vi "LCM_data_assign_tmp.vi"(9 "time-to-live":u16, 10 "Velodyne1":T3(ring), 11 "velodyne enable":bool) -> ()   [LabVIEW 2015]
uses:
  G_LCM.vi
  G_ALL.vi
  G_SEN.vi
  <vilib>/Instr/_visa.llb/VISA Configure Serial Port (Instr).vi
panel:
  out "mission_request":T1
  out "error out 3":errorcluster
  out "velodyne overflow? 2":bool
  out "VELO_RAW":T2={"hash"=6418264790525055119, "sys time"=0, "type"=0, "raw"=""} {"hash" format="%x"}
  out "ibeo overflow?":bool
  out "veodyne error out":errorcluster
  out "control input":T4
  in  "saveconfig":bool
  in  "get data":bool
  in  "parameter idx 2":u16 format="%x"
  in  "setdata":bool
  in  "Mouting":u32 format="%x"
  in  "parameter idx":u16 format="%x"
  out "LCM error":errorcluster
  out "error out":errorcluster
  out "SDT_GPS_DATA":T5
  out "PATH_T":T6
  out "length":i32
  out "ALT_T":T7={"hash"=-8920902524919788889, "sys time"=0, "u time"=0, "alt"=0.0} {"hash" format="%016x"}
  out "value":cluster{"time":i32, "alt":sgl}
  out "data":dbl[][](array[numeric]) format="%#_17g"
  out "Waveform Graph":dbl[](graph)
  out "IBEO_2202_T":T8={"hash"=-9184050406206942030, "sys time"=0, "Header"={"Size of prev messages"=0, "Size of this messages"=8534, "Reserved"=0, "DeviceID"=0, "Data type"=8706, "NTP time"=30358766255088}, "Scan header"={"Scan number"=22632, "scanner status"=811, "Sync phase offset"=0, "Scan start time NTP"=30358508796168, "Scan end time NTP"=30358603880928, "Angle ticks per rotation"=11520, "Start angle"=0.8726646259971648, "End angle"=-0.8726646259971648, "Scan points"=849, "pos_x"=0.0, "pos_y"=0.0, "pos_h"=0.0, "Mounting position x"=3.5, "Mounting position y"=0.0, "Mounting position z"=0.45, "Reserved"=5}, "Scan points"=[{"flags"=0, "Echo"=0, "Radial distance"=20.2, "Horizontal angle"=0.8552113334772213, "Vertical angle"=-0.020943951023931952, "Echo pulse width"=92, "Reserved"=0}, {"flags"=0, "Echo"=0, "Radial distance"=20.05, "Horizontal angle"=0.8552113334772213, "Vertical angle"=-0.006981317007977317, "Echo pulse width"=48, "Reserved"=0}, {"flags"=0, "Echo"=0, "Radial distance"=20.21, "Horizontal angle"=0.8464846872172498, "Vertical angle"=-0.020943951023931952, "Echo pulse width"=80, "Reserved"=0}, {"flags"=0, "Echo"=0, "Radial distance"=20.03, "Horizontal angle"=0.8464846872172498, "Vertical angle"=-0.006981317007977317, "Echo pulse width"=120, "Reserved"=0}, {"flags"=0, "Echo"=0, "Radial distance"=20.400000000000002, "Horizontal angle"=0.8377580409572781, "Vertical angle"=-0.020943951023931952, "Echo pulse width"=136, "Reserved"=0}, {"flags"=0, "Echo"=0, "Radial distance"=20.080000000000002, "Horizontal angle"=0.8377580409572781, "Vertical angle"=-0.006981317007977317, "Echo pulse width"=132, "Reserved"=0}, {"flags"=0, "Echo"=0, "Radial distance"=20.67, "Horizontal angle"=0.8290313946973066, "Vertical angle"=-0.020943951023931952, "Echo pulse width"=124, "Reserved"=0}, {"flags"=0, "Echo"=0, "Radial distance"=20.37, "Horizontal angle"=0.8290313946973066, "Vertical angle"=-0.006981317007977317, "Echo pulse width"=144, "Reserved"=0}, {"flags"=5, "Echo"=0, "Radial distance"=20.830000000000002, "Horizontal angle"=0.8203047484373349, "Vertical angle"=-0.020943951023931952, "Echo pulse width"=72, "Reserved"=0}, {"flags"=4, "Echo"=1, "Radial distance"=21.87, "Horizontal angle"=0.8203047484373349, "Vertical angle"=-0.020943951023931952, "Echo pulse width"=124, "Reserved"=0}, {"flags"=4, "Echo"=0, "Radial distance"=21.88, "Horizontal angle"=0.8115781021773633, "Vertical angle"=-0.020943951023931952, "Echo pulse width"=132, "Reserved"=0}, {"flags"=4, "Echo"=0, "Radial distance"=21.78, "Horizontal angle"=0.8028514559173915, "Vertical angle"=-0.020943951023931952, "Echo pulse width"=156, "Reserved"=0}, {"flags"=4, "Echo"=0, "Radial distance"=21.76, "Horizontal angle"=0.7941248096574199, "Vertical angle"=-0.020943951023931952, "Echo pulse width"=176, "Reserved"=0}, {"flags"=1, "Echo"=0, "Radial distance"=23.37, "Horizontal angle"=0.7941248096574199, "Vertical angle"=-0.006981317007977317, "Echo pulse width"=100, "Reserved"=1}, {"flags"=0, "Echo"=1, "Radial distance"=48.230000000000004, "Horizontal angle"=0.7941248096574199, "Vertical angle"=-0.006981317007977317, "Echo pulse width"=120, "Reserved"=2}, {"flags"=4, "Echo"=0, "Radial distance"=21.76, "Horizontal angle"=0.7853981633974483, "Vertical angle"=-0.020943951023931952, "Echo pulse width"=172, "Reserved"=0}, {"flags"=1, "Echo"=0, "Radial distance"=23.25, "Horizontal angle"=0.7853981633974483, "Vertical angle"=-0.006981317007977317, "Echo pulse width"=144, "Reserved"=1}, {"flags"=0, "Echo"=1, "Radial distance"=48.02, "Horizontal angle"=0.7853981633974483, "Vertical angle"=-0.006981317007977317, "Echo pulse width"=108, "Reserved"=2}, {"flags"=0, "Echo"=0, "Radial distance"=16.740000000000002, "Horizontal angle"=0.7766715171374766, "Vertical angle"=-0.020943951023931952, "Echo pulse width"=156, "Reserved"=3}, {"flags"=0, "Echo"=0, "Radial distance"=16.77, "Horizontal angle"=0.7766715171374766, "Vertical angle"=-0.006981317007977317, "Echo pulse width"=152, "Reserved"=3}, {"flags"=5, "Echo"=0, "Radial distance"=5.44, "Horizontal angle"=0.767944870877505, "Vertical angle"=-0.020943951023931952, "Echo pulse width"=136, "Reserved"=0}, {"flags"=4, "Echo"=1, "Radial distance"=21.87, "Horizontal angle"=0.767944870877505, "Vertical angle"=-0.020943951023931952, "Echo pulse width"=164, "Reserved"=0}, {"flags"=1, "Echo"=0, "Radial distance"=23.17, "Horizontal angle"=0.767944870877505, "Vertical angle"=-0.006981317007977317, "Echo pulse width"=148, "Reserved"=1}, {"flags"=0, "Echo"=1, "Radial distance"=48.18, "Horizontal angle"=0.767944870877505, "Vertical angle"=-0.006981317007977317, "Echo pulse width"=108, "Reserved"=4}, {"flags"=4, "Echo"=0, "Radial distance"=22.03, "Horizontal angle"=0.7592182246175333, "Vertical angle"=-0.020943951023931952, "Echo pulse width"=164, "Reserved"=0}, {"flags"=0, "Echo"=0, "Radial distance"=23.3, "Horizontal angle"=0.7592182246175333, "Vertical angle"=-0.006981317007977317, "Echo pulse width"=168, "Reserved"=1}, {"flags"=5, "Echo"=0, "Radial distance"=5.21, "Horizontal angle"=0.7504915783575618, "Vertical angle"=-0.020943951023931952, "Echo pulse width"=144, "Reserved"=0}, {"flags"=4, "Echo"=1, "Radial distance"=22.27, "Horizontal angle"=0.7504915783575618, "Vertical angle"=-0.020943951023931952, "Echo pulse width"=164, "Reserved"=0}, {"flags"=0, "Echo"=0, "Radial distance"=23.34, "Horizontal angle"=0.7504915783575618, "Vertical angle"=-0.006981317007977317, "Echo pulse width"=172, "Reserved"=1}, {"flags"=5, "Echo"=0, "Radial distance"=20.36, "Horizontal angle"=0.74176493209759, "Vertical angle"=-0.020943951023931952, "Echo pulse width"=68, "Reserved"=0}, {"flags"=4, "Echo"=1, "Radial distance"=22.42, "Horizontal angle"=0.74176493209759, "Vertical angle"=-0.020943951023931952, "Echo pulse width"=152, "Reserved"=0}, {"flags"=0, "Echo"=0, "Radial distance"=23.38, "Horizontal angle"=0.74176493209759, "Vertical angle"=-0.006981317007977317, "Echo pulse width"=168, "Reserved"=1}, {"flags"=5, "Echo"=0, "Radial distance"=5.5600000000000005, "Horizontal angle"=0.7330382858376184, "Vertical angle"=-0.020943951023931952, "Echo pulse width"=168, "Reserved"=0}, {"flags"=4, "Echo"=1, "Radial distance"=22.62, "Horizontal angle"=0.7330382858376184, "Vertical angle"=-0.020943951023931952, "Echo pulse width"=152, "Reserved"=0}, {"flags"=1, "Echo"=0, "Radial distance"=23.37, "Horizontal angle"=0.7330382858376184, "Vertical angle"=-0.006981317007977317, "Echo pulse width"=156, "Reserved"=1}, {"flags"=0, "Echo"=1, "Radial distance"=48.21, "Horizontal angle"=0.7330382858376184, "Vertical angle"=-0.006981317007977317, "Echo pulse width"=72, "Reserved"=5}, {"flags"=5, "Echo"=0, "Radial distance"=5.58, "Horizontal angle"=0.7243116395776468, "Vertical angle"=-0.020943951023931952, "Echo pulse width"=136, "Reserved"=0}, {"flags"=5, "Echo"=1, "Radial distance"=20.88, "Horizontal angle"=0.7243116395776468, "Vertical angle"=-0.020943951023931952, "Echo pulse width"=64, "Reserved"=0}, {"flags"=4, "Echo"=2, "Radial distance"=22.77, "Horizontal angle"=0.7243116395776468, "Vertical angle"=-0.020943951023931952, "Echo pulse width"=148, "Reserved"=0}, {"flags"=0, "Echo"=0, "Radial distance"=23.62, "Horizontal angle"=0.7243116395776468, "Vertical angle"=-0.006981317007977317, "Echo pulse width"=172, "Reserved"=1}, {"flags"=5, "Echo"=0, "Radial distance"=5.63, "Horizontal angle"=0.7155849933176751, "Vertical angle"=-0.020943951023931952, "Echo pulse width"=196, "Reserved"=0}, {"flags"=4, "Echo"=1, "Radial distance"=22.69, "Horizontal angle"=0.7155849933176751, "Vertical angle"=-0.020943951023931952, "Echo pulse width"=212, "Reserved"=0}, {"flags"=0, "Echo"=0, "Radial distance"=23.82, "Horizontal angle"=0.7155849933176751, "Vertical angle"=-0.006981317007977317, "Echo pulse width"=160, "Reserved"=1}, {"flags"=5, "Echo"=0, "Radial distance"=5.67, "Horizontal angle"=0.7068583470577035, "Vertical angle"=-0.020943951023931952, "Echo pulse width"=172, "Reserved"=0}, {"flags"=4, "Echo"=1, "Radial distance"=23.16, "Horizontal angle"=0.7068583470577035, "Vertical angle"=-0.020943951023931952, "Echo pulse width"=176, "Reserved"=0}, {"flags"=0, "Echo"=0, "Radial distance"=23.62, "Horizontal angle"=0.7068583470577035, "Vertical angle"=-0.006981317007977317, "Echo pulse width"=164, "Reserved"=1}, {"flags"=5, "Echo"=0, "Radial distance"=5.53, "Horizontal angle"=0.6981317007977318, "Vertical angle"=-0.020943951023931952, "Echo pulse width"=208, "Reserved"=0}, {"flags"=0, "Echo"=1, "Radial distance"=23.35, "Horizontal angle"=0.6981317007977318, "Vertical angle"=-0.020943951023931952, "Echo pulse width"=160, "Reserved"=1}, {"flags"=0, "Echo"=0, "Radial distance"=23.650000000000002, "Horizontal angle"=0.6981317007977318, "Vertical angle"=-0.006981317007977317, "Echo pulse width"=148, "Reserved"=1}, {"flags"=5, "Echo"=0, "Radial distance"=5.55, "Horizontal angle"=0.6894050545377601, "Vertical angle"=-0.020943951023931952, "Echo pulse width"=192, "Reserved"=0}, {"flags"=0, "Echo"=1, "Radial distance"=23.55, "Horizontal angle"=0.6894050545377601, "Vertical angle"=-0.020943951023931952, "Echo pulse width"=160, "Reserved"=1}, {"flags"=0, "Echo"=0, "Radial distance"=23.62, "Horizontal angle"=0.6894050545377601, "Vertical angle"=-0.006981317007977317, "Echo pulse width"=160, "Reserved"=1}, {"flags"=5, "Echo"=0, "Radial distance"=5.5600000000000005, "Horizontal angle"=0.6806784082777886, "Vertical angle"=-0.020943951023931952, "Echo pulse width"=236, "Reserved"=0}, {"flags"=0, "Echo"=1, "Radial distance"=23.77, "Horizontal angle"=0.6806784082777886, "Vertical angle"=-0.020943951023931952, "Echo pulse width"=144, "Reserved"=1}, {"flags"=0, "Echo"=0, "Radial distance"=23.61, "Horizontal angle"=0.6806784082777886, "Vertical angle"=-0.006981317007977317, "Echo pulse width"=156, "Reserved"=1}, {"flags"=5, "Echo"=0, "Radial distance"=5.5200000000000005, "Horizontal angle"=0.6719517620178168, "Vertical angle"=-0.020943951023931952, "Echo pulse width"=220, "Reserved"=0}, {"flags"=4, "Echo"=1, "Radial distance"=24.17, "Horizontal angle"=0.6719517620178168, "Vertical angle"=-0.020943951023931952, "Echo pulse width"=148, "Reserved"=0}, {"flags"=0, "Echo"=0, "Radial distance"=23.66, "Horizontal angle"=0.6719517620178168, "Vertical angle"=-0.006981317007977317, "Echo pulse width"=164, "Reserved"=1}, {"flags"=5, "Echo"=0, "Radial distance"=5.67, "Horizontal angle"=0.6632251157578453, "Vertical angle"=-0.020943951023931952, "Echo pulse width"=224, "Reserved"=0}, {"flags"=4, "Echo"=1, "Radial distance"=24.45, "Horizontal angle"=0.6632251157578453, "Vertical angle"=-0.020943951023931952, "Echo pulse width"=148, "Reserved"=0}, {"flags"=1, "Echo"=0, "Radial distance"=32.230000000000004, "Horizontal angle"=0.6632251157578453, "Vertical angle"=-0.006981317007977317, "Echo pulse width"=40, "Reserved"=6}, {"flags"=0, "Echo"=1, "Radial distance"=35.42, "Horizontal angle"=0.6632251157578453, "Vertical angle"=-0.006981317007977317, "Echo pulse width"=164, "Reserved"=7}, {"flags"=5, "Echo"=0, "Radial distance"=5.63, "Horizontal angle"=0.6544984694978736, "Vertical angle"=-0.020943951023931952, "Echo pulse width"=208, "Reserved"=0}, {"flags"=4, "Echo"=1, "Radial distance"=24.73, "Horizontal angle"=0.6544984694978736, "Vertical angle"=-0.020943951023931952, "Echo pulse width"=144, "Reserved"=0}, {"flags"=0, "Echo"=0, "Radial distance"=35.14, "Horizontal angle"=0.6544984694978736, "Vertical angle"=-0.006981317007977317, "Echo pulse width"=164, "Reserved"=7}, {"flags"=5, "Echo"=0, "Radial distance"=5.64, "Horizontal angle"=0.6457718232379019, "Vertical angle"=-0.020943951023931952, "Echo pulse width"=244, "Reserved"=0}, {"flags"=4, "Echo"=1, "Radial distance"=25.04, "Horizontal angle"=0.6457718232379019, "Vertical angle"=-0.020943951023931952, "Echo pulse width"=132, "Reserved"=0}, {"flags"=0, "Echo"=0, "Radial distance"=35.01, "Horizontal angle"=0.6457718232379019, "Vertical angle"=-0.006981317007977317, "Echo pulse width"=156, "Reserved"=7}, {"flags"=5, "Echo"=0, "Radial distance"=5.71, "Horizontal angle"=0.6370451769779303, "Vertical angle"=-0.020943951023931952, "Echo pulse width"=264, "Reserved"=0}, {"flags"=4, "Echo"=1, "Radial distance"=25.6, "Horizontal angle"=0.6370451769779303, "Vertical angle"=-0.020943951023931952, "Echo pulse width"=132, "Reserved"=0}, {"flags"=1, "Echo"=0, "Radial distance"=32.68, "Horizontal angle"=0.6370451769779303, "Vertical angle"=-0.006981317007977317, "Echo pulse width"=56, "Reserved"=8}, {"flags"=0, "Echo"=1, "Radial distance"=34.86, "Horizontal angle"=0.6370451769779303, "Vertical angle"=-0.006981317007977317, "Echo pulse width"=160, "Reserved"=7}, {"flags"=5, "Echo"=0, "Radial distance"=5.63, "Horizontal angle"=0.6283185307179586, "Vertical angle"=-0.020943951023931952, "Echo pulse width"=296, "Reserved"=0}, {"flags"=4, "Echo"=1, "Radial distance"=25.84, "Horizontal angle"=0.6283185307179586, "Vertical angle"=-0.020943951023931952, "Echo pulse width"=92, "Reserved"=0}, {"flags"=5, "Echo"=0, "Radial distance"=7.54, "Horizontal angle"=0.6283185307179586, "Vertical angle"=-0.006981317007977317, "Echo pulse width"=168, "Reserved"=0}, {"flags"=0, "Echo"=1, "Radial distance"=34.87, "Horizontal angle"=0.6283185307179586, "Vertical angle"=-0.006981317007977317, "Echo pulse width"=124, "Reserved"=7}, {"flags"=4, "Echo"=0, "Radial distance"=5.67, "Horizontal angle"=0.619591884457987, "Vertical angle"=-0.020943951023931952, "Echo pulse width"=272, "Reserved"=0}, {"flags"=4, "Echo"=0, "Radial distance"=7.38, "Horizontal angle"=0.619591884457987, "Vertical angle"=-0.006981317007977317, "Echo pulse width"=204, "Reserved"=0}, {"flags"=4, "Echo"=0, "Radial distance"=5.67, "Horizontal angle"=0.6108652381980153, "Vertical angle"=-0.020943951023931952, "Echo pulse width"=284, "Reserved"=0}, {"flags"=0, "Echo"=0, "Radial distance"=7.33, "Horizontal angle"=0.6108652381980153, "Vertical angle"=-0.006981317007977317, "Echo pulse width"=224, "Reserved"=9}, {"flags"=0, "Echo"=0, "Radial distance"=7.21, "Horizontal angle"=0.6065019150680295, "Vertical angle"=0.00698131700797732, "Echo pulse width"=124, "Reserved"=9}, {"flags"=0, "Echo"=0, "Radial distance"=7.08, "Horizontal angle"=0.6065019150680295, "Vertical angle"=0.020943951023931963, "Echo pulse width"=120, "Reserved"=9}, {"flags"=4, "Echo"=0, "Radial distance"=5.79, "Horizontal angle"=0.6021385919380438, "Vertical angle"=-0.020943951023931952, "Echo pulse width"=248, "Reserved"=0}, {"flags"=0, "Echo"=0, "Radial distance"=7.09, "Horizontal angle"=0.6021385919380438, "Vertical angle"=-0.006981317007977317, "Echo pulse width"=232, "Reserved"=9}, {"flags"=0, "Echo"=0, "Radial distance"=7.24, "Horizontal angle"=0.5977752688080579, "Vertical angle"=0.00698131700797732, "Echo pulse width"=72, "Reserved"=9}, {"flags"=0, "Echo"=0, "Radial distance"=6.99, "Horizontal angle"=0.5977752688080579, "Vertical angle"=0.020943951023931963, "Echo pulse width"=60, "Reserved"=9}, {"flags"=4, "Echo"=0, "Radial distance"=5.75, "Horizontal angle"=0.593411945678072, "Vertical angle"=-0.020943951023931952, "Echo pulse width"=268, "Reserved"=0}, {"flags"=0, "Echo"=0, "Radial distance"=6.84, "Horizontal angle"=0.593411945678072, "Vertical angle"=-0.006981317007977317, "Echo pulse width"=284, "Reserved"=9}, {"flags"=0, "Echo"=0, "Radial distance"=7.140000000000001, "Horizontal angle"=0.5890486225480862, "Vertical angle"=0.00698131700797732, "Echo pulse width"=160, "Reserved"=9}, {"flags"=0, "Echo"=0, "Radial distance"=6.98, "Horizontal angle"=0.5890486225480862, "Vertical angle"=0.020943951023931963, "Echo pulse width"=144, "Reserved"=9}, {"flags"=4, "Echo"=0, "Radial distance"=5.79, "Horizontal angle"=0.5846852994181004, "Vertical angle"=-0.020943951023931952, "Echo pulse width"=236, "Reserved"=0}, {"flags"=0, "Echo"=0, "Radial distance"=6.95, "Horizontal angle"=0.5846852994181004, "Vertical angle"=-0.006981317007977317, "Echo pulse width"=264, "Reserved"=9}, {"flags"=0, "Echo"=0, "Radial distance"=7.03, "Horizontal angle"=0.5803219762881145, "Vertical angle"=0.00698131700797732, "Echo pulse width"=112, "Reserved"=9}, {"flags"=0, "Echo"=0, "Radial distance"=6.8, "Horizontal angle"=0.5803219762881145, "Vertical angle"=0.020943951023931963, "Echo pulse width"=104, "Reserved"=9}, {"flags"=4, "Echo"=0, "Radial distance"=5.67, "Horizontal angle"=0.5759586531581287, "Vertical angle"=-0.020943951023931952, "Echo pulse width"=268, "Reserved"=0}, {"flags"=0, "Echo"=0, "Radial distance"=6.76, "Horizontal angle"=0.5759586531581287, "Vertical angle"=-0.006981317007977317, "Echo pulse width"=288, "Reserved"=9}, {"flags"=0, "Echo"=0, "Radial distance"=7.0200000000000005, "Horizontal angle"=0.5715953300281429, "Vertical angle"=0.00698131700797732, "Echo pulse width"=168, "Reserved"=9}, {"flags"=0, "Echo"=0, "Radial distance"=6.91, "Horizontal angle"=0.5715953300281429, "Vertical angle"=0.020943951023931963, "Echo pulse width"=156, "Reserved"=9}, {"flags"=4, "Echo"=0, "Radial distance"=5.76, "Horizontal angle"=0.5672320068981571, "Vertical angle"=-0.020943951023931952, "Echo pulse width"=216, "Reserved"=0}, {"flags"=0, "Echo"=0, "Radial distance"=6.71, "Horizontal angle"=0.5672320068981571, "Vertical angle"=-0.006981317007977317, "Echo pulse width"=264, "Reserved"=9}, {"flags"=0, "Echo"=0, "Radial distance"=7.08, "Horizontal angle"=0.5628686837681712, "Vertical angle"=0.00698131700797732, "Echo pulse width"=136, "Reserved"=9}, {"flags"=0, "Echo"=0, "Radial distance"=6.8100000000000005, "Horizontal angle"=0.5628686837681712, "Vertical angle"=0.020943951023931963, "Echo pulse width"=112, "Reserved"=9}, {"flags"=4, "Echo"=0, "Radial distance"=5.79, "Horizontal angle"=0.5585053606381855, "Vertical angle"=-0.020943951023931952, "Echo pulse width"=248, "Reserved"=0}, {"flags"=0, "Echo"=0, "Radial distance"=6.6000000000000005, "Horizontal angle"=0.5585053606381855, "Vertical angle"=-0.006981317007977317, "Echo pulse width"=256, "Reserved"=9}, {"flags"=0, "Echo"=0, "Radial distance"=6.95, "Horizontal angle"=0.5541420375081997, "Vertical angle"=0.00698131700797732, "Echo pulse width"=176, "Reserved"=9}, {"flags"=0, "Echo"=0, "Radial distance"=6.75, "Horizontal angle"=0.5541420375081997, "Vertical angle"=0.020943951023931963, "Echo pulse width"=160, "Reserved"=9}, {"flags"=4, "Echo"=0, "Radial distance"=5.8100000000000005, "Horizontal angle"=0.5497787143782138, "Vertical angle"=-0.020943951023931952, "Echo pulse width"=204, "Reserved"=0}, {"flags"=0, "Echo"=0, "Radial distance"=6.61, "Horizontal angle"=0.5497787143782138, "Vertical angle"=-0.006981317007977317, "Echo pulse width"=224, "Reserved"=9}, {"flags"=0, "Echo"=0, "Radial distance"=6.88, "Horizontal angle"=0.5454153912482279, "Vertical angle"=0.00698131700797732, "Echo pulse width"=140, "Reserved"=9}, {"flags"=0, "Echo"=0, "Radial distance"=6.65, "Horizontal angle"=0.5454153912482279, "Vertical angle"=0.020943951023931963, "Echo pulse width"=124, "Reserved"=9}, {"flags"=4, "Echo"=0, "Radial distance"=5.8, "Horizontal angle"=0.5410520681182421, "Vertical angle"=-0.020943951023931952, "Echo pulse width"=232, "Reserved"=0}, {"flags"=0, "Echo"=0, "Radial distance"=6.65, "Horizontal angle"=0.5410520681182421, "Vertical angle"=-0.006981317007977317, "Echo pulse width"=232, "Reserved"=9}, {"flags"=0, "Echo"=0, "Radial distance"=6.91, "Horizontal angle"=0.5366887449882564, "Vertical angle"=0.00698131700797732, "Echo pulse width"=192, "Reserved"=9}, {"flags"=0, "Echo"=0, "Radial distance"=6.67, "Horizontal angle"=0.5366887449882564, "Vertical angle"=0.020943951023931963, "Echo pulse width"=160, "Reserved"=9}, {"flags"=4, "Echo"=0, "Radial distance"=5.91, "Horizontal angle"=0.5323254218582705, "Vertical angle"=-0.020943951023931952, "Echo pulse width"=196, "Reserved"=0}, {"flags"=0, "Echo"=0, "Radial distance"=6.7, "Horizontal angle"=0.5323254218582705, "Vertical angle"=-0.006981317007977317, "Echo pulse width"=200, "Reserved"=9}, {"flags"=0, "Echo"=0, "Radial distance"=6.72, "Horizontal angle"=0.5279620987282847, "Vertical angle"=0.00698131700797732, "Echo pulse width"=136, "Reserved"=9}, {"flags"=0, "Echo"=0, "Radial distance"=6.66, "Horizontal angle"=0.5279620987282847, "Vertical angle"=0.020943951023931963, "Echo pulse width"=144, "Reserved"=9}, {"flags"=4, "Echo"=0, "Radial distance"=5.91, "Horizontal angle"=0.5235987755982988, "Vertical angle"=-0.020943951023931952, "Echo pulse width"=224, "Reserved"=0}, {"flags"=0, "Echo"=0, "Radial distance"=6.72, "Horizontal angle"=0.5235987755982988, "Vertical angle"=-0.006981317007977317, "Echo pulse width"=220, "Reserved"=9}, {"flags"=0, "Echo"=0, "Radial distance"=6.87, "Horizontal angle"=0.519235452468313, "Vertical angle"=0.00698131700797732, "Echo pulse width"=180, "Reserved"=9}, {"flags"=0, "Echo"=0, "Radial distance"=6.68, "Horizontal angle"=0.519235452468313, "Vertical angle"=0.020943951023931963, "Echo pulse width"=180, "Reserved"=9}, {"flags"=4, "Echo"=0, "Radial distance"=6.03, "Horizontal angle"=0.5148721293383272, "Vertical angle"=-0.020943951023931952, "Echo pulse width"=192, "Reserved"=0}, {"flags"=0, "Echo"=0, "Radial distance"=6.68, "Horizontal angle"=0.5148721293383272, "Vertical angle"=-0.006981317007977317, "Echo pulse width"=208, "Reserved"=9}, {"flags"=0, "Echo"=0, "Radial distance"=7.01, "Horizontal angle"=0.5105088062083414, "Vertical angle"=0.00698131700797732, "Echo pulse width"=176, "Reserved"=9}, {"flags"=0, "Echo"=0, "Radial distance"=6.62, "Horizontal angle"=0.5105088062083414, "Vertical angle"=0.020943951023931963, "Echo pulse width"=148, "Reserved"=9}, {"flags"=4, "Echo"=0, "Radial distance"=5.99, "Horizontal angle"=0.5061454830783556, "Vertical angle"=-0.020943951023931952, "Echo pulse width"=216, "Reserved"=0}, {"flags"=0, "Echo"=0, "Radial distance"=6.6000000000000005, "Horizontal angle"=0.5061454830783556, "Vertical angle"=-0.006981317007977317, "Echo pulse width"=220, "Reserved"=9}, {"flags"=0, "Echo"=0, "Radial distance"=6.82, "Horizontal angle"=0.5017821599483697, "Vertical angle"=0.00698131700797732, "Echo pulse width"=200, "Reserved"=9}, {"flags"=0, "Echo"=0, "Radial distance"=6.640000000000001, "Horizontal angle"=0.5017821599483697, "Vertical angle"=0.020943951023931963, "Echo pulse width"=180, "Reserved"=9}, {"flags"=4, "Echo"=0, "Radial distance"=6.09, "Horizontal angle"=0.4974188368183839, "Vertical angle"=-0.020943951023931952, "Echo pulse width"=188, "Reserved"=0}, {"flags"=0, "Echo"=0, "Radial distance"=6.66, "Horizontal angle"=0.4974188368183839, "Vertical angle"=-0.006981317007977317, "Echo pulse width"=204, "Reserved"=9}, {"flags"=0, "Echo"=0, "Radial distance"=6.79, "Horizontal angle"=0.49305551368839806, "Vertical angle"=0.00698131700797732, "Echo pulse width"=160, "Reserved"=9}, {"flags"=0, "Echo"=0, "Radial distance"=6.59, "Horizontal angle"=0.49305551368839806, "Vertical angle"=0.020943951023931963, "Echo pulse width"=160, "Reserved"=9}, {"flags"=4, "Echo"=0, "Radial distance"=6.15, "Horizontal angle"=0.4886921905584123, "Vertical angle"=-0.020943951023931952, "Echo pulse width"=216, "Reserved"=0}, {"flags"=0, "Echo"=0, "Radial distance"=6.71, "Horizontal angle"=0.4886921905584123, "Vertical angle"=-0.006981317007977317, "Echo pulse width"=200, "Reserved"=9}, {"flags"=0, "Echo"=0, "Radial distance"=6.6000000000000005, "Horizontal angle"=0.48432886742842646, "Vertical angle"=0.00698131700797732, "Echo pulse width"=184, "Reserved"=9}, {"flags"=0, "Echo"=0, "Radial distance"=6.5200000000000005, "Horizontal angle"=0.48432886742842646, "Vertical angle"=0.020943951023931963, "Echo pulse width"=176, "Reserved"=9}, {"flags"=4, "Echo"=0, "Radial distance"=6.15, "Horizontal angle"=0.4799655442984406, "Vertical angle"=-0.020943951023931952, "Echo pulse width"=196, "Reserved"=0}, {"flags"=0, "Echo"=0, "Radial distance"=6.72, "Horizontal angle"=0.4799655442984406, "Vertical angle"=-0.006981317007977317, "Echo pulse width"=184, "Reserved"=9}, {"flags"=0, "Echo"=0, "Radial distance"=6.71, "Horizontal angle"=0.47560222116845474, "Vertical angle"=0.00698131700797732, "Echo pulse width"=184, "Reserved"=9}, {"flags"=0, "Echo"=0, "Radial distance"=6.63, "Horizontal angle"=0.47560222116845474, "Vertical angle"=0.020943951023931963, "Echo pulse width"=168, "Reserved"=9}, {"flags"=4, "Echo"=0, "Radial distance"=6.15, "Horizontal angle"=0.47123889803846897, "Vertical angle"=-0.020943951023931952, "Echo pulse width"=224, "Reserved"=0}, {"flags"=0, "Echo"=0, "Radial distance"=6.68, "Horizontal angle"=0.47123889803846897, "Vertical angle"=-0.006981317007977317, "Echo pulse width"=196, "Reserved"=9}, {"flags"=0, "Echo"=0, "Radial distance"=6.6000000000000005, "Horizontal angle"=0.46687557490848314, "Vertical angle"=0.00698131700797732, "Echo pulse width"=188, "Reserved"=9}, {"flags"=0, "Echo"=0, "Radial distance"=6.6000000000000005, "Horizontal angle"=0.46687557490848314, "Vertical angle"=0.020943951023931963, "Echo pulse width"=196, "Reserved"=9}, {"flags"=4, "Echo"=0, "Radial distance"=6.13, "Horizontal angle"=0.4625122517784973, "Vertical angle"=-0.020943951023931952, "Echo pulse width"=204, "Reserved"=0}, {"flags"=0, "Echo"=0, "Radial distance"=6.63, "Horizontal angle"=0.4625122517784973, "Vertical angle"=-0.006981317007977317, "Echo pulse width"=192, "Reserved"=9}, {"flags"=0, "Echo"=0, "Radial distance"=6.57, "Horizontal angle"=0.45814892864851153, "Vertical angle"=0.00698131700797732, "Echo pulse width"=172, "Reserved"=9}, {"flags"=0, "Echo"=0, "Radial distance"=6.63, "Horizontal angle"=0.45814892864851153, "Vertical angle"=0.020943951023931963, "Echo pulse width"=180, "Reserved"=9}, {"flags"=4, "Echo"=0, "Radial distance"=6.3100000000000005, "Horizontal angle"=0.45378560551852565, "Vertical angle"=-0.020943951023931952, "Echo pulse width"=220, "Reserved"=0}, {"flags"=0, "Echo"=0, "Radial distance"=6.67, "Horizontal angle"=0.45378560551852565, "Vertical angle"=-0.006981317007977317, "Echo pulse width"=200, "Reserved"=9}, {"flags"=0, "Echo"=0, "Radial distance"=6.63, "Horizontal angle"=0.4494222823885398, "Vertical angle"=0.00698131700797732, "Echo pulse width"=192, "Reserved"=9}, {"flags"=0, "Echo"=0, "Radial distance"=6.49, "Horizontal angle"=0.4494222823885398, "Vertical angle"=0.020943951023931963, "Echo pulse width"=184, "Reserved"=9}, {"flags"=4, "Echo"=0, "Radial distance"=6.2700000000000005, "Horizontal angle"=0.445058959258554, "Vertical angle"=-0.020943951023931952, "Echo pulse width"=196, "Reserved"=0}, {"flags"=0, "Echo"=0, "Radial distance"=6.59, "Horizontal angle"=0.445058959258554, "Vertical angle"=-0.006981317007977317, "Echo pulse width"=196, "Reserved"=9}, {"flags"=0, "Echo"=0, "Radial distance"=6.53, "Horizontal angle"=0.4406956361285682, "Vertical angle"=0.00698131700797732, "Echo pulse width"=172, "Reserved"=9}, {"flags"=0, "Echo"=0, "Radial distance"=6.51, "Horizontal angle"=0.4406956361285682, "Vertical angle"=0.020943951023931963, "Echo pulse width"=172, "Reserved"=9}, {"flags"=4, "Echo"=0, "Radial distance"=6.3500000000000005, "Horizontal angle"=0.4363323129985824, "Vertical angle"=-0.020943951023931952, "Echo pulse width"=220, "Reserved"=0}, {"flags"=0, "Echo"=0, "Radial distance"=6.67, "Horizontal angle"=0.4363323129985824, "Vertical angle"=-0.006981317007977317, "Echo pulse width"=204, "Reserved"=9}, {"flags"=0, "Echo"=0, "Radial distance"=6.5600000000000005, "Horizontal angle"=0.4319689898685966, "Vertical angle"=0.00698131700797732, "Echo pulse width"=188, "Reserved"=9}, {"flags"=0, "Echo"=0, "Radial distance"=6.5200000000000005, "Horizontal angle"=0.4319689898685966, "Vertical angle"=0.020943951023931963, "Echo pulse width"=192, "Reserved"=9}, {"flags"=0, "Echo"=0, "Radial distance"=6.390000000000001, "Horizontal angle"=0.42760566673861067, "Vertical angle"=-0.020943951023931952, "Echo pulse width"=192, "Reserved"=9}, {"flags"=0, "Echo"=0, "Radial distance"=6.71, "Horizontal angle"=0.42760566673861067, "Vertical angle"=-0.006981317007977317, "Echo pulse width"=192, "Reserved"=9}, {"flags"=0, "Echo"=0, "Radial distance"=6.49, "Horizontal angle"=0.4232423436086249, "Vertical angle"=0.00698131700797732, "Echo pulse width"=168, "Reserved"=9}, {"flags"=0, "Echo"=0, "Radial distance"=6.51, "Horizontal angle"=0.4232423436086249, "Vertical angle"=0.020943951023931963, "Echo pulse width"=168, "Reserved"=9}, {"flags"=0, "Echo"=0, "Radial distance"=6.41, "Horizontal angle"=0.41887902047863906, "Vertical angle"=-0.020943951023931952, "Echo pulse width"=212, "Reserved"=9}, {"flags"=0, "Echo"=0, "Radial distance"=6.76, "Horizontal angle"=0.41887902047863906, "Vertical angle"=-0.006981317007977317, "Echo pulse width"=216, "Reserved"=9}, {"flags"=0, "Echo"=0, "Radial distance"=6.66, "Horizontal angle"=0.4145156973486533, "Vertical angle"=0.00698131700797732, "Echo pulse width"=204, "Reserved"=9}, {"flags"=0, "Echo"=0, "Radial distance"=6.49, "Horizontal angle"=0.4145156973486533, "Vertical angle"=0.020943951023931963, "Echo pulse width"=188, "Reserved"=9}, {"flags"=0, "Echo"=0, "Radial distance"=6.47, "Horizontal angle"=0.41015237421866746, "Vertical angle"=-0.020943951023931952, "Echo pulse width"=180, "Reserved"=9}, {"flags"=0, "Echo"=0, "Radial distance"=6.71, "Horizontal angle"=0.41015237421866746, "Vertical angle"=-0.006981317007977317, "Echo pulse width"=192, "Reserved"=9}, {"flags"=0, "Echo"=0, "Radial distance"=6.69, "Horizontal angle"=0.40578905108868163, "Vertical angle"=0.00698131700797732, "Echo pulse width"=176, "Reserved"=9}, {"flags"=0, "Echo"=0, "Radial distance"=6.51, "Horizontal angle"=0.40578905108868163, "Vertical angle"=0.020943951023931963, "Echo pulse width"=176, "Reserved"=9}, {"flags"=0, "Echo"=0, "Radial distance"=6.53, "Horizontal angle"=0.40142572795869574, "Vertical angle"=-0.020943951023931952, "Echo pulse width"=208, "Reserved"=9}, {"flags"=0, "Echo"=0, "Radial distance"=6.71, "Horizontal angle"=0.40142572795869574, "Vertical angle"=-0.006981317007977317, "Echo pulse width"=200, "Reserved"=9}, {"flags"=0, "Echo"=0, "Radial distance"=6.79, "Horizontal angle"=0.39706240482870997, "Vertical angle"=0.00698131700797732, "Echo pulse width"=220, "Reserved"=9}, {"flags"=0, "Echo"=0, "Radial distance"=6.72, "Horizontal angle"=0.39706240482870997, "Vertical angle"=0.020943951023931963, "Echo pulse width"=220, "Reserved"=9}, {"flags"=0, "Echo"=0, "Radial distance"=6.61, "Horizontal angle"=0.39269908169872414, "Vertical angle"=-0.020943951023931952, "Echo pulse width"=184, "Reserved"=9}, {"flags"=0, "Echo"=0, "Radial distance"=6.74, "Horizontal angle"=0.39269908169872414, "Vertical angle"=-0.006981317007977317, "Echo pulse width"=176, "Reserved"=9}, {"flags"=0, "Echo"=0, "Radial distance"=6.69, "Horizontal angle"=0.3883357585687383, "Vertical angle"=0.00698131700797732, "Echo pulse width"=172, "Reserved"=9}, {"flags"=0, "Echo"=0, "Radial distance"=6.59, "Horizontal angle"=0.3883357585687383, "Vertical angle"=0.020943951023931963, "Echo pulse width"=160, "Reserved"=9}, {"flags"=0, "Echo"=0, "Radial distance"=6.63, "Horizontal angle"=0.3839724354387525, "Vertical angle"=-0.020943951023931952, "Echo pulse width"=216, "Reserved"=9}, {"flags"=0, "Echo"=0, "Radial distance"=6.74, "Horizontal angle"=0.3839724354387525, "Vertical angle"=-0.006981317007977317, "Echo pulse width"=208, "Reserved"=9}, {"flags"=0, "Echo"=0, "Radial distance"=6.84, "Horizontal angle"=0.37960911230876665, "Vertical angle"=0.00698131700797732, "Echo pulse width"=208, "Reserved"=9}, {"flags"=0, "Echo"=0, "Radial distance"=6.640000000000001, "Horizontal angle"=0.37960911230876665, "Vertical angle"=0.020943951023931963, "Echo pulse width"=200, "Reserved"=9}, {"flags"=0, "Echo"=0, "Radial distance"=6.67, "Horizontal angle"=0.3752457891787809, "Vertical angle"=-0.020943951023931952, "Echo pulse width"=180, "Reserved"=9}, {"flags"=0, "Echo"=0, "Radial distance"=6.67, "Horizontal angle"=0.3752457891787809, "Vertical angle"=-0.006981317007977317, "Echo pulse width"=196, "Reserved"=9}, {"flags"=0, "Echo"=0, "Radial distance"=6.69, "Horizontal angle"=0.370882466048795, "Vertical angle"=0.00698131700797732, "Echo pulse width"=172, "Reserved"=9}, {"flags"=0, "Echo"=0, "Radial distance"=6.67, "Horizontal angle"=0.370882466048795, "Vertical angle"=0.020943951023931963, "Echo pulse width"=172, "Reserved"=9}, {"flags"=0, "Echo"=0, "Radial distance"=6.84, "Horizontal angle"=0.3665191429188092, "Vertical angle"=-0.020943951023931952, "Echo pulse width"=236, "Reserved"=9}, {"flags"=0, "Echo"=0, "Radial distance"=6.84, "Horizontal angle"=0.3665191429188092, "Vertical angle"=-0.006981317007977317, "Echo pulse width"=276, "Reserved"=9}, {"flags"=0, "Echo"=0, "Radial distance"=6.95, "Horizontal angle"=0.3621558197888234, "Vertical angle"=0.00698131700797732, "Echo pulse width"=220, "Reserved"=9}, {"flags"=0, "Echo"=0, "Radial distance"=6.76, "Horizontal angle"=0.3621558197888234, "Vertical angle"=0.020943951023931963, "Echo pulse width"=196, "Reserved"=9}, {"flags"=0, "Echo"=0, "Radial distance"=6.87, "Horizontal angle"=0.35779249665883756, "Vertical angle"=-0.020943951023931952, "Echo pulse width"=192, "Reserved"=9}, {"flags"=0, "Echo"=0, "Radial distance"=7.05, "Horizontal angle"=0.35779249665883756, "Vertical angle"=-0.006981317007977317, "Echo pulse width"=236, "Reserved"=9}, {"flags"=0, "Echo"=0, "Radial distance"=6.8100000000000005, "Horizontal angle"=0.3534291735288517, "Vertical angle"=0.00698131700797732, "Echo pulse width"=168, "Reserved"=9}, {"flags"=0, "Echo"=0, "Radial distance"=6.79, "Horizontal angle"=0.3534291735288517, "Vertical angle"=0.020943951023931963, "Echo pulse width"=168, "Reserved"=9}, {"flags"=0, "Echo"=0, "Radial distance"=6.95, "Horizontal angle"=0.3490658503988659, "Vertical angle"=-0.020943951023931952, "Echo pulse width"=192, "Reserved"=9}, {"flags"=0, "Echo"=0, "Radial distance"=7.04, "Horizontal angle"=0.3490658503988659, "Vertical angle"=-0.006981317007977317, "Echo pulse width"=284, "Reserved"=9}, {"flags"=0, "Echo"=0, "Radial distance"=7.07, "Horizontal angle"=0.34470252726888007, "Vertical angle"=0.00698131700797732, "Echo pulse width"=252, "Reserved"=9}, {"flags"=0, "Echo"=0, "Radial distance"=6.98, "Horizontal angle"=0.34470252726888007, "Vertical angle"=0.020943951023931963, "Echo pulse width"=212, "Reserved"=9}, {"flags"=0, "Echo"=0, "Radial distance"=7.11, "Horizontal angle"=0.3403392041388943, "Vertical angle"=-0.020943951023931952, "Echo pulse width"=176, "Reserved"=9}, {"flags"=0, "Echo"=0, "Radial distance"=7.140000000000001, "Horizontal angle"=0.3403392041388943, "Vertical angle"=-0.006981317007977317, "Echo pulse width"=252, "Reserved"=9}, {"flags"=0, "Echo"=0, "Radial distance"=7.0200000000000005, "Horizontal angle"=0.3359758810089084, "Vertical angle"=0.00698131700797732, "Echo pulse width"=196, "Reserved"=9}, {"flags"=0, "Echo"=0, "Radial distance"=6.95, "Horizontal angle"=0.3359758810089084, "Vertical angle"=0.020943951023931963, "Echo pulse width"=176, "Reserved"=9}, {"flags"=0, "Echo"=0, "Radial distance"=7.23, "Horizontal angle"=0.33161255787892263, "Vertical angle"=-0.020943951023931952, "Echo pulse width"=268, "Reserved"=9}, {"flags"=0, "Echo"=0, "Radial distance"=7.28, "Horizontal angle"=0.33161255787892263, "Vertical angle"=-0.006981317007977317, "Echo pulse width"=284, "Reserved"=9}, {"flags"=0, "Echo"=0, "Radial distance"=7.2700000000000005, "Horizontal angle"=0.3272492347489368, "Vertical angle"=0.00698131700797732, "Echo pulse width"=276, "Reserved"=9}, {"flags"=0, "Echo"=0, "Radial distance"=7.16, "Horizontal angle"=0.3272492347489368, "Vertical angle"=0.020943951023931963, "Echo pulse width"=204, "Reserved"=9}, {"flags"=0, "Echo"=0, "Radial distance"=7.59, "Horizontal angle"=0.32288591161895097, "Vertical angle"=-0.020943951023931952, "Echo pulse width"=232, "Reserved"=9}, {"flags"=0, "Echo"=0, "Radial distance"=7.69, "Horizontal angle"=0.32288591161895097, "Vertical angle"=-0.006981317007977317, "Echo pulse width"=232, "Reserved"=9}, {"flags"=0, "Echo"=0, "Radial distance"=7.53, "Horizontal angle"=0.31852258848896514, "Vertical angle"=0.00698131700797732, "Echo pulse width"=172, "Reserved"=9}, {"flags"=0, "Echo"=0, "Radial distance"=7.41, "Horizontal angle"=0.31852258848896514, "Vertical angle"=0.020943951023931963, "Echo pulse width"=184, "Reserved"=9}, {"flags"=0, "Echo"=0, "Radial distance"=7.3500000000000005, "Horizontal angle"=0.3141592653589793, "Vertical angle"=-0.020943951023931952, "Echo pulse width"=300, "Reserved"=9}, {"flags"=0, "Echo"=0, "Radial distance"=7.68, "Horizontal angle"=0.3141592653589793, "Vertical angle"=-0.006981317007977317, "Echo pulse width"=264, "Reserved"=9}, {"flags"=0, "Echo"=0, "Radial distance"=7.58, "Horizontal angle"=0.3097959422289935, "Vertical angle"=0.00698131700797732, "Echo pulse width"=204, "Reserved"=9}, {"flags"=0, "Echo"=0, "Radial distance"=7.48, "Horizontal angle"=0.3097959422289935, "Vertical angle"=0.020943951023931963, "Echo pulse width"=192, "Reserved"=9}, {"flags"=0, "Echo"=0, "Radial distance"=7.47, "Horizontal angle"=0.30543261909900765, "Vertical angle"=-0.020943951023931952, "Echo pulse width"=260, "Reserved"=9}, {"flags"=0, "Echo"=0, "Radial distance"=7.8100000000000005, "Horizontal angle"=0.30543261909900765, "Vertical angle"=-0.006981317007977317, "Echo pulse width"=232, "Reserved"=9}, {"flags"=0, "Echo"=0, "Radial distance"=7.63, "Horizontal angle"=0.3010692959690219, "Vertical angle"=0.00698131700797732, "Echo pulse width"=164, "Reserved"=9}, {"flags"=0, "Echo"=0, "Radial distance"=7.59, "Horizontal angle"=0.3010692959690219, "Vertical angle"=0.020943951023931963, "Echo pulse width"=172, "Reserved"=9}, {"flags"=0, "Echo"=0, "Radial distance"=7.55, "Horizontal angle"=0.296705972839036, "Vertical angle"=-0.020943951023931952, "Echo pulse width"=300, "Reserved"=9}, {"flags"=0, "Echo"=0, "Radial distance"=7.96, "Horizontal angle"=0.296705972839036, "Vertical angle"=-0.006981317007977317, "Echo pulse width"=264, "Reserved"=9}, {"flags"=0, "Echo"=0, "Radial distance"=7.97, "Horizontal angle"=0.2923426497090502, "Vertical angle"=0.00698131700797732, "Echo pulse width"=236, "Reserved"=9}, {"flags"=0, "Echo"=0, "Radial distance"=7.82, "Horizontal angle"=0.2923426497090502, "Vertical angle"=0.020943951023931963, "Echo pulse width"=212, "Reserved"=9}, {"flags"=0, "Echo"=0, "Radial distance"=8.45, "Horizontal angle"=0.28797932657906433, "Vertical angle"=-0.020943951023931952, "Echo pulse width"=204, "Reserved"=9}, {"flags"=0, "Echo"=0, "Radial distance"=8.17, "Horizontal angle"=0.28797932657906433, "Vertical angle"=-0.006981317007977317, "Echo pulse width"=236, "Reserved"=9}, {"flags"=0, "Echo"=0, "Radial distance"=8.15, "Horizontal angle"=0.28361600344907856, "Vertical angle"=0.00698131700797732, "Echo pulse width"=184, "Reserved"=9}, {"flags"=0, "Echo"=0, "Radial distance"=7.95, "Horizontal angle"=0.28361600344907856, "Vertical angle"=0.020943951023931963, "Echo pulse width"=172, "Reserved"=9}, {"flags"=0, "Echo"=0, "Radial distance"=8.56, "Horizontal angle"=0.2792526803190927, "Vertical angle"=-0.020943951023931952, "Echo pulse width"=232, "Reserved"=9}, {"flags"=0, "Echo"=0, "Radial distance"=8.4, "Horizontal angle"=0.2792526803190927, "Vertical angle"=-0.006981317007977317, "Echo pulse width"=264, "Reserved"=9}, {"flags"=0, "Echo"=0, "Radial distance"=8.23, "Horizontal angle"=0.2748893571891069, "Vertical angle"=0.00698131700797732, "Echo pulse width"=192, "Reserved"=9}, {"flags"=0, "Echo"=0, "Radial distance"=8.2, "Horizontal angle"=0.2748893571891069, "Vertical angle"=0.020943951023931963, "Echo pulse width"=192, "Reserved"=9}, {"flags"=0, "Echo"=0, "Radial distance"=8.700000000000001, "Horizontal angle"=0.27052603405912107, "Vertical angle"=-0.020943951023931952, "Echo pulse width"=224, "Reserved"=9}, {"flags"=0, "Echo"=0, "Radial distance"=8.61, "Horizontal angle"=0.27052603405912107, "Vertical angle"=-0.006981317007977317, "Echo pulse width"=220, "Reserved"=9}, {"flags"=0, "Echo"=0, "Radial distance"=8.49, "Horizontal angle"=0.26616271092913524, "Vertical angle"=0.00698131700797732, "Echo pulse width"=176, "Reserved"=9}, {"flags"=0, "Echo"=0, "Radial distance"=8.43, "Horizontal angle"=0.26616271092913524, "Vertical angle"=0.020943951023931963, "Echo pulse width"=176, "Reserved"=9}, {"flags"=0, "Echo"=0, "Radial distance"=8.71, "Horizontal angle"=0.2617993877991494, "Vertical angle"=-0.020943951023931952, "Echo pulse width"=260, "Reserved"=9}, {"flags"=0, "Echo"=0, "Radial distance"=8.700000000000001, "Horizontal angle"=0.2617993877991494, "Vertical angle"=-0.006981317007977317, "Echo pulse width"=248, "Reserved"=9}, {"flags"=0, "Echo"=0, "Radial distance"=8.71, "Horizontal angle"=0.2574360646691636, "Vertical angle"=0.00698131700797732, "Echo pulse width"=196, "Reserved"=9}, {"flags"=0, "Echo"=0, "Radial distance"=8.68, "Horizontal angle"=0.2574360646691636, "Vertical angle"=0.020943951023931963, "Echo pulse width"=216, "Reserved"=9}, {"flags"=0, "Echo"=0, "Radial distance"=9.11, "Horizontal angle"=0.2530727415391778, "Vertical angle"=-0.020943951023931952, "Echo pulse width"=208, "Reserved"=9}, {"flags"=0, "Echo"=0, "Radial distance"=8.94, "Horizontal angle"=0.2530727415391778, "Vertical angle"=-0.006981317007977317, "Echo pulse width"=200, "Reserved"=9}, {"flags"=0, "Echo"=0, "Radial distance"=8.85, "Horizontal angle"=0.24870941840919195, "Vertical angle"=0.00698131700797732, "Echo pulse width"=176, "Reserved"=9}, {"flags"=0, "Echo"=0, "Radial distance"=8.870000000000001, "Horizontal angle"=0.24870941840919195, "Vertical angle"=0.020943951023931963, "Echo pulse width"=172, "Reserved"=9}, {"flags"=0, "Echo"=0, "Radial distance"=9.19, "Horizontal angle"=0.24434609527920614, "Vertical angle"=-0.020943951023931952, "Echo pulse width"=256, "Reserved"=9}, {"flags"=0, "Echo"=0, "Radial distance"=9.36, "Horizontal angle"=0.24434609527920614, "Vertical angle"=-0.006981317007977317, "Echo pulse width"=280, "Reserved"=9}, {"flags"=0, "Echo"=0, "Radial distance"=9.24, "Horizontal angle"=0.2399827721492203, "Vertical angle"=0.00698131700797732, "Echo pulse width"=208, "Reserved"=9}, {"flags"=0, "Echo"=0, "Radial distance"=9.200000000000001, "Horizontal angle"=0.2399827721492203, "Vertical angle"=0.020943951023931963, "Echo pulse width"=204, "Reserved"=9}, {"flags"=0, "Echo"=0, "Radial distance"=9.42, "Horizontal angle"=0.23561944901923448, "Vertical angle"=-0.020943951023931952, "Echo pulse width"=224, "Reserved"=9}, {"flags"=0, "Echo"=0, "Radial distance"=9.59, "Horizontal angle"=0.23561944901923448, "Vertical angle"=-0.006981317007977317, "Echo pulse width"=264, "Reserved"=9}, {"flags"=0, "Echo"=0, "Radial distance"=9.49, "Horizontal angle"=0.23125612588924865, "Vertical angle"=0.00698131700797732, "Echo pulse width"=176, "Reserved"=9}, {"flags"=0, "Echo"=0, "Radial distance"=9.35, "Horizontal angle"=0.23125612588924865, "Vertical angle"=0.020943951023931963, "Echo pulse width"=172, "Reserved"=9}, {"flags"=0, "Echo"=0, "Radial distance"=9.67, "Horizontal angle"=0.22689280275926282, "Vertical angle"=-0.020943951023931952, "Echo pulse width"=260, "Reserved"=9}, {"flags"=0, "Echo"=0, "Radial distance"=10.0, "Horizontal angle"=0.22689280275926282, "Vertical angle"=-0.006981317007977317, "Echo pulse width"=284, "Reserved"=9}, {"flags"=0, "Echo"=0, "Radial distance"=9.91, "Horizontal angle"=0.222529479629277, "Vertical angle"=0.00698131700797732, "Echo pulse width"=248, "Reserved"=9}, {"flags"=0, "Echo"=0, "Radial distance"=9.76, "Horizontal angle"=0.222529479629277, "Vertical angle"=0.020943951023931963, "Echo pulse width"=204, "Reserved"=9}, {"flags"=0, "Echo"=0, "Radial distance"=10.02, "Horizontal angle"=0.2181661564992912, "Vertical angle"=-0.020943951023931952, "Echo pulse width"=228, "Reserved"=9}, {"flags"=0, "Echo"=0, "Radial distance"=10.35, "Horizontal angle"=0.2181661564992912, "Vertical angle"=-0.006981317007977317, "Echo pulse width"=264, "Reserved"=9}, {"flags"=0, "Echo"=0, "Radial distance"=10.17, "Horizontal angle"=0.21380283336930533, "Vertical angle"=0.00698131700797732, "Echo pulse width"=180, "Reserved"=9}, {"flags"=0, "Echo"=0, "Radial distance"=10.07, "Horizontal angle"=0.21380283336930533, "Vertical angle"=0.020943951023931963, "Echo pulse width"=176, "Reserved"=9}, {"flags"=0, "Echo"=0, "Radial distance"=9.950000000000001, "Horizontal angle"=0.20943951023931953, "Vertical angle"=-0.020943951023931952, "Echo pulse width"=288, "Reserved"=9}, {"flags"=0, "Echo"=0, "Radial distance"=10.4, "Horizontal angle"=0.20943951023931953, "Vertical angle"=-0.006981317007977317, "Echo pulse width"=316, "Reserved"=9}, {"flags"=0, "Echo"=0, "Radial distance"=10.55, "Horizontal angle"=0.20507618710933373, "Vertical angle"=0.00698131700797732, "Echo pulse width"=268, "Reserved"=9}, {"flags"=0, "Echo"=0, "Radial distance"=10.32, "Horizontal angle"=0.20507618710933373, "Vertical angle"=0.020943951023931963, "Echo pulse width"=204, "Reserved"=9}, {"flags"=0, "Echo"=0, "Radial distance"=10.44, "Horizontal angle"=0.20071286397934787, "Vertical angle"=-0.020943951023931952, "Echo pulse width"=216, "Reserved"=9}, {"flags"=0, "Echo"=0, "Radial distance"=10.75, "Horizontal angle"=0.20071286397934787, "Vertical angle"=-0.006981317007977317, "Echo pulse width"=280, "Reserved"=9}, {"flags"=0, "Echo"=0, "Radial distance"=10.85, "Horizontal angle"=0.19634954084936207, "Vertical angle"=0.00698131700797732, "Echo pulse width"=176, "Reserved"=9}, {"flags"=0, "Echo"=0, "Radial distance"=10.8, "Horizontal angle"=0.19634954084936207, "Vertical angle"=0.020943951023931963, "Echo pulse width"=192, "Reserved"=9}, {"flags"=4, "Echo"=0, "Radial distance"=10.11, "Horizontal angle"=0.19198621771937624, "Vertical angle"=-0.020943951023931952, "Echo pulse width"=324, "Reserved"=0}, {"flags"=0, "Echo"=0, "Radial distance"=11.28, "Horizontal angle"=0.19198621771937624, "Vertical angle"=-0.006981317007977317, "Echo pulse width"=260, "Reserved"=9}, {"flags"=0, "Echo"=0, "Radial distance"=11.23, "Horizontal angle"=0.18762289458939044, "Vertical angle"=0.00698131700797732, "Echo pulse width"=220, "Reserved"=9}, {"flags"=0, "Echo"=0, "Radial distance"=11.120000000000001, "Horizontal angle"=0.18762289458939044, "Vertical angle"=0.020943951023931963, "Echo pulse width"=200, "Reserved"=9}, {"flags"=4, "Echo"=0, "Radial distance"=10.43, "Horizontal angle"=0.1832595714594046, "Vertical angle"=-0.020943951023931952, "Echo pulse width"=296, "Reserved"=0}, {"flags"=0, "Echo"=0, "Radial distance"=11.39, "Horizontal angle"=0.1832595714594046, "Vertical angle"=-0.006981317007977317, "Echo pulse width"=260, "Reserved"=9}, {"flags"=0, "Echo"=0, "Radial distance"=11.370000000000001, "Horizontal angle"=0.17889624832941878, "Vertical angle"=0.00698131700797732, "Echo pulse width"=172, "Reserved"=9}, {"flags"=0, "Echo"=0, "Radial distance"=11.51, "Horizontal angle"=0.17889624832941878, "Vertical angle"=0.020943951023931963, "Echo pulse width"=176, "Reserved"=9}, {"flags"=4, "Echo"=0, "Radial distance"=10.49, "Horizontal angle"=0.17453292519943295, "Vertical angle"=-0.020943951023931952, "Echo pulse width"=372, "Reserved"=0}, {"flags"=0, "Echo"=0, "Radial distance"=11.92, "Horizontal angle"=0.17453292519943295, "Vertical angle"=-0.006981317007977317, "Echo pulse width"=296, "Reserved"=9}, {"flags"=0, "Echo"=0, "Radial distance"=11.88, "Horizontal angle"=0.17016960206944715, "Vertical angle"=0.00698131700797732, "Echo pulse width"=208, "Reserved"=9}, {"flags"=0, "Echo"=0, "Radial distance"=12.040000000000001, "Horizontal angle"=0.17016960206944715, "Vertical angle"=0.020943951023931963, "Echo pulse width"=216, "Reserved"=9}, {"flags"=4, "Echo"=0, "Radial distance"=10.950000000000001, "Horizontal angle"=0.16580627893946132, "Vertical angle"=-0.020943951023931952, "Echo pulse width"=308, "Reserved"=0}, {"flags"=0, "Echo"=0, "Radial distance"=12.5, "Horizontal angle"=0.16580627893946132, "Vertical angle"=-0.006981317007977317, "Echo pulse width"=200, "Reserved"=9}, {"flags"=0, "Echo"=0, "Radial distance"=12.41, "Horizontal angle"=0.16144295580947549, "Vertical angle"=0.00698131700797732, "Echo pulse width"=172, "Reserved"=9}, {"flags"=0, "Echo"=0, "Radial distance"=12.71, "Horizontal angle"=0.16144295580947549, "Vertical angle"=0.020943951023931963, "Echo pulse width"=180, "Reserved"=9}, {"flags"=4, "Echo"=0, "Radial distance"=11.27, "Horizontal angle"=0.15707963267948966, "Vertical angle"=-0.020943951023931952, "Echo pulse width"=312, "Reserved"=0}, {"flags"=4, "Echo"=0, "Radial distance"=13.26, "Horizontal angle"=0.15707963267948966, "Vertical angle"=-0.006981317007977317, "Echo pulse width"=244, "Reserved"=0}, {"flags"=2, "Echo"=0, "Radial distance"=13.08, "Horizontal angle"=0.15271630954950383, "Vertical angle"=0.00698131700797732, "Echo pulse width"=212, "Reserved"=0}, {"flags"=3, "Echo"=0, "Radial distance"=13.27, "Horizontal angle"=0.15271630954950383, "Vertical angle"=0.020943951023931963, "Echo pulse width"=156, "Reserved"=0}, {"flags"=0, "Echo"=1, "Radial distance"=19.92, "Horizontal angle"=0.15271630954950383, "Vertical angle"=0.020943951023931963, "Echo pulse width"=176, "Reserved"=10}, {"flags"=4, "Echo"=0, "Radial distance"=11.790000000000001, "Horizontal angle"=0.148352986419518, "Vertical angle"=-0.020943951023931952, "Echo pulse width"=264, "Reserved"=0}, {"flags"=5, "Echo"=0, "Radial distance"=13.88, "Horizontal angle"=0.148352986419518, "Vertical angle"=-0.006981317007977317, "Echo pulse width"=168, "Reserved"=0}, {"flags"=5, "Echo"=1, "Radial distance"=15.94, "Horizontal angle"=0.148352986419518, "Vertical angle"=-0.006981317007977317, "Echo pulse width"=108, "Reserved"=0}, {"flags"=4, "Echo"=2, "Radial distance"=18.05, "Horizontal angle"=0.148352986419518, "Vertical angle"=-0.006981317007977317, "Echo pulse width"=340, "Reserved"=0}, {"flags"=0, "Echo"=0, "Radial distance"=19.580000000000002, "Horizontal angle"=0.14398966328953217, "Vertical angle"=0.00698131700797732, "Echo pulse width"=204, "Reserved"=10}, {"flags"=0, "Echo"=0, "Radial distance"=19.73, "Horizontal angle"=0.14398966328953217, "Vertical angle"=0.020943951023931963, "Echo pulse width"=188, "Reserved"=10}, {"flags"=4, "Echo"=0, "Radial distance"=12.19, "Horizontal angle"=0.13962634015954636, "Vertical angle"=-0.020943951023931952, "Echo pulse width"=296, "Reserved"=0}, {"flags"=3, "Echo"=0, "Radial distance"=13.52, "Horizontal angle"=0.13962634015954636, "Vertical angle"=-0.006981317007977317, "Echo pulse width"=128, "Reserved"=0}, {"flags"=5, "Echo"=1, "Radial distance"=15.610000000000001, "Horizontal angle"=0.13962634015954636, "Vertical angle"=-0.006981317007977317, "Echo pulse width"=392, "Reserved"=0}, {"flags"=0, "Echo"=2, "Radial distance"=19.61, "Horizontal angle"=0.13962634015954636, "Vertical angle"=-0.006981317007977317, "Echo pulse width"=148, "Reserved"=10}, {"flags"=0, "Echo"=0, "Radial distance"=19.56, "Horizontal angle"=0.13526301702956053, "Vertical angle"=0.00698131700797732, "Echo pulse width"=208, "Reserved"=10}, {"flags"=0, "Echo"=0, "Radial distance"=19.76, "Horizontal angle"=0.13526301702956053, "Vertical angle"=0.020943951023931963, "Echo pulse width"=192, "Reserved"=10}, {"flags"=4, "Echo"=0, "Radial distance"=12.83, "Horizontal angle"=0.1308996938995747, "Vertical angle"=-0.020943951023931952, "Echo pulse width"=288, "Reserved"=0}, {"flags"=5, "Echo"=0, "Radial distance"=14.97, "Horizontal angle"=0.1308996938995747, "Vertical angle"=-0.006981317007977317, "Echo pulse width"=400, "Reserved"=0}, {"flags"=0, "Echo"=1, "Radial distance"=19.35, "Horizontal angle"=0.1308996938995747, "Vertical angle"=-0.006981317007977317, "Echo pulse width"=204, "Reserved"=10}, {"flags"=0, "Echo"=0, "Radial distance"=19.59, "Horizontal angle"=0.1265363707695889, "Vertical angle"=0.00698131700797732, "Echo pulse width"=196, "Reserved"=10}, {"flags"=0, "Echo"=0, "Radial distance"=19.8, "Horizontal angle"=0.1265363707695889, "Vertical angle"=0.020943951023931963, "Echo pulse width"=200, "Reserved"=10}, {"flags"=4, "Echo"=0, "Radial distance"=13.39, "Horizontal angle"=0.12217304763960307, "Vertical angle"=-0.020943951023931952, "Echo pulse width"=292, "Reserved"=0}, {"flags"=5, "Echo"=0, "Radial distance"=15.700000000000001, "Horizontal angle"=0.12217304763960307, "Vertical angle"=-0.006981317007977317, "Echo pulse width"=172, "Reserved"=0}, {"flags"=4, "Echo"=1, "Radial distance"=17.69, "Horizontal angle"=0.12217304763960307, "Vertical angle"=-0.006981317007977317, "Echo pulse width"=380, "Reserved"=0}, {"flags"=0, "Echo"=0, "Radial distance"=19.75, "Horizontal angle"=0.11780972450961724, "Vertical angle"=0.00698131700797732, "Echo pulse width"=216, "Reserved"=10}, {"flags"=0, "Echo"=0, "Radial distance"=19.84, "Horizontal angle"=0.11780972450961724, "Vertical angle"=0.020943951023931963, "Echo pulse width"=200, "Reserved"=10}, {"flags"=5, "Echo"=0, "Radial distance"=13.99, "Horizontal angle"=0.11344640137963141, "Vertical angle"=-0.020943951023931952, "Echo pulse width"=152, "Reserved"=0}, {"flags"=4, "Echo"=1, "Radial distance"=15.35, "Horizontal angle"=0.11344640137963141, "Vertical angle"=-0.020943951023931952, "Echo pulse width"=120, "Reserved"=0}, {"flags"=4, "Echo"=0, "Radial distance"=16.45, "Horizontal angle"=0.11344640137963141, "Vertical angle"=-0.006981317007977317, "Echo pulse width"=500, "Reserved"=0}, {"flags"=0, "Echo"=0, "Radial distance"=19.71, "Horizontal angle"=0.1090830782496456, "Vertical angle"=0.00698131700797732, "Echo pulse width"=196, "Reserved"=10}, {"flags"=0, "Echo"=0, "Radial distance"=20.0, "Horizontal angle"=0.1090830782496456, "Vertical angle"=0.020943951023931963, "Echo pulse width"=200, "Reserved"=10}, {"flags"=4, "Echo"=0, "Radial distance"=14.72, "Horizontal angle"=0.10471975511965977, "Vertical angle"=-0.020943951023931952, "Echo pulse width"=172, "Reserved"=0}, {"flags"=4, "Echo"=0, "Radial distance"=17.25, "Horizontal angle"=0.10471975511965977, "Vertical angle"=-0.006981317007977317, "Echo pulse width"=420, "Reserved"=0}, {"flags"=0, "Echo"=0, "Radial distance"=19.72, "Horizontal angle"=0.10035643198967394, "Vertical angle"=0.00698131700797732, "Echo pulse width"=188, "Reserved"=10}, {"flags"=1, "Echo"=0, "Radial distance"=20.2, "Horizontal angle"=0.10035643198967394, "Vertical angle"=0.020943951023931963, "Echo pulse width"=204, "Reserved"=10}, {"flags"=0, "Echo"=1, "Radial distance"=22.21, "Horizontal angle"=0.10035643198967394, "Vertical angle"=0.020943951023931963, "Echo pulse width"=20, "Reserved"=11}, {"flags"=4, "Echo"=0, "Radial distance"=15.6, "Horizontal angle"=0.09599310885968812, "Vertical angle"=-0.020943951023931952, "Echo pulse width"=172, "Reserved"=0}, {"flags"=5, "Echo"=0, "Radial distance"=17.62, "Horizontal angle"=0.09599310885968812, "Vertical angle"=-0.006981317007977317, "Echo pulse width"=164, "Reserved"=0}, {"flags"=0, "Echo"=1, "Radial distance"=19.82, "Horizontal angle"=0.09599310885968812, "Vertical angle"=-0.006981317007977317, "Echo pulse width"=208, "Reserved"=10}, {"flags"=0, "Echo"=0, "Radial distance"=19.91, "Horizontal angle"=0.0916297857297023, "Vertical angle"=0.00698131700797732, "Echo pulse width"=192, "Reserved"=10}, {"flags"=0, "Echo"=0, "Radial distance"=20.52, "Horizontal angle"=0.0916297857297023, "Vertical angle"=0.020943951023931963, "Echo pulse width"=204, "Reserved"=10}, {"flags"=4, "Echo"=0, "Radial distance"=16.31, "Horizontal angle"=0.08726646259971647, "Vertical angle"=-0.020943951023931952, "Echo pulse width"=224, "Reserved"=0}, {"flags"=4, "Echo"=0, "Radial distance"=18.650000000000002, "Horizontal angle"=0.08726646259971647, "Vertical angle"=-0.006981317007977317, "Echo pulse width"=368, "Reserved"=0}, {"flags"=4, "Echo"=0, "Radial distance"=20.92, "Horizontal angle"=0.08290313946973066, "Vertical angle"=0.00698131700797732, "Echo pulse width"=184, "Reserved"=0}, {"flags"=4, "Echo"=0, "Radial distance"=21.46, "Horizontal angle"=0.08290313946973066, "Vertical angle"=0.020943951023931963, "Echo pulse width"=212, "Reserved"=0}, {"flags"=4, "Echo"=0, "Radial distance"=15.290000000000001, "Horizontal angle"=0.07853981633974483, "Vertical angle"=-0.020943951023931952, "Echo pulse width"=436, "Reserved"=0}, {"flags"=4, "Echo"=0, "Radial distance"=18.61, "Horizontal angle"=0.07853981633974483, "Vertical angle"=-0.006981317007977317, "Echo pulse width"=508, "Reserved"=0}, {"flags"=4, "Echo"=0, "Radial distance"=22.12, "Horizontal angle"=0.074176493209759, "Vertical angle"=0.00698131700797732, "Echo pulse width"=188, "Reserved"=0}, {"flags"=4, "Echo"=0, "Radial distance"=22.64, "Horizontal angle"=0.074176493209759, "Vertical angle"=0.020943951023931963, "Echo pulse width"=220, "Reserved"=0}, {"flags"=5, "Echo"=0, "Radial distance"=15.76, "Horizontal angle"=0.06981317007977318, "Vertical angle"=-0.020943951023931952, "Echo pulse width"=232, "Reserved"=0}, {"flags"=4, "Echo"=1, "Radial distance"=18.98, "Horizontal angle"=0.06981317007977318, "Vertical angle"=-0.020943951023931952, "Echo pulse width"=156, "Reserved"=0}, {"flags"=5, "Echo"=0, "Radial distance"=19.32, "Horizontal angle"=0.06981317007977318, "Vertical angle"=-0.006981317007977317, "Echo pulse width"=128, "Reserved"=0}, {"flags"=4, "Echo"=1, "Radial distance"=21.68, "Horizontal angle"=0.06981317007977318, "Vertical angle"=-0.006981317007977317, "Echo pulse width"=292, "Reserved"=0}, {"flags"=4, "Echo"=0, "Radial distance"=23.46, "Horizontal angle"=0.06544984694978735, "Vertical angle"=0.00698131700797732, "Echo pulse width"=200, "Reserved"=0}, {"flags"=4, "Echo"=0, "Radial distance"=24.44, "Horizontal angle"=0.06544984694978735, "Vertical angle"=0.020943951023931963, "Echo pulse width"=180, "Reserved"=0}, {"flags"=5, "Echo"=0, "Radial distance"=16.88, "Horizontal angle"=0.061086523819801536, "Vertical angle"=-0.020943951023931952, "Echo pulse width"=236, "Reserved"=0}, {"flags"=0, "Echo"=1, "Radial distance"=20.56, "Horizontal angle"=0.061086523819801536, "Vertical angle"=-0.020943951023931952, "Echo pulse width"=132, "Reserved"=10}, {"flags"=1, "Echo"=0, "Radial distance"=20.75, "Horizontal angle"=0.061086523819801536, "Vertical angle"=-0.006981317007977317, "Echo pulse width"=124, "Reserved"=10}, {"flags"=5, "Echo"=1, "Radial distance"=22.91, "Horizontal angle"=0.061086523819801536, "Vertical angle"=-0.006981317007977317, "Echo pulse width"=200, "Reserved"=0}, {"flags"=0, "Echo"=2, "Radial distance"=24.85, "Horizontal angle"=0.061086523819801536, "Vertical angle"=-0.006981317007977317, "Echo pulse width"=156, "Reserved"=12}, {"flags"=0, "Echo"=0, "Radial distance"=25.14, "Horizontal angle"=0.056723200689815706, "Vertical angle"=0.00698131700797732, "Echo pulse width"=204, "Reserved"=12}, {"flags"=0, "Echo"=0, "Radial distance"=26.37, "Horizontal angle"=0.056723200689815706, "Vertical angle"=0.020943951023931963, "Echo pulse width"=64, "Reserved"=13}, {"flags"=5, "Echo"=0, "Radial distance"=18.31, "Horizontal angle"=0.05235987755982988, "Vertical angle"=-0.020943951023931952, "Echo pulse width"=248, "Reserved"=0}, {"flags"=0, "Echo"=1, "Radial distance"=22.41, "Horizontal angle"=0.05235987755982988, "Vertical angle"=-0.020943951023931952, "Echo pulse width"=84, "Reserved"=14}, {"flags"=1, "Echo"=0, "Radial distance"=22.6, "Horizontal angle"=0.05235987755982988, "Vertical angle"=-0.006981317007977317, "Echo pulse width"=136, "Reserved"=14}, {"flags"=1, "Echo"=1, "Radial distance"=24.97, "Horizontal angle"=0.05235987755982988, "Vertical angle"=-0.006981317007977317, "Echo pulse width"=144, "Reserved"=12}, {"flags"=0, "Echo"=2, "Radial distance"=26.560000000000002, "Horizontal angle"=0.05235987755982988, "Vertical angle"=-0.006981317007977317, "Echo pulse width"=128, "Reserved"=13}, {"flags"=4, "Echo"=0, "Radial distance"=32.79, "Horizontal angle"=0.04799655442984406, "Vertical angle"=0.00698131700797732, "Echo pulse width"=176, "Reserved"=0}, {"flags"=4, "Echo"=0, "Radial distance"=20.11, "Horizontal angle"=0.04363323129985824, "Vertical angle"=-0.020943951023931952, "Echo pulse width"=264, "Reserved"=0}, {"flags"=5, "Echo"=0, "Radial distance"=24.76, "Horizontal angle"=0.04363323129985824, "Vertical angle"=-0.006981317007977317, "Echo pulse width"=132, "Reserved"=0}, {"flags"=5, "Echo"=1, "Radial distance"=28.05, "Horizontal angle"=0.04363323129985824, "Vertical angle"=-0.006981317007977317, "Echo pulse width"=224, "Reserved"=0}, {"flags"=4, "Echo"=2, "Radial distance"=31.12, "Horizontal angle"=0.04363323129985824, "Vertical angle"=-0.006981317007977317, "Echo pulse width"=92, "Reserved"=0}, {"flags"=4, "Echo"=0, "Radial distance"=32.99, "Horizontal angle"=0.039269908169872414, "Vertical angle"=0.00698131700797732, "Echo pulse width"=180, "Reserved"=0}, {"flags"=4, "Echo"=0, "Radial distance"=22.52, "Horizontal angle"=0.03490658503988659, "Vertical angle"=-0.020943951023931952, "Echo pulse width"=236, "Reserved"=0}, {"flags"=5, "Echo"=0, "Radial distance"=27.490000000000002, "Horizontal angle"=0.03490658503988659, "Vertical angle"=-0.006981317007977317, "Echo pulse width"=144, "Reserved"=0}, {"flags"=4, "Echo"=1, "Radial distance"=31.14, "Horizontal angle"=0.03490658503988659, "Vertical angle"=-0.006981317007977317, "Echo pulse width"=208, "Reserved"=0}, {"flags"=0, "Echo"=0, "Radial distance"=33.94, "Horizontal angle"=0.030543261909900768, "Vertical angle"=0.00698131700797732, "Echo pulse width"=200, "Reserved"=15}, {"flags"=4, "Echo"=0, "Radial distance"=24.73, "Horizontal angle"=0.02617993877991494, "Vertical angle"=-0.020943951023931952, "Echo pulse width"=80, "Reserved"=0}, {"flags"=5, "Echo"=0, "Radial distance"=30.580000000000002, "Horizontal angle"=0.02617993877991494, "Vertical angle"=-0.006981317007977317, "Echo pulse width"=168, "Reserved"=0}, {"flags"=1, "Echo"=1, "Radial distance"=34.27, "Horizontal angle"=0.02617993877991494, "Vertical angle"=-0.006981317007977317, "Echo pulse width"=112, "Reserved"=15}, {"flags"=4, "Echo"=2, "Radial distance"=36.050000000000004, "Horizontal angle"=0.02617993877991494, "Vertical angle"=-0.006981317007977317, "Echo pulse width"=76, "Reserved"=0}, {"flags"=4, "Echo"=0, "Radial distance"=37.57, "Horizontal angle"=0.02181661564992912, "Vertical angle"=0.00698131700797732, "Echo pulse width"=236, "Reserved"=0}, {"flags"=5, "Echo"=0, "Radial distance"=29.080000000000002, "Horizontal angle"=0.017453292519943295, "Vertical angle"=-0.006981317007977317, "Echo pulse width"=192, "Reserved"=0}, {"flags"=5, "Echo"=1, "Radial distance"=34.93, "Horizontal angle"=0.017453292519943295, "Vertical angle"=-0.006981317007977317, "Echo pulse width"=100, "Reserved"=0}, {"flags"=4, "Echo"=2, "Radial distance"=38.480000000000004, "Horizontal angle"=0.017453292519943295, "Vertical angle"=-0.006981317007977317, "Echo pulse width"=132, "Reserved"=0}, {"flags"=0, "Echo"=0, "Radial distance"=54.64, "Horizontal angle"=0.01308996938995747, "Vertical angle"=0.00698131700797732, "Echo pulse width"=188, "Reserved"=16}, {"flags"=0, "Echo"=0, "Radial distance"=54.18, "Horizontal angle"=0.01308996938995747, "Vertical angle"=0.020943951023931963, "Echo pulse width"=92, "Reserved"=16}, {"flags"=5, "Echo"=0, "Radial distance"=32.88, "Horizontal angle"=0.008726646259971648, "Vertical angle"=-0.006981317007977317, "Echo pulse width"=192, "Reserved"=0}, {"flags"=5, "Echo"=1, "Radial distance"=34.25, "Horizontal angle"=0.008726646259971648, "Vertical angle"=-0.006981317007977317, "Echo pulse width"=76, "Reserved"=0}, {"flags"=4, "Echo"=2, "Radial distance"=40.58, "Horizontal angle"=0.008726646259971648, "Vertical angle"=-0.006981317007977317, "Echo pulse width"=104, "Reserved"=0}, {"flags"=4, "Echo"=0, "Radial distance"=22.93, "Horizontal angle"=0.0, "Vertical angle"=-0.020943951023931952, "Echo pulse width"=84, "Reserved"=0}, {"flags"=4, "Echo"=0, "Radial distance"=22.61, "Horizontal angle"=-0.008726646259971648, "Vertical angle"=-0.020943951023931952, "Echo pulse width"=208, "Reserved"=0}, {"flags"=0, "Echo"=0, "Radial distance"=71.72, "Horizontal angle"=-0.01308996938995747, "Vertical angle"=0.00698131700797732, "Echo pulse width"=144, "Reserved"=17}, {"flags"=5, "Echo"=0, "Radial distance"=21.75, "Horizontal angle"=-0.017453292519943295, "Vertical angle"=-0.020943951023931952, "Echo pulse width"=188, "Reserved"=0}, {"flags"=4, "Echo"=1, "Radial distance"=23.55, "Horizontal angle"=-0.017453292519943295, "Vertical angle"=-0.020943951023931952, "Echo pulse width"=120, "Reserved"=0}, {"flags"=0, "Echo"=0, "Radial distance"=71.49, "Horizontal angle"=-0.017453292519943295, "Vertical angle"=-0.006981317007977317, "Echo pulse width"=52, "Reserved"=17}, {"flags"=5, "Echo"=0, "Radial distance"=21.03, "Horizontal angle"=-0.02617993877991494, "Vertical angle"=-0.020943951023931952, "Echo pulse width"=184, "Reserved"=0}, {"flags"=4, "Echo"=1, "Radial distance"=24.19, "Horizontal angle"=-0.02617993877991494, "Vertical angle"=-0.020943951023931952, "Echo pulse width"=112, "Reserved"=0}, {"flags"=0, "Echo"=0, "Radial distance"=58.050000000000004, "Horizontal angle"=-0.02617993877991494, "Vertical angle"=-0.006981317007977317, "Echo pulse width"=48, "Reserved"=18}, {"flags"=5, "Echo"=0, "Radial distance"=21.240000000000002, "Horizontal angle"=-0.03490658503988659, "Vertical angle"=-0.020943951023931952, "Echo pulse width"=168, "Reserved"=0}, {"flags"=4, "Echo"=1, "Radial distance"=24.47, "Horizontal angle"=-0.03490658503988659, "Vertical angle"=-0.020943951023931952, "Echo pulse width"=116, "Reserved"=0}, {"flags"=5, "Echo"=0, "Radial distance"=21.830000000000002, "Horizontal angle"=-0.04363323129985824, "Vertical angle"=-0.020943951023931952, "Echo pulse width"=164, "Reserved"=0}, {"flags"=4, "Echo"=1, "Radial distance"=23.71, "Horizontal angle"=-0.04363323129985824, "Vertical angle"=-0.020943951023931952, "Echo pulse width"=116, "Reserved"=0}, {"flags"=4, "Echo"=0, "Radial distance"=22.650000000000002, "Horizontal angle"=-0.05235987755982988, "Vertical angle"=-0.020943951023931952, "Echo pulse width"=212, "Reserved"=0}, {"flags"=0, "Echo"=0, "Radial distance"=229.02, "Horizontal angle"=-0.06544984694978735, "Vertical angle"=0.00698131700797732, "Echo pulse width"=128, "Reserved"=19}, {"flags"=0, "Echo"=0, "Radial distance"=188.3, "Horizontal angle"=-0.06544984694978735, "Vertical angle"=0.020943951023931963, "Echo pulse width"=144, "Reserved"=20}, {"flags"=1, "Echo"=0, "Radial distance"=38.07, "Horizontal angle"=-0.06981317007977318, "Vertical angle"=-0.006981317007977317, "Echo pulse width"=204, "Reserved"=21}, {"flags"=1, "Echo"=1, "Radial distance"=39.56, "Horizontal angle"=-0.06981317007977318, "Vertical angle"=-0.006981317007977317, "Echo pulse width"=88, "Reserved"=22}, {"flags"=0, "Echo"=2, "Radial distance"=57.84, "Horizontal angle"=-0.06981317007977318, "Vertical angle"=-0.006981317007977317, "Echo pulse width"=36, "Reserved"=23}, {"flags"=4, "Echo"=0, "Radial distance"=30.03, "Horizontal angle"=-0.07853981633974483, "Vertical angle"=-0.006981317007977317, "Echo pulse width"=200, "Reserved"=0}, {"flags"=4, "Echo"=0, "Radial distance"=21.91, "Horizontal angle"=-0.08726646259971647, "Vertical angle"=-0.020943951023931952, "Echo pulse width"=340, "Reserved"=0}, {"flags"=0, "Echo"=0, "Radial distance"=58.21, "Horizontal angle"=-0.08726646259971647, "Vertical angle"=-0.006981317007977317, "Echo pulse width"=52, "Reserved"=24}, {"flags"=0, "Echo"=0, "Radial distance"=88.99, "Horizontal angle"=-0.10035643198967394, "Vertical angle"=0.00698131700797732, "Echo pulse width"=76, "Reserved"=25}, {"flags"=4, "Echo"=0, "Radial distance"=15.52, "Horizontal angle"=-0.10471975511965977, "Vertical angle"=-0.020943951023931952, "Echo pulse width"=236, "Reserved"=0}, {"flags"=0, "Echo"=0, "Radial distance"=89.03, "Horizontal angle"=-0.1090830782496456, "Vertical angle"=0.00698131700797732, "Echo pulse width"=140, "Reserved"=25}, {"flags"=4, "Echo"=0, "Radial distance"=14.870000000000001, "Horizontal angle"=-0.11344640137963141, "Vertical angle"=-0.020943951023931952, "Echo pulse width"=76, "Reserved"=0}, {"flags"=0, "Echo"=0, "Radial distance"=287.03000000000003, "Horizontal angle"=-0.11780972450961724, "Vertical angle"=0.00698131700797732, "Echo pulse width"=140, "Reserved"=26}, {"flags"=4, "Echo"=0, "Radial distance"=22.91, "Horizontal angle"=-0.12217304763960307, "Vertical angle"=-0.020943951023931952, "Echo pulse width"=116, "Reserved"=0}, {"flags"=0, "Echo"=0, "Radial distance"=69.89, "Horizontal angle"=-0.1265363707695889, "Vertical angle"=0.020943951023931963, "Echo pulse width"=132, "Reserved"=27}, {"flags"=4, "Echo"=0, "Radial distance"=22.91, "Horizontal angle"=-0.1308996938995747, "Vertical angle"=-0.020943951023931952, "Echo pulse width"=252, "Reserved"=0}, {"flags"=0, "Echo"=0, "Radial distance"=153.20000000000002, "Horizontal angle"=-0.13526301702956053, "Vertical angle"=0.020943951023931963, "Echo pulse width"=48, "Reserved"=28}, {"flags"=5, "Echo"=0, "Radial distance"=22.1, "Horizontal angle"=-0.13962634015954636, "Vertical angle"=-0.020943951023931952, "Echo pulse width"=156, "Reserved"=0}, {"flags"=4, "Echo"=1, "Radial distance"=24.42, "Horizontal angle"=-0.13962634015954636, "Vertical angle"=-0.020943951023931952, "Echo pulse width"=152, "Reserved"=0}, {"flags"=4, "Echo"=0, "Radial distance"=47.07, "Horizontal angle"=-0.13962634015954636, "Vertical angle"=-0.006981317007977317, "Echo pulse width"=40, "Reserved"=0}, {"flags"=5, "Echo"=0, "Radial distance"=21.6, "Horizontal angle"=-0.148352986419518, "Vertical angle"=-0.020943951023931952, "Echo pulse width"=172, "Reserved"=0}, {"flags"=4, "Echo"=1, "Radial distance"=24.560000000000002, "Horizontal angle"=-0.148352986419518, "Vertical angle"=-0.020943951023931952, "Echo pulse width"=88, "Reserved"=0}, {"flags"=4, "Echo"=0, "Radial distance"=42.27, "Horizontal angle"=-0.148352986419518, "Vertical angle"=-0.006981317007977317, "Echo pulse width"=84, "Reserved"=0}, {"flags"=0, "Echo"=0, "Radial distance"=96.75, "Horizontal angle"=-0.15271630954950383, "Vertical angle"=0.00698131700797732, "Echo pulse width"=136, "Reserved"=29}, {"flags"=5, "Echo"=0, "Radial distance"=21.12, "Horizontal angle"=-0.15707963267948966, "Vertical angle"=-0.020943951023931952, "Echo pulse width"=176, "Reserved"=0}, {"flags"=4, "Echo"=1, "Radial distance"=24.02, "Horizontal angle"=-0.15707963267948966, "Vertical angle"=-0.020943951023931952, "Echo pulse width"=96, "Reserved"=0}, {"flags"=4, "Echo"=0, "Radial distance"=38.67, "Horizontal angle"=-0.15707963267948966, "Vertical angle"=-0.006981317007977317, "Echo pulse width"=120, "Reserved"=0}, {"flags"=0, "Echo"=0, "Radial distance"=84.31, "Horizontal angle"=-0.16144295580947549, "Vertical angle"=0.00698131700797732, "Echo pulse width"=104, "Reserved"=30}, {"flags"=5, "Echo"=0, "Radial distance"=21.52, "Horizontal angle"=-0.16580627893946132, "Vertical angle"=-0.020943951023931952, "Echo pulse width"=232, "Reserved"=0}, {"flags"=4, "Echo"=1, "Radial distance"=23.6, "Horizontal angle"=-0.16580627893946132, "Vertical angle"=-0.020943951023931952, "Echo pulse width"=92, "Reserved"=0}, {"flags"=5, "Echo"=0, "Radial distance"=30.400000000000002, "Horizontal angle"=-0.16580627893946132, "Vertical angle"=-0.006981317007977317, "Echo pulse width"=132, "Reserved"=0}, {"flags"=4, "Echo"=1, "Radial distance"=35.68, "Horizontal angle"=-0.16580627893946132, "Vertical angle"=-0.006981317007977317, "Echo pulse width"=128, "Reserved"=0}, {"flags"=1, "Echo"=0, "Radial distance"=74.71000000000001, "Horizontal angle"=-0.17016960206944715, "Vertical angle"=0.00698131700797732, "Echo pulse width"=104, "Reserved"=31}, {"flags"=0, "Echo"=1, "Radial distance"=76.92, "Horizontal angle"=-0.17016960206944715, "Vertical angle"=0.00698131700797732, "Echo pulse width"=148, "Reserved"=32}, {"flags"=0, "Echo"=0, "Radial distance"=76.97, "Horizontal angle"=-0.17016960206944715, "Vertical angle"=0.020943951023931963, "Echo pulse width"=128, "Reserved"=32}, {"flags"=4, "Echo"=0, "Radial distance"=22.63, "Horizontal angle"=-0.17453292519943295, "Vertical angle"=-0.020943951023931952, "Echo pulse width"=224, "Reserved"=0}, {"flags"=4, "Echo"=0, "Radial distance"=33.160000000000004, "Horizontal angle"=-0.17453292519943295, "Vertical angle"=-0.006981317007977317, "Echo pulse width"=128, "Reserved"=0}, {"flags"=0, "Echo"=0, "Radial distance"=70.54, "Horizontal angle"=-0.17889624832941878, "Vertical angle"=0.00698131700797732, "Echo pulse width"=128, "Reserved"=33}, {"flags"=4, "Echo"=0, "Radial distance"=31.080000000000002, "Horizontal angle"=-0.1832595714594046, "Vertical angle"=-0.006981317007977317, "Echo pulse width"=128, "Reserved"=0}, {"flags"=0, "Echo"=0, "Radial distance"=62.67, "Horizontal angle"=-0.18762289458939044, "Vertical angle"=0.00698131700797732, "Echo pulse width"=136, "Reserved"=34}, {"flags"=4, "Echo"=0, "Radial distance"=24.96, "Horizontal angle"=-0.19198621771937624, "Vertical angle"=-0.020943951023931952, "Echo pulse width"=136, "Reserved"=0}, {"flags"=4, "Echo"=0, "Radial distance"=29.32, "Horizontal angle"=-0.19198621771937624, "Vertical angle"=-0.006981317007977317, "Echo pulse width"=136, "Reserved"=0}, {"flags"=0, "Echo"=0, "Radial distance"=58.64, "Horizontal angle"=-0.19634954084936207, "Vertical angle"=0.00698131700797732, "Echo pulse width"=148, "Reserved"=35}, {"flags"=0, "Echo"=0, "Radial distance"=70.59, "Horizontal angle"=-0.19634954084936207, "Vertical angle"=0.020943951023931963, "Echo pulse width"=116, "Reserved"=36}, {"flags"=4, "Echo"=0, "Radial distance"=23.59, "Horizontal angle"=-0.20071286397934787, "Vertical angle"=-0.020943951023931952, "Echo pulse width"=160, "Reserved"=0}, {"flags"=4, "Echo"=0, "Radial distance"=27.68, "Horizontal angle"=-0.20071286397934787, "Vertical angle"=-0.006981317007977317, "Echo pulse width"=136, "Reserved"=0}, {"flags"=0, "Echo"=0, "Radial distance"=54.61, "Horizontal angle"=-0.20507618710933373, "Vertical angle"=0.00698131700797732, "Echo pulse width"=152, "Reserved"=37}, {"flags"=0, "Echo"=0, "Radial distance"=94.06, "Horizontal angle"=-0.20507618710933373, "Vertical angle"=0.020943951023931963, "Echo pulse width"=108, "Reserved"=38}, {"flags"=4, "Echo"=0, "Radial distance"=22.32, "Horizontal angle"=-0.20943951023931953, "Vertical angle"=-0.020943951023931952, "Echo pulse width"=172, "Reserved"=0}, {"flags"=4, "Echo"=0, "Radial distance"=26.16, "Horizontal angle"=-0.20943951023931953, "Vertical angle"=-0.006981317007977317, "Echo pulse width"=140, "Reserved"=0}, {"flags"=5, "Echo"=0, "Radial distance"=49.84, "Horizontal angle"=-0.21380283336930533, "Vertical angle"=0.00698131700797732, "Echo pulse width"=148, "Reserved"=0}, {"flags"=0, "Echo"=1, "Radial distance"=54.76, "Horizontal angle"=-0.21380283336930533, "Vertical angle"=0.00698131700797732, "Echo pulse width"=56, "Reserved"=37}, {"flags"=1, "Echo"=0, "Radial distance"=58.45, "Horizontal angle"=-0.21380283336930533, "Vertical angle"=0.020943951023931963, "Echo pulse width"=32, "Reserved"=39}, {"flags"=0, "Echo"=1, "Radial distance"=62.25, "Horizontal angle"=-0.21380283336930533, "Vertical angle"=0.020943951023931963, "Echo pulse width"=64, "Reserved"=40}, {"flags"=4, "Echo"=0, "Radial distance"=21.150000000000002, "Horizontal angle"=-0.2181661564992912, "Vertical angle"=-0.020943951023931952, "Echo pulse width"=164, "Reserved"=0}, {"flags"=5, "Echo"=0, "Radial distance"=24.97, "Horizontal angle"=-0.2181661564992912, "Vertical angle"=-0.006981317007977317, "Echo pulse width"=144, "Reserved"=0}, {"flags"=4, "Echo"=1, "Radial distance"=26.35, "Horizontal angle"=-0.2181661564992912, "Vertical angle"=-0.006981317007977317, "Echo pulse width"=64, "Reserved"=0}, {"flags"=4, "Echo"=0, "Radial distance"=49.5, "Horizontal angle"=-0.222529479629277, "Vertical angle"=0.00698131700797732, "Echo pulse width"=160, "Reserved"=0}, {"flags"=0, "Echo"=0, "Radial distance"=93.9, "Horizontal angle"=-0.222529479629277, "Vertical angle"=0.020943951023931963, "Echo pulse width"=92, "Reserved"=41}, {"flags"=5, "Echo"=0, "Radial distance"=20.13, "Horizontal angle"=-0.22689280275926282, "Vertical angle"=-0.020943951023931952, "Echo pulse width"=148, "Reserved"=0}, {"flags"=4, "Echo"=1, "Radial distance"=22.12, "Horizontal angle"=-0.22689280275926282, "Vertical angle"=-0.020943951023931952, "Echo pulse width"=136, "Reserved"=0}, {"flags"=5, "Echo"=0, "Radial distance"=23.72, "Horizontal angle"=-0.22689280275926282, "Vertical angle"=-0.006981317007977317, "Echo pulse width"=136, "Reserved"=0}, {"flags"=4, "Echo"=1, "Radial distance"=25.01, "Horizontal angle"=-0.22689280275926282, "Vertical angle"=-0.006981317007977317, "Echo pulse width"=100, "Reserved"=0}, {"flags"=4, "Echo"=0, "Radial distance"=44.88, "Horizontal angle"=-0.23125612588924865, "Vertical angle"=0.00698131700797732, "Echo pulse width"=148, "Reserved"=0}, {"flags"=0, "Echo"=0, "Radial distance"=63.27, "Horizontal angle"=-0.23125612588924865, "Vertical angle"=0.020943951023931963, "Echo pulse width"=112, "Reserved"=42}, {"flags"=5, "Echo"=0, "Radial distance"=19.240000000000002, "Horizontal angle"=-0.23561944901923448, "Vertical angle"=-0.020943951023931952, "Echo pulse width"=168, "Reserved"=0}, {"flags"=0, "Echo"=1, "Radial distance"=22.32, "Horizontal angle"=-0.23561944901923448, "Vertical angle"=-0.020943951023931952, "Echo pulse width"=176, "Reserved"=43}, {"flags"=4, "Echo"=0, "Radial distance"=23.06, "Horizontal angle"=-0.23561944901923448, "Vertical angle"=-0.006981317007977317, "Echo pulse width"=244, "Reserved"=0}, {"flags"=4, "Echo"=0, "Radial distance"=44.5, "Horizontal angle"=-0.2399827721492203, "Vertical angle"=0.00698131700797732, "Echo pulse width"=160, "Reserved"=0}, {"flags"=0, "Echo"=0, "Radial distance"=74.82000000000001, "Horizontal angle"=-0.2399827721492203, "Vertical angle"=0.020943951023931963, "Echo pulse width"=84, "Reserved"=44}, {"flags"=5, "Echo"=0, "Radial distance"=18.48, "Horizontal angle"=-0.24434609527920614, "Vertical angle"=-0.020943951023931952, "Echo pulse width"=176, "Reserved"=0}, {"flags"=0, "Echo"=1, "Radial distance"=21.59, "Horizontal angle"=-0.24434609527920614, "Vertical angle"=-0.020943951023931952, "Echo pulse width"=116, "Reserved"=43}, {"flags"=0, "Echo"=0, "Radial distance"=22.1, "Horizontal angle"=-0.24434609527920614, "Vertical angle"=-0.006981317007977317, "Echo pulse width"=248, "Reserved"=43}, {"flags"=1, "Echo"=0, "Radial distance"=39.93, "Horizontal angle"=-0.24870941840919195, "Vertical angle"=0.00698131700797732, "Echo pulse width"=156, "Reserved"=45}, {"flags"=0, "Echo"=1, "Radial distance"=44.6, "Horizontal angle"=-0.24870941840919195, "Vertical angle"=0.00698131700797732, "Echo pulse width"=84, "Reserved"=46}, {"flags"=0, "Echo"=0, "Radial distance"=95.45, "Horizontal angle"=-0.24870941840919195, "Vertical angle"=0.020943951023931963, "Echo pulse width"=76, "Reserved"=47}, {"flags"=5, "Echo"=0, "Radial distance"=17.68, "Horizontal angle"=-0.2530727415391778, "Vertical angle"=-0.020943951023931952, "Echo pulse width"=176, "Reserved"=0}, {"flags"=0, "Echo"=1, "Radial distance"=20.39, "Horizontal angle"=-0.2530727415391778, "Vertical angle"=-0.020943951023931952, "Echo pulse width"=196, "Reserved"=48}, {"flags"=0, "Echo"=0, "Radial distance"=21.32, "Horizontal angle"=-0.2530727415391778, "Vertical angle"=-0.006981317007977317, "Echo pulse width"=264, "Reserved"=43}, {"flags"=0, "Echo"=0, "Radial distance"=39.7, "Horizontal angle"=-0.2574360646691636, "Vertical angle"=0.00698131700797732, "Echo pulse width"=168, "Reserved"=45}, {"flags"=0, "Echo"=0, "Radial distance"=39.83, "Horizontal angle"=-0.2574360646691636, "Vertical angle"=0.020943951023931963, "Echo pulse width"=116, "Reserved"=45}, {"flags"=5, "Echo"=0, "Radial distance"=17.03, "Horizontal angle"=-0.2617993877991494, "Vertical angle"=-0.020943951023931952, "Echo pulse width"=192, "Reserved"=0}, {"flags"=4, "Echo"=1, "Radial distance"=19.43, "Horizontal angle"=-0.2617993877991494, "Vertical angle"=-0.020943951023931952, "Echo pulse width"=220, "Reserved"=0}, {"flags"=1, "Echo"=0, "Radial distance"=20.57, "Horizontal angle"=-0.2617993877991494, "Vertical angle"=-0.006981317007977317, "Echo pulse width"=232, "Reserved"=48}, {"flags"=4, "Echo"=1, "Radial distance"=22.67, "Horizontal angle"=-0.2617993877991494, "Vertical angle"=-0.006981317007977317, "Echo pulse width"=120, "Reserved"=0}, {"flags"=0, "Echo"=0, "Radial distance"=39.62, "Horizontal angle"=-0.26616271092913524, "Vertical angle"=0.00698131700797732, "Echo pulse width"=168, "Reserved"=45}, {"flags"=0, "Echo"=0, "Radial distance"=39.83, "Horizontal angle"=-0.26616271092913524, "Vertical angle"=0.020943951023931963, "Echo pulse width"=116, "Reserved"=45}, {"flags"=4, "Echo"=0, "Radial distance"=16.53, "Horizontal angle"=-0.27052603405912107, "Vertical angle"=-0.020943951023931952, "Echo pulse width"=440, "Reserved"=0}, {"flags"=5, "Echo"=0, "Radial distance"=20.080000000000002, "Horizontal angle"=-0.27052603405912107, "Vertical angle"=-0.006981317007977317, "Echo pulse width"=260, "Reserved"=0}, {"flags"=4, "Echo"=1, "Radial distance"=22.47, "Horizontal angle"=-0.27052603405912107, "Vertical angle"=-0.006981317007977317, "Echo pulse width"=64, "Reserved"=0}, {"flags"=0, "Echo"=0, "Radial distance"=39.9, "Horizontal angle"=-0.2748893571891069, "Vertical angle"=0.00698131700797732, "Echo pulse width"=172, "Reserved"=45}, {"flags"=0, "Echo"=0, "Radial distance"=95.94, "Horizontal angle"=-0.2748893571891069, "Vertical angle"=0.020943951023931963, "Echo pulse width"=92, "Reserved"=49}, {"flags"=4, "Echo"=0, "Radial distance"=16.05, "Horizontal angle"=-0.2792526803190927, "Vertical angle"=-0.020943951023931952, "Echo pulse width"=424, "Reserved"=0}, {"flags"=5, "Echo"=0, "Radial distance"=19.42, "Horizontal angle"=-0.2792526803190927, "Vertical angle"=-0.006981317007977317, "Echo pulse width"=160, "Reserved"=0}, {"flags"=5, "Echo"=1, "Radial distance"=20.650000000000002, "Horizontal angle"=-0.2792526803190927, "Vertical angle"=-0.006981317007977317, "Echo pulse width"=76, "Reserved"=0}, {"flags"=4, "Echo"=2, "Radial distance"=22.6, "Horizontal angle"=-0.2792526803190927, "Vertical angle"=-0.006981317007977317, "Echo pulse width"=60, "Reserved"=0}, {"flags"=0, "Echo"=0, "Radial distance"=34.82, "Horizontal angle"=-0.28361600344907856, "Vertical angle"=0.00698131700797732, "Echo pulse width"=172, "Reserved"=50}, {"flags"=1, "Echo"=0, "Radial distance"=35.06, "Horizontal angle"=-0.28361600344907856, "Vertical angle"=0.020943951023931963, "Echo pulse width"=148, "Reserved"=50}, {"flags"=0, "Echo"=1, "Radial distance"=59.39, "Horizontal angle"=-0.28361600344907856, "Vertical angle"=0.020943951023931963, "Echo pulse width"=96, "Reserved"=51}, {"flags"=4, "Echo"=0, "Radial distance"=15.81, "Horizontal angle"=-0.28797932657906433, "Vertical angle"=-0.020943951023931952, "Echo pulse width"=392, "Reserved"=0}, {"flags"=5, "Echo"=0, "Radial distance"=19.1, "Horizontal angle"=-0.28797932657906433, "Vertical angle"=-0.006981317007977317, "Echo pulse width"=208, "Reserved"=0}, {"flags"=5, "Echo"=1, "Radial distance"=20.830000000000002, "Horizontal angle"=-0.28797932657906433, "Vertical angle"=-0.006981317007977317, "Echo pulse width"=40, "Reserved"=0}, {"flags"=4, "Echo"=2, "Radial distance"=22.11, "Horizontal angle"=-0.28797932657906433, "Vertical angle"=-0.006981317007977317, "Echo pulse width"=84, "Reserved"=0}, {"flags"=0, "Echo"=0, "Radial distance"=34.79, "Horizontal angle"=-0.2923426497090502, "Vertical angle"=0.00698131700797732, "Echo pulse width"=176, "Reserved"=50}, {"flags"=1, "Echo"=0, "Radial distance"=34.99, "Horizontal angle"=-0.2923426497090502, "Vertical angle"=0.020943951023931963, "Echo pulse width"=160, "Reserved"=50}, {"flags"=0, "Echo"=1, "Radial distance"=94.31, "Horizontal angle"=-0.2923426497090502, "Vertical angle"=0.020943951023931963, "Echo pulse width"=12, "Reserved"=52}, {"flags"=4, "Echo"=0, "Radial distance"=16.43, "Horizontal angle"=-0.296705972839036, "Vertical angle"=-0.020943951023931952, "Echo pulse width"=268, "Reserved"=0}, {"flags"=5, "Echo"=0, "Radial distance"=18.740000000000002, "Horizontal angle"=-0.296705972839036, "Vertical angle"=-0.006981317007977317, "Echo pulse width"=244, "Reserved"=0}, {"flags"=4, "Echo"=1, "Radial distance"=21.62, "Horizontal angle"=-0.296705972839036, "Vertical angle"=-0.006981317007977317, "Echo pulse width"=168, "Reserved"=0}, {"flags"=4, "Echo"=0, "Radial distance"=34.03, "Horizontal angle"=-0.3010692959690219, "Vertical angle"=0.00698131700797732, "Echo pulse width"=264, "Reserved"=0}, {"flags"=0, "Echo"=0, "Radial distance"=34.9, "Horizontal angle"=-0.3010692959690219, "Vertical angle"=0.020943951023931963, "Echo pulse width"=148, "Reserved"=50}, {"flags"=4, "Echo"=0, "Radial distance"=16.35, "Horizontal angle"=-0.30543261909900765, "Vertical angle"=-0.020943951023931952, "Echo pulse width"=216, "Reserved"=0}, {"flags"=5, "Echo"=0, "Radial distance"=18.28, "Horizontal angle"=-0.30543261909900765, "Vertical angle"=-0.006981317007977317, "Echo pulse width"=296, "Reserved"=0}, {"flags"=5, "Echo"=1, "Radial distance"=21.87, "Horizontal angle"=-0.30543261909900765, "Vertical angle"=-0.006981317007977317, "Echo pulse width"=124, "Reserved"=0}, {"flags"=4, "Echo"=2, "Radial distance"=25.73, "Horizontal angle"=-0.30543261909900765, "Vertical angle"=-0.006981317007977317, "Echo pulse width"=76, "Reserved"=0}, {"flags"=5, "Echo"=0, "Radial distance"=33.47, "Horizontal angle"=-0.3097959422289935, "Vertical angle"=0.00698131700797732, "Echo pulse width"=192, "Reserved"=0}, {"flags"=0, "Echo"=1, "Radial distance"=35.18, "Horizontal angle"=-0.3097959422289935, "Vertical angle"=0.00698131700797732, "Echo pulse width"=132, "Reserved"=50}, {"flags"=0, "Echo"=0, "Radial distance"=81.47, "Horizontal angle"=-0.3097959422289935, "Vertical angle"=0.020943951023931963, "Echo pulse width"=96, "Reserved"=53}, {"flags"=4, "Echo"=0, "Radial distance"=16.080000000000002, "Horizontal angle"=-0.3141592653589793, "Vertical angle"=-0.020943951023931952, "Echo pulse width"=180, "Reserved"=0}, {"flags"=5, "Echo"=0, "Radial distance"=18.080000000000002, "Horizontal angle"=-0.3141592653589793, "Vertical angle"=-0.006981317007977317, "Echo pulse width"=272, "Reserved"=0}, {"flags"=5, "Echo"=1, "Radial distance"=21.150000000000002, "Horizontal angle"=-0.3141592653589793, "Vertical angle"=-0.006981317007977317, "Echo pulse width"=112, "Reserved"=0}, {"flags"=4, "Echo"=2, "Radial distance"=31.16, "Horizontal angle"=-0.3141592653589793, "Vertical angle"=-0.006981317007977317, "Echo pulse width"=88, "Reserved"=0}, {"flags"=1, "Echo"=0, "Radial distance"=30.3, "Horizontal angle"=-0.31852258848896514, "Vertical angle"=0.00698131700797732, "Echo pulse width"=172, "Reserved"=54}, {"flags"=4, "Echo"=1, "Radial distance"=33.27, "Horizontal angle"=-0.31852258848896514, "Vertical angle"=0.00698131700797732, "Echo pulse width"=104, "Reserved"=0}, {"flags"=1, "Echo"=0, "Radial distance"=30.21, "Horizontal angle"=-0.31852258848896514, "Vertical angle"=0.020943951023931963, "Echo pulse width"=136, "Reserved"=54}, {"flags"=5, "Echo"=1, "Radial distance"=34.26, "Horizontal angle"=-0.31852258848896514, "Vertical angle"=0.020943951023931963, "Echo pulse width"=80, "Reserved"=0}, {"flags"=0, "Echo"=2, "Radial distance"=83.43, "Horizontal angle"=-0.31852258848896514, "Vertical angle"=0.020943951023931963, "Echo pulse width"=112, "Reserved"=55}, {"flags"=4, "Echo"=0, "Radial distance"=15.67, "Horizontal angle"=-0.32288591161895097, "Vertical angle"=-0.020943951023931952, "Echo pulse width"=184, "Reserved"=0}, {"flags"=5, "Echo"=0, "Radial distance"=17.68, "Horizontal angle"=-0.32288591161895097, "Vertical angle"=-0.006981317007977317, "Echo pulse width"=312, "Reserved"=0}, {"flags"=5, "Echo"=1, "Radial distance"=20.95, "Horizontal angle"=-0.32288591161895097, "Vertical angle"=-0.006981317007977317, "Echo pulse width"=80, "Reserved"=0}, {"flags"=4, "Echo"=2, "Radial distance"=24.71, "Horizontal angle"=-0.32288591161895097, "Vertical angle"=-0.006981317007977317, "Echo pulse width"=84, "Reserved"=0}, {"flags"=0, "Echo"=0, "Radial distance"=30.07, "Horizontal angle"=-0.3272492347489368, "Vertical angle"=0.00698131700797732, "Echo pulse width"=180, "Reserved"=54}, {"flags"=1, "Echo"=0, "Radial distance"=30.080000000000002, "Horizontal angle"=-0.3272492347489368, "Vertical angle"=0.020943951023931963, "Echo pulse width"=168, "Reserved"=54}, {"flags"=0, "Echo"=1, "Radial distance"=63.910000000000004, "Horizontal angle"=-0.3272492347489368, "Vertical angle"=0.020943951023931963, "Echo pulse width"=112, "Reserved"=56}, {"flags"=4, "Echo"=0, "Radial distance"=15.31, "Horizontal angle"=-0.33161255787892263, "Vertical angle"=-0.020943951023931952, "Echo pulse width"=192, "Reserved"=0}, {"flags"=5, "Echo"=0, "Radial distance"=17.8, "Horizontal angle"=-0.33161255787892263, "Vertical angle"=-0.006981317007977317, "Echo pulse width"=292, "Reserved"=0}, {"flags"=5, "Echo"=1, "Radial distance"=20.87, "Horizontal angle"=-0.33161255787892263, "Vertical angle"=-0.006981317007977317, "Echo pulse width"=44, "Reserved"=0}, {"flags"=4, "Echo"=2, "Radial distance"=24.88, "Horizontal angle"=-0.33161255787892263, "Vertical angle"=-0.006981317007977317, "Echo pulse width"=92, "Reserved"=0}, {"flags"=0, "Echo"=0, "Radial distance"=29.98, "Horizontal angle"=-0.3359758810089084, "Vertical angle"=0.00698131700797732, "Echo pulse width"=172, "Reserved"=54}, {"flags"=1, "Echo"=0, "Radial distance"=30.04, "Horizontal angle"=-0.3359758810089084, "Vertical angle"=0.020943951023931963, "Echo pulse width"=172, "Reserved"=54}, {"flags"=0, "Echo"=1, "Radial distance"=82.82000000000001, "Horizontal angle"=-0.3359758810089084, "Vertical angle"=0.020943951023931963, "Echo pulse width"=104, "Reserved"=57}, {"flags"=4, "Echo"=0, "Radial distance"=14.93, "Horizontal angle"=-0.3403392041388943, "Vertical angle"=-0.020943951023931952, "Echo pulse width"=208, "Reserved"=0}, {"flags"=5, "Echo"=0, "Radial distance"=17.44, "Horizontal angle"=-0.3403392041388943, "Vertical angle"=-0.006981317007977317, "Echo pulse width"=312, "Reserved"=0}, {"flags"=5, "Echo"=1, "Radial distance"=24.6, "Horizontal angle"=-0.3403392041388943, "Vertical angle"=-0.006981317007977317, "Echo pulse width"=36, "Reserved"=0}, {"flags"=4, "Echo"=2, "Radial distance"=28.55, "Horizontal angle"=-0.3403392041388943, "Vertical angle"=-0.006981317007977317, "Echo pulse width"=120, "Reserved"=0}, {"flags"=0, "Echo"=0, "Radial distance"=30.11, "Horizontal angle"=-0.34470252726888007, "Vertical angle"=0.00698131700797732, "Echo pulse width"=176, "Reserved"=54}, {"flags"=0, "Echo"=0, "Radial distance"=30.11, "Horizontal angle"=-0.34470252726888007, "Vertical angle"=0.020943951023931963, "Echo pulse width"=160, "Reserved"=54}, {"flags"=4, "Echo"=0, "Radial distance"=14.55, "Horizontal angle"=-0.3490658503988659, "Vertical angle"=-0.020943951023931952, "Echo pulse width"=228, "Reserved"=0}, {"flags"=5, "Echo"=0, "Radial distance"=16.85, "Horizontal angle"=-0.3490658503988659, "Vertical angle"=-0.006981317007977317, "Echo pulse width"=336, "Reserved"=0}, {"flags"=4, "Echo"=1, "Radial distance"=27.68, "Horizontal angle"=-0.3490658503988659, "Vertical angle"=-0.006981317007977317, "Echo pulse width"=128, "Reserved"=0}, {"flags"=1, "Echo"=0, "Radial distance"=30.38, "Horizontal angle"=-0.3534291735288517, "Vertical angle"=0.00698131700797732, "Echo pulse width"=164, "Reserved"=54}, {"flags"=4, "Echo"=1, "Radial distance"=31.77, "Horizontal angle"=-0.3534291735288517, "Vertical angle"=0.00698131700797732, "Echo pulse width"=88, "Reserved"=0}, {"flags"=1, "Echo"=0, "Radial distance"=30.43, "Horizontal angle"=-0.3534291735288517, "Vertical angle"=0.020943951023931963, "Echo pulse width"=116, "Reserved"=54}, {"flags"=0, "Echo"=1, "Radial distance"=84.26, "Horizontal angle"=-0.3534291735288517, "Vertical angle"=0.020943951023931963, "Echo pulse width"=92, "Reserved"=58}, {"flags"=4, "Echo"=0, "Radial distance"=14.200000000000001, "Horizontal angle"=-0.35779249665883756, "Vertical angle"=-0.020943951023931952, "Echo pulse width"=220, "Reserved"=0}, {"flags"=5, "Echo"=0, "Radial distance"=16.81, "Horizontal angle"=-0.35779249665883756, "Vertical angle"=-0.006981317007977317, "Echo pulse width"=388, "Reserved"=0}, {"flags"=0, "Echo"=1, "Radial distance"=26.76, "Horizontal angle"=-0.35779249665883756, "Vertical angle"=-0.006981317007977317, "Echo pulse width"=132, "Reserved"=59}, {"flags"=1, "Echo"=0, "Radial distance"=27.01, "Horizontal angle"=-0.3621558197888234, "Vertical angle"=0.00698131700797732, "Echo pulse width"=120, "Reserved"=59}, {"flags"=4, "Echo"=1, "Radial distance"=31.62, "Horizontal angle"=-0.3621558197888234, "Vertical angle"=0.00698131700797732, "Echo pulse width"=132, "Reserved"=0}, {"flags"=4, "Echo"=0, "Radial distance"=13.790000000000001, "Horizontal angle"=-0.3665191429188092, "Vertical angle"=-0.020943951023931952, "Echo pulse width"=248, "Reserved"=0}, {"flags"=5, "Echo"=0, "Radial distance"=16.73, "Horizontal angle"=-0.3665191429188092, "Vertical angle"=-0.006981317007977317, "Echo pulse width"=360, "Reserved"=0}, {"flags"=4, "Echo"=1, "Radial distance"=26.240000000000002, "Horizontal angle"=-0.3665191429188092, "Vertical angle"=-0.006981317007977317, "Echo pulse width"=128, "Reserved"=0}, {"flags"=0, "Echo"=0, "Radial distance"=25.43, "Horizontal angle"=-0.370882466048795, "Vertical angle"=0.00698131700797732, "Echo pulse width"=192, "Reserved"=60}, {"flags"=1, "Echo"=0, "Radial distance"=25.310000000000002, "Horizontal angle"=-0.370882466048795, "Vertical angle"=0.020943951023931963, "Echo pulse width"=160, "Reserved"=60}, {"flags"=0, "Echo"=1, "Radial distance"=95.93, "Horizontal angle"=-0.370882466048795, "Vertical angle"=0.020943951023931963, "Echo pulse width"=36, "Reserved"=61}, {"flags"=4, "Echo"=0, "Radial distance"=13.51, "Horizontal angle"=-0.3752457891787809, "Vertical angle"=-0.020943951023931952, "Echo pulse width"=240, "Reserved"=0}, {"flags"=5, "Echo"=0, "Radial distance"=16.41, "Horizontal angle"=-0.3752457891787809, "Vertical angle"=-0.006981317007977317, "Echo pulse width"=364, "Reserved"=0}, {"flags"=0, "Echo"=1, "Radial distance"=25.55, "Horizontal angle"=-0.3752457891787809, "Vertical angle"=-0.006981317007977317, "Echo pulse width"=124, "Reserved"=60}, {"flags"=0, "Echo"=0, "Radial distance"=25.19, "Horizontal angle"=-0.37960911230876665, "Vertical angle"=0.00698131700797732, "Echo pulse width"=180, "Reserved"=60}, {"flags"=1, "Echo"=0, "Radial distance"=25.21, "Horizontal angle"=-0.37960911230876665, "Vertical angle"=0.020943951023931963, "Echo pulse width"=184, "Reserved"=60}, {"flags"=0, "Echo"=1, "Radial distance"=29.01, "Horizontal angle"=-0.37960911230876665, "Vertical angle"=0.020943951023931963, "Echo pulse width"=136, "Reserved"=62}, {"flags"=4, "Echo"=0, "Radial distance"=13.11, "Horizontal angle"=-0.3839724354387525, "Vertical angle"=-0.020943951023931952, "Echo pulse width"=272, "Reserved"=0}, {"flags"=5, "Echo"=0, "Radial distance"=16.09, "Horizontal angle"=-0.3839724354387525, "Vertical angle"=-0.006981317007977317, "Echo pulse width"=372, "Reserved"=0}, {"flags"=0, "Echo"=1, "Radial distance"=24.76, "Horizontal angle"=-0.3839724354387525, "Vertical angle"=-0.006981317007977317, "Echo pulse width"=136, "Reserved"=60}, {"flags"=0, "Echo"=0, "Radial distance"=25.11, "Horizontal angle"=-0.3883357585687383, "Vertical angle"=0.00698131700797732, "Echo pulse width"=176, "Reserved"=60}, {"flags"=1, "Echo"=0, "Radial distance"=25.13, "Horizontal angle"=-0.3883357585687383, "Vertical angle"=0.020943951023931963, "Echo pulse width"=188, "Reserved"=60}, {"flags"=0, "Echo"=1, "Radial distance"=29.09, "Horizontal angle"=-0.3883357585687383, "Vertical angle"=0.020943951023931963, "Echo pulse width"=136, "Reserved"=62}, {"flags"=4, "Echo"=0, "Radial distance"=12.91, "Horizontal angle"=-0.39269908169872414, "Vertical angle"=-0.020943951023931952, "Echo pulse width"=276, "Reserved"=0}, {"flags"=5, "Echo"=0, "Radial distance"=15.88, "Horizontal angle"=-0.39269908169872414, "Vertical angle"=-0.006981317007977317, "Echo pulse width"=216, "Reserved"=0}, {"flags"=5, "Echo"=1, "Radial distance"=18.09, "Horizontal angle"=-0.39269908169872414, "Vertical angle"=-0.006981317007977317, "Echo pulse width"=152, "Reserved"=0}, {"flags"=4, "Echo"=2, "Radial distance"=24.32, "Horizontal angle"=-0.39269908169872414, "Vertical angle"=-0.006981317007977317, "Echo pulse width"=136, "Reserved"=0}, {"flags"=0, "Echo"=0, "Radial distance"=25.150000000000002, "Horizontal angle"=-0.39706240482870997, "Vertical angle"=0.00698131700797732, "Echo pulse width"=192, "Reserved"=60}, {"flags"=1, "Echo"=0, "Radial distance"=25.17, "Horizontal angle"=-0.39706240482870997, "Vertical angle"=0.020943951023931963, "Echo pulse width"=184, "Reserved"=60}, {"flags"=0, "Echo"=1, "Radial distance"=29.14, "Horizontal angle"=-0.39706240482870997, "Vertical angle"=0.020943951023931963, "Echo pulse width"=144, "Reserved"=62}, {"flags"=4, "Echo"=0, "Radial distance"=12.55, "Horizontal angle"=-0.40142572795869574, "Vertical angle"=-0.020943951023931952, "Echo pulse width"=300, "Reserved"=0}, {"flags"=5, "Echo"=0, "Radial distance"=15.780000000000001, "Horizontal angle"=-0.40142572795869574, "Vertical angle"=-0.006981317007977317, "Echo pulse width"=212, "Reserved"=0}, {"flags"=5, "Echo"=1, "Radial distance"=17.85, "Horizontal angle"=-0.40142572795869574, "Vertical angle"=-0.006981317007977317, "Echo pulse width"=148, "Reserved"=0}, {"flags"=4, "Echo"=2, "Radial distance"=23.85, "Horizontal angle"=-0.40142572795869574, "Vertical angle"=-0.006981317007977317, "Echo pulse width"=144, "Reserved"=0}, {"flags"=0, "Echo"=0, "Radial distance"=25.19, "Horizontal angle"=-0.40578905108868163, "Vertical angle"=0.00698131700797732, "Echo pulse width"=196, "Reserved"=60}, {"flags"=0, "Echo"=0, "Radial distance"=25.44, "Horizontal angle"=-0.40578905108868163, "Vertical angle"=0.020943951023931963, "Echo pulse width"=288, "Reserved"=60}, {"flags"=4, "Echo"=0, "Radial distance"=12.31, "Horizontal angle"=-0.41015237421866746, "Vertical angle"=-0.020943951023931952, "Echo pulse width"=304, "Reserved"=0}, {"flags"=5, "Echo"=0, "Radial distance"=15.530000000000001, "Horizontal angle"=-0.41015237421866746, "Vertical angle"=-0.006981317007977317, "Echo pulse width"=232, "Reserved"=0}, {"flags"=5, "Echo"=1, "Radial distance"=18.35, "Horizontal angle"=-0.41015237421866746, "Vertical angle"=-0.006981317007977317, "Echo pulse width"=204, "Reserved"=0}, {"flags"=4, "Echo"=2, "Radial distance"=23.41, "Horizontal angle"=-0.41015237421866746, "Vertical angle"=-0.006981317007977317, "Echo pulse width"=152, "Reserved"=0}, {"flags"=1, "Echo"=0, "Radial distance"=25.150000000000002, "Horizontal angle"=-0.4145156973486533, "Vertical angle"=0.00698131700797732, "Echo pulse width"=284, "Reserved"=60}, {"flags"=4, "Echo"=1, "Radial distance"=42.410000000000004, "Horizontal angle"=-0.4145156973486533, "Vertical angle"=0.00698131700797732, "Echo pulse width"=156, "Reserved"=0}, {"flags"=1, "Echo"=0, "Radial distance"=61.690000000000005, "Horizontal angle"=-0.4145156973486533, "Vertical angle"=0.020943951023931963, "Echo pulse width"=64, "Reserved"=63}, {"flags"=0, "Echo"=1, "Radial distance"=83.67, "Horizontal angle"=-0.4145156973486533, "Vertical angle"=0.020943951023931963, "Echo pulse width"=100, "Reserved"=64}, {"flags"=4, "Echo"=0, "Radial distance"=12.030000000000001, "Horizontal angle"=-0.41887902047863906, "Vertical angle"=-0.020943951023931952, "Echo pulse width"=260, "Reserved"=0}, {"flags"=5, "Echo"=0, "Radial distance"=15.24, "Horizontal angle"=-0.41887902047863906, "Vertical angle"=-0.006981317007977317, "Echo pulse width"=256, "Reserved"=0}, {"flags"=5, "Echo"=1, "Radial distance"=18.18, "Horizontal angle"=-0.41887902047863906, "Vertical angle"=-0.006981317007977317, "Echo pulse width"=212, "Reserved"=0}, {"flags"=4, "Echo"=2, "Radial distance"=22.73, "Horizontal angle"=-0.41887902047863906, "Vertical angle"=-0.006981317007977317, "Echo pulse width"=144, "Reserved"=0}, {"flags"=5, "Echo"=0, "Radial distance"=25.150000000000002, "Horizontal angle"=-0.4232423436086249, "Vertical angle"=0.00698131700797732, "Echo pulse width"=260, "Reserved"=0}, {"flags"=5, "Echo"=1, "Radial distance"=29.25, "Horizontal angle"=-0.4232423436086249, "Vertical angle"=0.00698131700797732, "Echo pulse width"=92, "Reserved"=0}, {"flags"=4, "Echo"=2, "Radial distance"=42.46, "Horizontal angle"=-0.4232423436086249, "Vertical angle"=0.00698131700797732, "Echo pulse width"=164, "Reserved"=0}, {"flags"=4, "Echo"=0, "Radial distance"=44.550000000000004, "Horizontal angle"=-0.4232423436086249, "Vertical angle"=0.020943951023931963, "Echo pulse width"=164, "Reserved"=0}, {"flags"=4, "Echo"=0, "Radial distance"=11.86, "Horizontal angle"=-0.42760566673861067, "Vertical angle"=-0.020943951023931952, "Echo pulse width"=224, "Reserved"=0}, {"flags"=5, "Echo"=0, "Radial distance"=15.120000000000001, "Horizontal angle"=-0.42760566673861067, "Vertical angle"=-0.006981317007977317, "Echo pulse width"=276, "Reserved"=0}, {"flags"=5, "Echo"=1, "Radial distance"=18.28, "Horizontal angle"=-0.42760566673861067, "Vertical angle"=-0.006981317007977317, "Echo pulse width"=136, "Reserved"=0}, {"flags"=4, "Echo"=2, "Radial distance"=22.29, "Horizontal angle"=-0.42760566673861067, "Vertical angle"=-0.006981317007977317, "Echo pulse width"=148, "Reserved"=0}, {"flags"=5, "Echo"=0, "Radial distance"=24.990000000000002, "Horizontal angle"=-0.4319689898685966, "Vertical angle"=0.00698131700797732, "Echo pulse width"=256, "Reserved"=0}, {"flags"=5, "Echo"=1, "Radial distance"=32.85, "Horizontal angle"=-0.4319689898685966, "Vertical angle"=0.00698131700797732, "Echo pulse width"=92, "Reserved"=0}, {"flags"=4, "Echo"=2, "Radial distance"=42.54, "Horizontal angle"=-0.4319689898685966, "Vertical angle"=0.00698131700797732, "Echo pulse width"=160, "Reserved"=0}, {"flags"=4, "Echo"=0, "Radial distance"=11.55, "Horizontal angle"=-0.4363323129985824, "Vertical angle"=-0.020943951023931952, "Echo pulse width"=260, "Reserved"=0}, {"flags"=0, "Echo"=0, "Radial distance"=12.5, "Horizontal angle"=-0.4363323129985824, "Vertical angle"=-0.006981317007977317, "Echo pulse width"=160, "Reserved"=65}, {"flags"=0, "Echo"=0, "Radial distance"=12.450000000000001, "Horizontal angle"=-0.4406956361285682, "Vertical angle"=0.00698131700797732, "Echo pulse width"=156, "Reserved"=65}, {"flags"=0, "Echo"=0, "Radial distance"=12.47, "Horizontal angle"=-0.4406956361285682, "Vertical angle"=0.020943951023931963, "Echo pulse width"=160, "Reserved"=65}, {"flags"=4, "Echo"=0, "Radial distance"=11.51, "Horizontal angle"=-0.445058959258554, "Vertical angle"=-0.020943951023931952, "Echo pulse width"=248, "Reserved"=0}, {"flags"=0, "Echo"=0, "Radial distance"=12.48, "Horizontal angle"=-0.445058959258554, "Vertical angle"=-0.006981317007977317, "Echo pulse width"=148, "Reserved"=65}, {"flags"=0, "Echo"=0, "Radial distance"=12.5, "Horizontal angle"=-0.4494222823885398, "Vertical angle"=0.00698131700797732, "Echo pulse width"=96, "Reserved"=65}, {"flags"=0, "Echo"=0, "Radial distance"=12.44, "Horizontal angle"=-0.4494222823885398, "Vertical angle"=0.020943951023931963, "Echo pulse width"=104, "Reserved"=65}, {"flags"=4, "Echo"=0, "Radial distance"=11.15, "Horizontal angle"=-0.45378560551852565, "Vertical angle"=-0.020943951023931952, "Echo pulse width"=308, "Reserved"=0}, {"flags"=1, "Echo"=0, "Radial distance"=12.6, "Horizontal angle"=-0.45378560551852565, "Vertical angle"=-0.006981317007977317, "Echo pulse width"=128, "Reserved"=65}, {"flags"=5, "Echo"=1, "Radial distance"=15.76, "Horizontal angle"=-0.45378560551852565, "Vertical angle"=-0.006981317007977317, "Echo pulse width"=272, "Reserved"=0}, {"flags"=4, "Echo"=2, "Radial distance"=18.59, "Horizontal angle"=-0.45378560551852565, "Vertical angle"=-0.006981317007977317, "Echo pulse width"=124, "Reserved"=0}, {"flags"=0, "Echo"=0, "Radial distance"=20.79, "Horizontal angle"=-0.45814892864851153, "Vertical angle"=0.00698131700797732, "Echo pulse width"=192, "Reserved"=66}, {"flags"=0, "Echo"=0, "Radial distance"=20.57, "Horizontal angle"=-0.45814892864851153, "Vertical angle"=0.020943951023931963, "Echo pulse width"=184, "Reserved"=66}, {"flags"=4, "Echo"=0, "Radial distance"=11.15, "Horizontal angle"=-0.4625122517784973, "Vertical angle"=-0.020943951023931952, "Echo pulse width"=288, "Reserved"=0}, {"flags"=5, "Echo"=0, "Radial distance"=14.96, "Horizontal angle"=-0.4625122517784973, "Vertical angle"=-0.006981317007977317, "Echo pulse width"=288, "Reserved"=0}, {"flags"=5, "Echo"=1, "Radial distance"=18.31, "Horizontal angle"=-0.4625122517784973, "Vertical angle"=-0.006981317007977317, "Echo pulse width"=80, "Reserved"=0}, {"flags"=0, "Echo"=2, "Radial distance"=20.45, "Horizontal angle"=-0.4625122517784973, "Vertical angle"=-0.006981317007977317, "Echo pulse width"=144, "Reserved"=66}, {"flags"=0, "Echo"=0, "Radial distance"=20.6, "Horizontal angle"=-0.46687557490848314, "Vertical angle"=0.00698131700797732, "Echo pulse width"=184, "Reserved"=66}, {"flags"=0, "Echo"=0, "Radial distance"=20.400000000000002, "Horizontal angle"=-0.46687557490848314, "Vertical angle"=0.020943951023931963, "Echo pulse width"=180, "Reserved"=66}, {"flags"=4, "Echo"=0, "Radial distance"=10.89, "Horizontal angle"=-0.47123889803846897, "Vertical angle"=-0.020943951023931952, "Echo pulse width"=348, "Reserved"=0}, {"flags"=5, "Echo"=0, "Radial distance"=14.290000000000001, "Horizontal angle"=-0.47123889803846897, "Vertical angle"=-0.006981317007977317, "Echo pulse width"=344, "Reserved"=0}, {"flags"=5, "Echo"=1, "Radial distance"=18.11, "Horizontal angle"=-0.47123889803846897, "Vertical angle"=-0.006981317007977317, "Echo pulse width"=64, "Reserved"=0}, {"flags"=4, "Echo"=2, "Radial distance"=20.09, "Horizontal angle"=-0.47123889803846897, "Vertical angle"=-0.006981317007977317, "Echo pulse width"=152, "Reserved"=0}, {"flags"=0, "Echo"=0, "Radial distance"=20.48, "Horizontal angle"=-0.47560222116845474, "Vertical angle"=0.00698131700797732, "Echo pulse width"=184, "Reserved"=66}, {"flags"=0, "Echo"=0, "Radial distance"=20.400000000000002, "Horizontal angle"=-0.47560222116845474, "Vertical angle"=0.020943951023931963, "Echo pulse width"=180, "Reserved"=66}, {"flags"=4, "Echo"=0, "Radial distance"=10.950000000000001, "Horizontal angle"=-0.4799655442984406, "Vertical angle"=-0.020943951023931952, "Echo pulse width"=288, "Reserved"=0}, {"flags"=5, "Echo"=0, "Radial distance"=14.88, "Horizontal angle"=-0.4799655442984406, "Vertical angle"=-0.006981317007977317, "Echo pulse width"=280, "Reserved"=0}, {"flags"=5, "Echo"=1, "Radial distance"=16.87, "Horizontal angle"=-0.4799655442984406, "Vertical angle"=-0.006981317007977317, "Echo pulse width"=44, "Reserved"=0}, {"flags"=4, "Echo"=2, "Radial distance"=17.93, "Horizontal angle"=-0.4799655442984406, "Vertical angle"=-0.006981317007977317, "Echo pulse width"=48, "Reserved"=0}, {"flags"=0, "Echo"=0, "Radial distance"=20.5, "Horizontal angle"=-0.48432886742842646, "Vertical angle"=0.00698131700797732, "Echo pulse width"=200, "Reserved"=66}, {"flags"=0, "Echo"=0, "Radial distance"=20.400000000000002, "Horizontal angle"=-0.48432886742842646, "Vertical angle"=0.020943951023931963, "Echo pulse width"=180, "Reserved"=66}, {"flags"=4, "Echo"=0, "Radial distance"=10.69, "Horizontal angle"=-0.4886921905584123, "Vertical angle"=-0.020943951023931952, "Echo pulse width"=344, "Reserved"=0}, {"flags"=5, "Echo"=0, "Radial distance"=14.09, "Horizontal angle"=-0.4886921905584123, "Vertical angle"=-0.006981317007977317, "Echo pulse width"=404, "Reserved"=0}, {"flags"=4, "Echo"=1, "Radial distance"=19.37, "Horizontal angle"=-0.4886921905584123, "Vertical angle"=-0.006981317007977317, "Echo pulse width"=152, "Reserved"=0}, {"flags"=0, "Echo"=0, "Radial distance"=20.38, "Horizontal angle"=-0.49305551368839806, "Vertical angle"=0.00698131700797732, "Echo pulse width"=240, "Reserved"=66}, {"flags"=0, "Echo"=0, "Radial distance"=20.52, "Horizontal angle"=-0.49305551368839806, "Vertical angle"=0.020943951023931963, "Echo pulse width"=176, "Reserved"=66}, {"flags"=4, "Echo"=0, "Radial distance"=10.790000000000001, "Horizontal angle"=-0.4974188368183839, "Vertical angle"=-0.020943951023931952, "Echo pulse width"=288, "Reserved"=0}, {"flags"=5, "Echo"=0, "Radial distance"=14.55, "Horizontal angle"=-0.4974188368183839, "Vertical angle"=-0.006981317007977317, "Echo pulse width"=328, "Reserved"=0}, {"flags"=4, "Echo"=1, "Radial distance"=19.01, "Horizontal angle"=-0.4974188368183839, "Vertical angle"=-0.006981317007977317, "Echo pulse width"=156, "Reserved"=0}, {"flags"=5, "Echo"=0, "Radial distance"=20.11, "Horizontal angle"=-0.5017821599483697, "Vertical angle"=0.00698131700797732, "Echo pulse width"=344, "Reserved"=0}, {"flags"=5, "Echo"=1, "Radial distance"=24.560000000000002, "Horizontal angle"=-0.5017821599483697, "Vertical angle"=0.00698131700797732, "Echo pulse width"=80, "Reserved"=0}, {"flags"=4, "Echo"=2, "Radial distance"=30.28, "Horizontal angle"=-0.5017821599483697, "Vertical angle"=0.00698131700797732, "Echo pulse width"=188, "Reserved"=0}, {"flags"=5, "Echo"=0, "Radial distance"=20.84, "Horizontal angle"=-0.5017821599483697, "Vertical angle"=0.020943951023931963, "Echo pulse width"=168, "Reserved"=0}, {"flags"=5, "Echo"=1, "Radial distance"=31.61, "Horizontal angle"=-0.5017821599483697, "Vertical angle"=0.020943951023931963, "Echo pulse width"=76, "Reserved"=0}, {"flags"=4, "Echo"=2, "Radial distance"=33.15, "Horizontal angle"=-0.5017821599483697, "Vertical angle"=0.020943951023931963, "Echo pulse width"=112, "Reserved"=0}, {"flags"=4, "Echo"=0, "Radial distance"=10.53, "Horizontal angle"=-0.5061454830783556, "Vertical angle"=-0.020943951023931952, "Echo pulse width"=344, "Reserved"=0}, {"flags"=5, "Echo"=0, "Radial distance"=13.85, "Horizontal angle"=-0.5061454830783556, "Vertical angle"=-0.006981317007977317, "Echo pulse width"=452, "Reserved"=0}, {"flags"=4, "Echo"=1, "Radial distance"=18.650000000000002, "Horizontal angle"=-0.5061454830783556, "Vertical angle"=-0.006981317007977317, "Echo pulse width"=156, "Reserved"=0}, {"flags"=5, "Echo"=0, "Radial distance"=19.55, "Horizontal angle"=-0.5105088062083414, "Vertical angle"=0.00698131700797732, "Echo pulse width"=176, "Reserved"=0}, {"flags"=5, "Echo"=1, "Radial distance"=21.330000000000002, "Horizontal angle"=-0.5105088062083414, "Vertical angle"=0.00698131700797732, "Echo pulse width"=88, "Reserved"=0}, {"flags"=4, "Echo"=2, "Radial distance"=23.81, "Horizontal angle"=-0.5105088062083414, "Vertical angle"=0.00698131700797732, "Echo pulse width"=120, "Reserved"=0}, {"flags"=4, "Echo"=0, "Radial distance"=31.68, "Horizontal angle"=-0.5105088062083414, "Vertical angle"=0.020943951023931963, "Echo pulse width"=220, "Reserved"=0}, {"flags"=4, "Echo"=0, "Radial distance"=10.51, "Horizontal angle"=-0.5148721293383272, "Vertical angle"=-0.020943951023931952, "Echo pulse width"=288, "Reserved"=0}, {"flags"=5, "Echo"=0, "Radial distance"=14.280000000000001, "Horizontal angle"=-0.5148721293383272, "Vertical angle"=-0.006981317007977317, "Echo pulse width"=364, "Reserved"=0}, {"flags"=4, "Echo"=1, "Radial distance"=18.37, "Horizontal angle"=-0.5148721293383272, "Vertical angle"=-0.006981317007977317, "Echo pulse width"=148, "Reserved"=0}, {"flags"=5, "Echo"=0, "Radial distance"=19.23, "Horizontal angle"=-0.519235452468313, "Vertical angle"=0.00698131700797732, "Echo pulse width"=192, "Reserved"=0}, {"flags"=5, "Echo"=1, "Radial distance"=23.71, "Horizontal angle"=-0.519235452468313, "Vertical angle"=0.00698131700797732, "Echo pulse width"=140, "Reserved"=0}, {"flags"=4, "Echo"=2, "Radial distance"=30.400000000000002, "Horizontal angle"=-0.519235452468313, "Vertical angle"=0.00698131700797732, "Echo pulse width"=188, "Reserved"=0}, {"flags"=4, "Echo"=0, "Radial distance"=31.64, "Horizontal angle"=-0.519235452468313, "Vertical angle"=0.020943951023931963, "Echo pulse width"=216, "Reserved"=0}, {"flags"=4, "Echo"=0, "Radial distance"=10.31, "Horizontal angle"=-0.5235987755982988, "Vertical angle"=-0.020943951023931952, "Echo pulse width"=340, "Reserved"=0}, {"flags"=5, "Echo"=0, "Radial distance"=13.57, "Horizontal angle"=-0.5235987755982988, "Vertical angle"=-0.006981317007977317, "Echo pulse width"=428, "Reserved"=0}, {"flags"=4, "Echo"=1, "Radial distance"=18.05, "Horizontal angle"=-0.5235987755982988, "Vertical angle"=-0.006981317007977317, "Echo pulse width"=156, "Reserved"=0}, {"flags"=5, "Echo"=0, "Radial distance"=18.88, "Horizontal angle"=-0.5279620987282847, "Vertical angle"=0.00698131700797732, "Echo pulse width"=228, "Reserved"=0}, {"flags"=5, "Echo"=1, "Radial distance"=23.35, "Horizontal angle"=-0.5279620987282847, "Vertical angle"=0.00698131700797732, "Echo pulse width"=104, "Reserved"=0}, {"flags"=4, "Echo"=2, "Radial distance"=30.34, "Horizontal angle"=-0.5279620987282847, "Vertical angle"=0.00698131700797732, "Echo pulse width"=204, "Reserved"=0}, {"flags"=4, "Echo"=0, "Radial distance"=31.66, "Horizontal angle"=-0.5279620987282847, "Vertical angle"=0.020943951023931963, "Echo pulse width"=212, "Reserved"=0}, {"flags"=4, "Echo"=0, "Radial distance"=10.39, "Horizontal angle"=-0.5323254218582705, "Vertical angle"=-0.020943951023931952, "Echo pulse width"=288, "Reserved"=0}, {"flags"=5, "Echo"=0, "Radial distance"=14.51, "Horizontal angle"=-0.5323254218582705, "Vertical angle"=-0.006981317007977317, "Echo pulse width"=316, "Reserved"=0}, {"flags"=4, "Echo"=1, "Radial distance"=17.66, "Horizontal angle"=-0.5323254218582705, "Vertical angle"=-0.006981317007977317, "Echo pulse width"=164, "Reserved"=0}, {"flags"=5, "Echo"=0, "Radial distance"=18.67, "Horizontal angle"=-0.5366887449882564, "Vertical angle"=0.00698131700797732, "Echo pulse width"=248, "Reserved"=0}, {"flags"=4, "Echo"=1, "Radial distance"=30.51, "Horizontal angle"=-0.5366887449882564, "Vertical angle"=0.00698131700797732, "Echo pulse width"=176, "Reserved"=0}, {"flags"=5, "Echo"=0, "Radial distance"=31.76, "Horizontal angle"=-0.5366887449882564, "Vertical angle"=0.020943951023931963, "Echo pulse width"=200, "Reserved"=0}, {"flags"=4, "Echo"=1, "Radial distance"=41.42, "Horizontal angle"=-0.5366887449882564, "Vertical angle"=0.020943951023931963, "Echo pulse width"=84, "Reserved"=0}, {"flags"=4, "Echo"=0, "Radial distance"=10.13, "Horizontal angle"=-0.5410520681182421, "Vertical angle"=-0.020943951023931952, "Echo pulse width"=348, "Reserved"=0}, {"flags"=4, "Echo"=0, "Radial distance"=13.49, "Horizontal angle"=-0.5410520681182421, "Vertical angle"=-0.006981317007977317, "Echo pulse width"=576, "Reserved"=0}, {"flags"=5, "Echo"=0, "Radial distance"=18.43, "Horizontal angle"=-0.5454153912482279, "Vertical angle"=0.00698131700797732, "Echo pulse width"=252, "Reserved"=0}, {"flags"=4, "Echo"=1, "Radial distance"=30.55, "Horizontal angle"=-0.5454153912482279, "Vertical angle"=0.00698131700797732, "Echo pulse width"=176, "Reserved"=0}, {"flags"=5, "Echo"=0, "Radial distance"=31.92, "Horizontal angle"=-0.5454153912482279, "Vertical angle"=0.020943951023931963, "Echo pulse width"=204, "Reserved"=0}, {"flags"=4, "Echo"=1, "Radial distance"=41.480000000000004, "Horizontal angle"=-0.5454153912482279, "Vertical angle"=0.020943951023931963, "Echo pulse width"=124, "Reserved"=0}, {"flags"=4, "Echo"=0, "Radial distance"=10.19, "Horizontal angle"=-0.5497787143782138, "Vertical angle"=-0.020943951023931952, "Echo pulse width"=296, "Reserved"=0}, {"flags"=4, "Echo"=0, "Radial distance"=14.120000000000001, "Horizontal angle"=-0.5497787143782138, "Vertical angle"=-0.006981317007977317, "Echo pulse width"=480, "Reserved"=0}, {"flags"=5, "Echo"=0, "Radial distance"=18.31, "Horizontal angle"=-0.5541420375081997, "Vertical angle"=0.00698131700797732, "Echo pulse width"=252, "Reserved"=0}, {"flags"=4, "Echo"=1, "Radial distance"=30.84, "Horizontal angle"=-0.5541420375081997, "Vertical angle"=0.00698131700797732, "Echo pulse width"=148, "Reserved"=0}, {"flags"=5, "Echo"=0, "Radial distance"=32.19, "Horizontal angle"=-0.5541420375081997, "Vertical angle"=0.020943951023931963, "Echo pulse width"=156, "Reserved"=0}, {"flags"=4, "Echo"=1, "Radial distance"=40.42, "Horizontal angle"=-0.5541420375081997, "Vertical angle"=0.020943951023931963, "Echo pulse width"=108, "Reserved"=0}, {"flags"=4, "Echo"=0, "Radial distance"=10.01, "Horizontal angle"=-0.5585053606381855, "Vertical angle"=-0.020943951023931952, "Echo pulse width"=344, "Reserved"=0}, {"flags"=5, "Echo"=0, "Radial distance"=13.17, "Horizontal angle"=-0.5585053606381855, "Vertical angle"=-0.006981317007977317, "Echo pulse width"=380, "Reserved"=0}, {"flags"=4, "Echo"=1, "Radial distance"=16.94, "Horizontal angle"=-0.5585053606381855, "Vertical angle"=-0.006981317007977317, "Echo pulse width"=160, "Reserved"=0}, {"flags"=4, "Echo"=0, "Radial distance"=16.67, "Horizontal angle"=-0.5628686837681712, "Vertical angle"=0.00698131700797732, "Echo pulse width"=364, "Reserved"=0}, {"flags"=0, "Echo"=0, "Radial distance"=16.37, "Horizontal angle"=-0.5628686837681712, "Vertical angle"=0.020943951023931963, "Echo pulse width"=188, "Reserved"=67}, {"flags"=4, "Echo"=0, "Radial distance"=10.19, "Horizontal angle"=-0.5672320068981571, "Vertical angle"=-0.020943951023931952, "Echo pulse width"=284, "Reserved"=0}, {"flags"=4, "Echo"=0, "Radial distance"=13.64, "Horizontal angle"=-0.5672320068981571, "Vertical angle"=-0.006981317007977317, "Echo pulse width"=476, "Reserved"=0}, {"flags"=0, "Echo"=0, "Radial distance"=16.39, "Horizontal angle"=-0.5715953300281429, "Vertical angle"=0.00698131700797732, "Echo pulse width"=196, "Reserved"=67}, {"flags"=0, "Echo"=0, "Radial distance"=16.17, "Horizontal angle"=-0.5715953300281429, "Vertical angle"=0.020943951023931963, "Echo pulse width"=188, "Reserved"=67}, {"flags"=4, "Echo"=0, "Radial distance"=9.99, "Horizontal angle"=-0.5759586531581287, "Vertical angle"=-0.020943951023931952, "Echo pulse width"=336, "Reserved"=0}, {"flags"=5, "Echo"=0, "Radial distance"=13.05, "Horizontal angle"=-0.5759586531581287, "Vertical angle"=-0.006981317007977317, "Echo pulse width"=336, "Reserved"=0}, {"flags"=0, "Echo"=1, "Radial distance"=16.38, "Horizontal angle"=-0.5759586531581287, "Vertical angle"=-0.006981317007977317, "Echo pulse width"=160, "Reserved"=67}, {"flags"=0, "Echo"=0, "Radial distance"=16.23, "Horizontal angle"=-0.5803219762881145, "Vertical angle"=0.00698131700797732, "Echo pulse width"=192, "Reserved"=67}, {"flags"=0, "Echo"=0, "Radial distance"=16.01, "Horizontal angle"=-0.5803219762881145, "Vertical angle"=0.020943951023931963, "Echo pulse width"=184, "Reserved"=67}, {"flags"=4, "Echo"=0, "Radial distance"=9.99, "Horizontal angle"=-0.5846852994181004, "Vertical angle"=-0.020943951023931952, "Echo pulse width"=288, "Reserved"=0}, {"flags"=4, "Echo"=0, "Radial distance"=13.32, "Horizontal angle"=-0.5846852994181004, "Vertical angle"=-0.006981317007977317, "Echo pulse width"=460, "Reserved"=0}, {"flags"=0, "Echo"=0, "Radial distance"=16.240000000000002, "Horizontal angle"=-0.5890486225480862, "Vertical angle"=0.00698131700797732, "Echo pulse width"=188, "Reserved"=67}, {"flags"=0, "Echo"=0, "Radial distance"=15.97, "Horizontal angle"=-0.5890486225480862, "Vertical angle"=0.020943951023931963, "Echo pulse width"=188, "Reserved"=67}, {"flags"=4, "Echo"=0, "Radial distance"=9.77, "Horizontal angle"=-0.593411945678072, "Vertical angle"=-0.020943951023931952, "Echo pulse width"=344, "Reserved"=0}, {"flags"=4, "Echo"=0, "Radial distance"=12.81, "Horizontal angle"=-0.593411945678072, "Vertical angle"=-0.006981317007977317, "Echo pulse width"=492, "Reserved"=0}, {"flags"=0, "Echo"=0, "Radial distance"=16.16, "Horizontal angle"=-0.5977752688080579, "Vertical angle"=0.00698131700797732, "Echo pulse width"=184, "Reserved"=67}, {"flags"=0, "Echo"=0, "Radial distance"=15.97, "Horizontal angle"=-0.5977752688080579, "Vertical angle"=0.020943951023931963, "Echo pulse width"=188, "Reserved"=67}, {"flags"=4, "Echo"=0, "Radial distance"=9.83, "Horizontal angle"=-0.6021385919380438, "Vertical angle"=-0.020943951023931952, "Echo pulse width"=284, "Reserved"=0}, {"flags"=4, "Echo"=0, "Radial distance"=12.96, "Horizontal angle"=-0.6021385919380438, "Vertical angle"=-0.006981317007977317, "Echo pulse width"=456, "Reserved"=0}, {"flags"=0, "Echo"=0, "Radial distance"=16.23, "Horizontal angle"=-0.6065019150680295, "Vertical angle"=0.00698131700797732, "Echo pulse width"=192, "Reserved"=67}, {"flags"=0, "Echo"=0, "Radial distance"=16.05, "Horizontal angle"=-0.6065019150680295, "Vertical angle"=0.020943951023931963, "Echo pulse width"=188, "Reserved"=67}, {"flags"=4, "Echo"=0, "Radial distance"=9.67, "Horizontal angle"=-0.6108652381980153, "Vertical angle"=-0.020943951023931952, "Echo pulse width"=340, "Reserved"=0}, {"flags"=4, "Echo"=0, "Radial distance"=12.69, "Horizontal angle"=-0.6108652381980153, "Vertical angle"=-0.006981317007977317, "Echo pulse width"=480, "Reserved"=0}, {"flags"=0, "Echo"=0, "Radial distance"=16.240000000000002, "Horizontal angle"=-0.6152285613280012, "Vertical angle"=0.00698131700797732, "Echo pulse width"=188, "Reserved"=67}, {"flags"=0, "Echo"=0, "Radial distance"=16.04, "Horizontal angle"=-0.6152285613280012, "Vertical angle"=0.020943951023931963, "Echo pulse width"=180, "Reserved"=67}, {"flags"=4, "Echo"=0, "Radial distance"=9.790000000000001, "Horizontal angle"=-0.619591884457987, "Vertical angle"=-0.020943951023931952, "Echo pulse width"=284, "Reserved"=0}, {"flags"=4, "Echo"=0, "Radial distance"=12.84, "Horizontal angle"=-0.619591884457987, "Vertical angle"=-0.006981317007977317, "Echo pulse width"=440, "Reserved"=0}, {"flags"=0, "Echo"=0, "Radial distance"=16.39, "Horizontal angle"=-0.6239552075879727, "Vertical angle"=0.00698131700797732, "Echo pulse width"=192, "Reserved"=67}, {"flags"=0, "Echo"=0, "Radial distance"=16.17, "Horizontal angle"=-0.6239552075879727, "Vertical angle"=0.020943951023931963, "Echo pulse width"=184, "Reserved"=67}, {"flags"=4, "Echo"=0, "Radial distance"=9.59, "Horizontal angle"=-0.6283185307179586, "Vertical angle"=-0.020943951023931952, "Echo pulse width"=340, "Reserved"=0}, {"flags"=4, "Echo"=0, "Radial distance"=12.61, "Horizontal angle"=-0.6283185307179586, "Vertical angle"=-0.006981317007977317, "Echo pulse width"=468, "Reserved"=0}, {"flags"=5, "Echo"=0, "Radial distance"=17.150000000000002, "Horizontal angle"=-0.6326818538479445, "Vertical angle"=0.00698131700797732, "Echo pulse width"=380, "Reserved"=0}, {"flags"=4, "Echo"=1, "Radial distance"=26.13, "Horizontal angle"=-0.6326818538479445, "Vertical angle"=0.00698131700797732, "Echo pulse width"=88, "Reserved"=0}, {"flags"=0, "Echo"=0, "Radial distance"=16.36, "Horizontal angle"=-0.6326818538479445, "Vertical angle"=0.020943951023931963, "Echo pulse width"=180, "Reserved"=67}, {"flags"=4, "Echo"=0, "Radial distance"=9.67, "Horizontal angle"=-0.6370451769779303, "Vertical angle"=-0.020943951023931952, "Echo pulse width"=300, "Reserved"=0}, {"flags"=4, "Echo"=0, "Radial distance"=12.72, "Horizontal angle"=-0.6370451769779303, "Vertical angle"=-0.006981317007977317, "Echo pulse width"=432, "Reserved"=0}, {"flags"=5, "Echo"=0, "Radial distance"=16.990000000000002, "Horizontal angle"=-0.6414085001079161, "Vertical angle"=0.00698131700797732, "Echo pulse width"=288, "Reserved"=0}, {"flags"=4, "Echo"=1, "Radial distance"=25.72, "Horizontal angle"=-0.6414085001079161, "Vertical angle"=0.00698131700797732, "Echo pulse width"=60, "Reserved"=0}, {"flags"=4, "Echo"=0, "Radial distance"=9.450000000000001, "Horizontal angle"=-0.6457718232379019, "Vertical angle"=-0.020943951023931952, "Echo pulse width"=352, "Reserved"=0}, {"flags"=4, "Echo"=0, "Radial distance"=12.49, "Horizontal angle"=-0.6457718232379019, "Vertical angle"=-0.006981317007977317, "Echo pulse width"=456, "Reserved"=0}, {"flags"=5, "Echo"=0, "Radial distance"=16.87, "Horizontal angle"=-0.6501351463678877, "Vertical angle"=0.00698131700797732, "Echo pulse width"=384, "Reserved"=0}, {"flags"=5, "Echo"=1, "Radial distance"=25.48, "Horizontal angle"=-0.6501351463678877, "Vertical angle"=0.00698131700797732, "Echo pulse width"=68, "Reserved"=0}, {"flags"=4, "Echo"=2, "Radial distance"=26.84, "Horizontal angle"=-0.6501351463678877, "Vertical angle"=0.00698131700797732, "Echo pulse width"=84, "Reserved"=0}, {"flags"=4, "Echo"=0, "Radial distance"=9.55, "Horizontal angle"=-0.6544984694978736, "Vertical angle"=-0.020943951023931952, "Echo pulse width"=300, "Reserved"=0}, {"flags"=4, "Echo"=0, "Radial distance"=12.64, "Horizontal angle"=-0.6544984694978736, "Vertical angle"=-0.006981317007977317, "Echo pulse width"=424, "Reserved"=0}, {"flags"=4, "Echo"=0, "Radial distance"=16.55, "Horizontal angle"=-0.6588617926278594, "Vertical angle"=0.00698131700797732, "Echo pulse width"=424, "Reserved"=0}, {"flags"=4, "Echo"=0, "Radial distance"=9.33, "Horizontal angle"=-0.6632251157578453, "Vertical angle"=-0.020943951023931952, "Echo pulse width"=352, "Reserved"=0}, {"flags"=4, "Echo"=0, "Radial distance"=12.290000000000001, "Horizontal angle"=-0.6632251157578453, "Vertical angle"=-0.006981317007977317, "Echo pulse width"=448, "Reserved"=0}, {"flags"=4, "Echo"=0, "Radial distance"=16.55, "Horizontal angle"=-0.667588438887831, "Vertical angle"=0.00698131700797732, "Echo pulse width"=396, "Reserved"=0}, {"flags"=0, "Echo"=0, "Radial distance"=76.51, "Horizontal angle"=-0.667588438887831, "Vertical angle"=0.020943951023931963, "Echo pulse width"=96, "Reserved"=68}, {"flags"=4, "Echo"=0, "Radial distance"=9.47, "Horizontal angle"=-0.6719517620178168, "Vertical angle"=-0.020943951023931952, "Echo pulse width"=296, "Reserved"=0}, {"flags"=4, "Echo"=0, "Radial distance"=12.48, "Horizontal angle"=-0.6719517620178168, "Vertical angle"=-0.006981317007977317, "Echo pulse width"=396, "Reserved"=0}, {"flags"=4, "Echo"=0, "Radial distance"=16.31, "Horizontal angle"=-0.6763150851478027, "Vertical angle"=0.00698131700797732, "Echo pulse width"=388, "Reserved"=0}, {"flags"=0, "Echo"=0, "Radial distance"=84.49, "Horizontal angle"=-0.6763150851478027, "Vertical angle"=0.020943951023931963, "Echo pulse width"=72, "Reserved"=69}, {"flags"=4, "Echo"=0, "Radial distance"=9.290000000000001, "Horizontal angle"=-0.6806784082777886, "Vertical angle"=-0.020943951023931952, "Echo pulse width"=344, "Reserved"=0}, {"flags"=4, "Echo"=0, "Radial distance"=12.25, "Horizontal angle"=-0.6806784082777886, "Vertical angle"=-0.006981317007977317, "Echo pulse width"=424, "Reserved"=0}, {"flags"=4, "Echo"=0, "Radial distance"=15.99, "Horizontal angle"=-0.6850417314077744, "Vertical angle"=0.00698131700797732, "Echo pulse width"=432, "Reserved"=0}, {"flags"=4, "Echo"=0, "Radial distance"=9.35, "Horizontal angle"=-0.6894050545377601, "Vertical angle"=-0.020943951023931952, "Echo pulse width"=296, "Reserved"=0}, {"flags"=4, "Echo"=0, "Radial distance"=12.48, "Horizontal angle"=-0.6894050545377601, "Vertical angle"=-0.006981317007977317, "Echo pulse width"=380, "Reserved"=0}, {"flags"=5, "Echo"=0, "Radial distance"=15.870000000000001, "Horizontal angle"=-0.6937683776677459, "Vertical angle"=0.00698131700797732, "Echo pulse width"=400, "Reserved"=0}, {"flags"=4, "Echo"=1, "Radial distance"=21.39, "Horizontal angle"=-0.6937683776677459, "Vertical angle"=0.00698131700797732, "Echo pulse width"=108, "Reserved"=0}, {"flags"=4, "Echo"=0, "Radial distance"=9.19, "Horizontal angle"=-0.6981317007977318, "Vertical angle"=-0.020943951023931952, "Echo pulse width"=332, "Reserved"=0}, {"flags"=4, "Echo"=0, "Radial distance"=12.09, "Horizontal angle"=-0.6981317007977318, "Vertical angle"=-0.006981317007977317, "Echo pulse width"=416, "Reserved"=0}, {"flags"=4, "Echo"=0, "Radial distance"=15.75, "Horizontal angle"=-0.7024950239277177, "Vertical angle"=0.00698131700797732, "Echo pulse width"=412, "Reserved"=0}, {"flags"=4, "Echo"=0, "Radial distance"=9.19, "Horizontal angle"=-0.7068583470577035, "Vertical angle"=-0.020943951023931952, "Echo pulse width"=292, "Reserved"=0}, {"flags"=4, "Echo"=0, "Radial distance"=12.24, "Horizontal angle"=-0.7068583470577035, "Vertical angle"=-0.006981317007977317, "Echo pulse width"=372, "Reserved"=0}, {"flags"=5, "Echo"=0, "Radial distance"=15.67, "Horizontal angle"=-0.7112216701876892, "Vertical angle"=0.00698131700797732, "Echo pulse width"=384, "Reserved"=0}, {"flags"=5, "Echo"=1, "Radial distance"=21.22, "Horizontal angle"=-0.7112216701876892, "Vertical angle"=0.00698131700797732, "Echo pulse width"=36, "Reserved"=0}, {"flags"=4, "Echo"=2, "Radial distance"=25.09, "Horizontal angle"=-0.7112216701876892, "Vertical angle"=0.00698131700797732, "Echo pulse width"=112, "Reserved"=0}, {"flags"=4, "Echo"=0, "Radial distance"=9.07, "Horizontal angle"=-0.7155849933176751, "Vertical angle"=-0.020943951023931952, "Echo pulse width"=332, "Reserved"=0}, {"flags"=4, "Echo"=0, "Radial distance"=11.85, "Horizontal angle"=-0.7155849933176751, "Vertical angle"=-0.006981317007977317, "Echo pulse width"=412, "Reserved"=0}, {"flags"=5, "Echo"=0, "Radial distance"=15.39, "Horizontal angle"=-0.7199483164476609, "Vertical angle"=0.00698131700797732, "Echo pulse width"=352, "Reserved"=0}, {"flags"=4, "Echo"=1, "Radial distance"=24.77, "Horizontal angle"=-0.7199483164476609, "Vertical angle"=0.00698131700797732, "Echo pulse width"=156, "Reserved"=0}, {"flags"=4, "Echo"=0, "Radial distance"=25.89, "Horizontal angle"=-0.7199483164476609, "Vertical angle"=0.020943951023931963, "Echo pulse width"=72, "Reserved"=0}, {"flags"=4, "Echo"=0, "Radial distance"=9.07, "Horizontal angle"=-0.7243116395776468, "Vertical angle"=-0.020943951023931952, "Echo pulse width"=288, "Reserved"=0}, {"flags"=4, "Echo"=0, "Radial distance"=12.120000000000001, "Horizontal angle"=-0.7243116395776468, "Vertical angle"=-0.006981317007977317, "Echo pulse width"=360, "Reserved"=0}, {"flags"=5, "Echo"=0, "Radial distance"=15.11, "Horizontal angle"=-0.7286749627076325, "Vertical angle"=0.00698131700797732, "Echo pulse width"=376, "Reserved"=0}, {"flags"=5, "Echo"=1, "Radial distance"=21.26, "Horizontal angle"=-0.7286749627076325, "Vertical angle"=0.00698131700797732, "Echo pulse width"=36, "Reserved"=0}, {"flags"=4, "Echo"=2, "Radial distance"=24.35, "Horizontal angle"=-0.7286749627076325, "Vertical angle"=0.00698131700797732, "Echo pulse width"=136, "Reserved"=0}, {"flags"=4, "Echo"=0, "Radial distance"=25.76, "Horizontal angle"=-0.7286749627076325, "Vertical angle"=0.020943951023931963, "Echo pulse width"=192, "Reserved"=0}, {"flags"=4, "Echo"=0, "Radial distance"=8.950000000000001, "Horizontal angle"=-0.7330382858376184, "Vertical angle"=-0.020943951023931952, "Echo pulse width"=332, "Reserved"=0}, {"flags"=4, "Echo"=0, "Radial distance"=11.85, "Horizontal angle"=-0.7330382858376184, "Vertical angle"=-0.006981317007977317, "Echo pulse width"=392, "Reserved"=0}, {"flags"=5, "Echo"=0, "Radial distance"=15.15, "Horizontal angle"=-0.7374016089676042, "Vertical angle"=0.00698131700797732, "Echo pulse width"=368, "Reserved"=0}, {"flags"=5, "Echo"=1, "Radial distance"=19.61, "Horizontal angle"=-0.7374016089676042, "Vertical angle"=0.00698131700797732, "Echo pulse width"=92, "Reserved"=0}, {"flags"=4, "Echo"=2, "Radial distance"=24.13, "Horizontal angle"=-0.7374016089676042, "Vertical angle"=0.00698131700797732, "Echo pulse width"=124, "Reserved"=0}, {"flags"=4, "Echo"=0, "Radial distance"=25.240000000000002, "Horizontal angle"=-0.7374016089676042, "Vertical angle"=0.020943951023931963, "Echo pulse width"=252, "Reserved"=0}, {"flags"=4, "Echo"=0, "Radial distance"=8.950000000000001, "Horizontal angle"=-0.74176493209759, "Vertical angle"=-0.020943951023931952, "Echo pulse width"=284, "Reserved"=0}, {"flags"=4, "Echo"=0, "Radial distance"=11.92, "Horizontal angle"=-0.74176493209759, "Vertical angle"=-0.006981317007977317, "Echo pulse width"=348, "Reserved"=0}, {"flags"=5, "Echo"=0, "Radial distance"=14.870000000000001, "Horizontal angle"=-0.7461282552275759, "Vertical angle"=0.00698131700797732, "Echo pulse width"=376, "Reserved"=0}, {"flags"=5, "Echo"=1, "Radial distance"=19.37, "Horizontal angle"=-0.7461282552275759, "Vertical angle"=0.00698131700797732, "Echo pulse width"=124, "Reserved"=0}, {"flags"=4, "Echo"=2, "Radial distance"=23.97, "Horizontal angle"=-0.7461282552275759, "Vertical angle"=0.00698131700797732, "Echo pulse width"=120, "Reserved"=0}, {"flags"=4, "Echo"=0, "Radial distance"=24.92, "Horizontal angle"=-0.7461282552275759, "Vertical angle"=0.020943951023931963, "Echo pulse width"=276, "Reserved"=0}, {"flags"=4, "Echo"=0, "Radial distance"=8.83, "Horizontal angle"=-0.7504915783575618, "Vertical angle"=-0.020943951023931952, "Echo pulse width"=324, "Reserved"=0}, {"flags"=4, "Echo"=0, "Radial distance"=11.65, "Horizontal angle"=-0.7504915783575618, "Vertical angle"=-0.006981317007977317, "Echo pulse width"=368, "Reserved"=0}, {"flags"=5, "Echo"=0, "Radial distance"=14.790000000000001, "Horizontal angle"=-0.7548549014875475, "Vertical angle"=0.00698131700797732, "Echo pulse width"=392, "Reserved"=0}, {"flags"=5, "Echo"=1, "Radial distance"=19.07, "Horizontal angle"=-0.7548549014875475, "Vertical angle"=0.00698131700797732, "Echo pulse width"=104, "Reserved"=0}, {"flags"=4, "Echo"=2, "Radial distance"=23.75, "Horizontal angle"=-0.7548549014875475, "Vertical angle"=0.00698131700797732, "Echo pulse width"=108, "Reserved"=0}, {"flags"=4, "Echo"=0, "Radial distance"=24.63, "Horizontal angle"=-0.7548549014875475, "Vertical angle"=0.020943951023931963, "Echo pulse width"=236, "Reserved"=0}, {"flags"=4, "Echo"=0, "Radial distance"=8.870000000000001, "Horizontal angle"=-0.7592182246175333, "Vertical angle"=-0.020943951023931952, "Echo pulse width"=280, "Reserved"=0}, {"flags"=4, "Echo"=0, "Radial distance"=11.790000000000001, "Horizontal angle"=-0.7592182246175333, "Vertical angle"=-0.006981317007977317, "Echo pulse width"=296, "Reserved"=0}, {"flags"=5, "Echo"=0, "Radial distance"=14.64, "Horizontal angle"=-0.7635815477475192, "Vertical angle"=0.00698131700797732, "Echo pulse width"=352, "Reserved"=0}, {"flags"=5, "Echo"=1, "Radial distance"=19.36, "Horizontal angle"=-0.7635815477475192, "Vertical angle"=0.00698131700797732, "Echo pulse width"=208, "Reserved"=0}, {"flags"=4, "Echo"=2, "Radial distance"=23.62, "Horizontal angle"=-0.7635815477475192, "Vertical angle"=0.00698131700797732, "Echo pulse width"=100, "Reserved"=0}, {"flags"=1, "Echo"=0, "Radial distance"=12.46, "Horizontal angle"=-0.7635815477475192, "Vertical angle"=0.020943951023931963, "Echo pulse width"=140, "Reserved"=70}, {"flags"=4, "Echo"=1, "Radial distance"=24.11, "Horizontal angle"=-0.7635815477475192, "Vertical angle"=0.020943951023931963, "Echo pulse width"=160, "Reserved"=0}, {"flags"=4, "Echo"=0, "Radial distance"=8.71, "Horizontal angle"=-0.767944870877505, "Vertical angle"=-0.020943951023931952, "Echo pulse width"=328, "Reserved"=0}, {"flags"=4, "Echo"=0, "Radial distance"=11.48, "Horizontal angle"=-0.767944870877505, "Vertical angle"=-0.006981317007977317, "Echo pulse width"=320, "Reserved"=0}, {"flags"=1, "Echo"=0, "Radial distance"=12.43, "Horizontal angle"=-0.7723081940074907, "Vertical angle"=0.00698131700797732, "Echo pulse width"=196, "Reserved"=70}, {"flags"=4, "Echo"=1, "Radial distance"=16.14, "Horizontal angle"=-0.7723081940074907, "Vertical angle"=0.00698131700797732, "Echo pulse width"=100, "Reserved"=0}, {"flags"=0, "Echo"=0, "Radial distance"=12.25, "Horizontal angle"=-0.7723081940074907, "Vertical angle"=0.020943951023931963, "Echo pulse width"=188, "Reserved"=70}, {"flags"=4, "Echo"=0, "Radial distance"=8.870000000000001, "Horizontal angle"=-0.7766715171374766, "Vertical angle"=-0.020943951023931952, "Echo pulse width"=276, "Reserved"=0}, {"flags"=4, "Echo"=0, "Radial distance"=11.790000000000001, "Horizontal angle"=-0.7766715171374766, "Vertical angle"=-0.006981317007977317, "Echo pulse width"=256, "Reserved"=0}, {"flags"=0, "Echo"=0, "Radial distance"=12.33, "Horizontal angle"=-0.7810348402674625, "Vertical angle"=0.00698131700797732, "Echo pulse width"=168, "Reserved"=70}, {"flags"=0, "Echo"=0, "Radial distance"=12.15, "Horizontal angle"=-0.7810348402674625, "Vertical angle"=0.020943951023931963, "Echo pulse width"=164, "Reserved"=70}, {"flags"=4, "Echo"=0, "Radial distance"=8.59, "Horizontal angle"=-0.7853981633974483, "Vertical angle"=-0.020943951023931952, "Echo pulse width"=332, "Reserved"=0}, {"flags"=4, "Echo"=0, "Radial distance"=11.32, "Horizontal angle"=-0.7853981633974483, "Vertical angle"=-0.006981317007977317, "Echo pulse width"=304, "Reserved"=0}, {"flags"=0, "Echo"=0, "Radial distance"=12.27, "Horizontal angle"=-0.789761486527434, "Vertical angle"=0.00698131700797732, "Echo pulse width"=192, "Reserved"=70}, {"flags"=0, "Echo"=0, "Radial distance"=12.08, "Horizontal angle"=-0.789761486527434, "Vertical angle"=0.020943951023931963, "Echo pulse width"=192, "Reserved"=70}, {"flags"=4, "Echo"=0, "Radial distance"=8.67, "Horizontal angle"=-0.7941248096574199, "Vertical angle"=-0.020943951023931952, "Echo pulse width"=276, "Reserved"=0}, {"flags"=4, "Echo"=0, "Radial distance"=11.5, "Horizontal angle"=-0.7941248096574199, "Vertical angle"=-0.006981317007977317, "Echo pulse width"=248, "Reserved"=0}, {"flags"=0, "Echo"=0, "Radial distance"=12.15, "Horizontal angle"=-0.7984881327874057, "Vertical angle"=0.00698131700797732, "Echo pulse width"=164, "Reserved"=70}, {"flags"=0, "Echo"=0, "Radial distance"=11.99, "Horizontal angle"=-0.7984881327874057, "Vertical angle"=0.020943951023931963, "Echo pulse width"=168, "Reserved"=70}, {"flags"=4, "Echo"=0, "Radial distance"=8.47, "Horizontal angle"=-0.8028514559173915, "Vertical angle"=-0.020943951023931952, "Echo pulse width"=324, "Reserved"=0}, {"flags"=4, "Echo"=0, "Radial distance"=11.16, "Horizontal angle"=-0.8028514559173915, "Vertical angle"=-0.006981317007977317, "Echo pulse width"=284, "Reserved"=0}, {"flags"=0, "Echo"=0, "Radial distance"=12.11, "Horizontal angle"=-0.8072147790473774, "Vertical angle"=0.00698131700797732, "Echo pulse width"=192, "Reserved"=70}, {"flags"=0, "Echo"=0, "Radial distance"=11.89, "Horizontal angle"=-0.8072147790473774, "Vertical angle"=0.020943951023931963, "Echo pulse width"=188, "Reserved"=70}, {"flags"=4, "Echo"=0, "Radial distance"=8.63, "Horizontal angle"=-0.8115781021773633, "Vertical angle"=-0.020943951023931952, "Echo pulse width"=276, "Reserved"=0}, {"flags"=4, "Echo"=0, "Radial distance"=11.33, "Horizontal angle"=-0.8115781021773633, "Vertical angle"=-0.006981317007977317, "Echo pulse width"=236, "Reserved"=0}, {"flags"=0, "Echo"=0, "Radial distance"=12.07, "Horizontal angle"=-0.8159414253073491, "Vertical angle"=0.00698131700797732, "Echo pulse width"=164, "Reserved"=70}, {"flags"=0, "Echo"=0, "Radial distance"=11.870000000000001, "Horizontal angle"=-0.8159414253073491, "Vertical angle"=0.020943951023931963, "Echo pulse width"=160, "Reserved"=70}, {"flags"=4, "Echo"=0, "Radial distance"=8.47, "Horizontal angle"=-0.8203047484373349, "Vertical angle"=-0.020943951023931952, "Echo pulse width"=312, "Reserved"=0}, {"flags"=4, "Echo"=0, "Radial distance"=11.120000000000001, "Horizontal angle"=-0.8203047484373349, "Vertical angle"=-0.006981317007977317, "Echo pulse width"=264, "Reserved"=0}, {"flags"=0, "Echo"=0, "Radial distance"=11.96, "Horizontal angle"=-0.8246680715673207, "Vertical angle"=0.00698131700797732, "Echo pulse width"=184, "Reserved"=70}, {"flags"=0, "Echo"=0, "Radial distance"=11.92, "Horizontal angle"=-0.8246680715673207, "Vertical angle"=0.020943951023931963, "Echo pulse width"=200, "Reserved"=70}, {"flags"=4, "Echo"=0, "Radial distance"=8.59, "Horizontal angle"=-0.8290313946973066, "Vertical angle"=-0.020943951023931952, "Echo pulse width"=264, "Reserved"=0}, {"flags"=4, "Echo"=0, "Radial distance"=11.33, "Horizontal angle"=-0.8290313946973066, "Vertical angle"=-0.006981317007977317, "Echo pulse width"=220, "Reserved"=0}, {"flags"=0, "Echo"=0, "Radial distance"=12.030000000000001, "Horizontal angle"=-0.8333947178272924, "Vertical angle"=0.00698131700797732, "Echo pulse width"=164, "Reserved"=70}, {"flags"=0, "Echo"=0, "Radial distance"=11.870000000000001, "Horizontal angle"=-0.8333947178272924, "Vertical angle"=0.020943951023931963, "Echo pulse width"=160, "Reserved"=70}, {"flags"=4, "Echo"=0, "Radial distance"=8.43, "Horizontal angle"=-0.8377580409572781, "Vertical angle"=-0.020943951023931952, "Echo pulse width"=304, "Reserved"=0}, {"flags"=4, "Echo"=0, "Radial distance"=11.0, "Horizontal angle"=-0.8377580409572781, "Vertical angle"=-0.006981317007977317, "Echo pulse width"=256, "Reserved"=0}, {"flags"=0, "Echo"=0, "Radial distance"=12.040000000000001, "Horizontal angle"=-0.842121364087264, "Vertical angle"=0.00698131700797732, "Echo pulse width"=184, "Reserved"=70}, {"flags"=0, "Echo"=0, "Radial distance"=11.89, "Horizontal angle"=-0.842121364087264, "Vertical angle"=0.020943951023931963, "Echo pulse width"=188, "Reserved"=70}, {"flags"=4, "Echo"=0, "Radial distance"=8.51, "Horizontal angle"=-0.8464846872172498, "Vertical angle"=-0.020943951023931952, "Echo pulse width"=256, "Reserved"=0}, {"flags"=4, "Echo"=0, "Radial distance"=11.24, "Horizontal angle"=-0.8464846872172498, "Vertical angle"=-0.006981317007977317, "Echo pulse width"=212, "Reserved"=0}, {"flags"=0, "Echo"=0, "Radial distance"=12.09, "Horizontal angle"=-0.8508480103472356, "Vertical angle"=0.00698131700797732, "Echo pulse width"=168, "Reserved"=70}, {"flags"=0, "Echo"=0, "Radial distance"=11.91, "Horizontal angle"=-0.8508480103472356, "Vertical angle"=0.020943951023931963, "Echo pulse width"=164, "Reserved"=70}, {"flags"=4, "Echo"=0, "Radial distance"=8.31, "Horizontal angle"=-0.8552113334772213, "Vertical angle"=-0.020943951023931952, "Echo pulse width"=308, "Reserved"=0}, {"flags"=4, "Echo"=0, "Radial distance"=10.84, "Horizontal angle"=-0.8552113334772213, "Vertical angle"=-0.006981317007977317, "Echo pulse width"=264, "Reserved"=0}, {"flags"=0, "Echo"=0, "Radial distance"=12.14, "Horizontal angle"=-0.8595746566072073, "Vertical angle"=0.00698131700797732, "Echo pulse width"=200, "Reserved"=70}, {"flags"=0, "Echo"=0, "Radial distance"=11.97, "Horizontal angle"=-0.8595746566072073, "Vertical angle"=0.020943951023931963, "Echo pulse width"=184, "Reserved"=70}, {"flags"=4, "Echo"=0, "Radial distance"=8.51, "Horizontal angle"=-0.8639379797371932, "Vertical angle"=-0.020943951023931952, "Echo pulse width"=240, "Reserved"=0}, {"flags"=4, "Echo"=0, "Radial distance"=11.34, "Horizontal angle"=-0.8639379797371932, "Vertical angle"=-0.006981317007977317, "Echo pulse width"=176, "Reserved"=0}, {"flags"=0, "Echo"=0, "Radial distance"=12.290000000000001, "Horizontal angle"=-0.868301302867179, "Vertical angle"=0.00698131700797732, "Echo pulse width"=176, "Reserved"=70}, {"flags"=0, "Echo"=0, "Radial distance"=12.19, "Horizontal angle"=-0.868301302867179, "Vertical angle"=0.020943951023931963, "Echo pulse width"=160, "Reserved"=70}]} {"hash" format="%016x"}
  out "header":T9
  out "Ibeo error out":errorcluster
types:
  T1 = cluster{"hash":i64, "sys time":i64, "request":i32[]}
  T2 = cluster{"hash":i64, "sys time":i64, "type":u8, "raw":string}
  T3 = enum16{"Velodyne 16", "Velodyne 32", "Velodyne 64"}
  T4 = cluster{"hash":i64, "sys time":i64, "ref_vel":dbl, "ref_steer":dbl, "alert":u8}
  T5 = cluster{"hash":i64, "sys time":i64, "lat":dbl, "lon":dbl}
  T6 = cluster{"hash":i64, "sys time":i64, "n":u32, "pathxy":dbl[]}
  T7 = cluster{"hash":i64, "sys time":i64, "u time":i64, "alt":dbl}
  T8 = cluster{"hash":i64, "sys time":i64, "Header":cluster{"Size of prev messages":u32, "Size of this messages":u32, "Reserved":u8, "DeviceID":u8, "Data type":u16, "NTP time":u64}, "Scan header":cluster{"Scan number":u16, "scanner status":u16, "Sync phase offset":u16, "Scan start time NTP":u64, "Scan end time NTP":u64, "Angle ticks per rotation":u16, "Start angle":dbl, "End angle":dbl, "Scan points":u16, "pos_x":dbl, "pos_y":dbl, "pos_h":dbl, "Mounting position x":dbl, "Mounting position y":dbl, "Mounting position z":dbl, "Reserved":u16}, "Scan points":cluster{"flags":u8, "Echo":u8, "Radial distance":dbl, "Horizontal angle":dbl, "Vertical angle":dbl, "Echo pulse width":u16, "Reserved":u16}[]}
  T9 = cluster{"Size of prev messages":u32, "Size of this messages":u32, "Reserved":u8, "DeviceID":u8, "Data type":u16, "NTP time":u64}
  T10 = enum16{"big-endian, network order", "native, host order", "little-endian"}
  T11 = cluster{"connection ID":refnum<k16>, "net address":u32, "port":u16}
  T12 = cluster{"hash":i64, "sys time":i64, "time":dbl, "yaw_rate":dbl, "mdps torque":dbl, "mdps str_ang":dbl, "VS_CAN":dbl, "lat_accel":dbl, "mcp":dbl, "accel pedal value":dbl, "tps":dbl, "odometer":dbl, "battery voltage":dbl}
  T13 = cluster{"identifier":u32, "timestamp":timestamp, "payload":u8[]}
  T14 = cluster{"hash":i64, "sys time":i64, "Timestamp":u32, "Rot_ang":dbl[], "Ver_ang":dbl[], "Dist":dbl[], "Ver_off":dbl[], "Intensity":u8[], "pos x":dbl, "pos y":dbl, "Heading":dbl}
  T15 = cluster{"Laser block ID":u16, "Rotational position":u16}
  T16 = cluster{"hash":i64, "sys time":i64, "n":i32, "error":i32[]}
  T17 = cluster{"hash":i64, "sys time":i64, "status":i32, "TS_num":i32}
  T18 = cluster{"sys time":i64, "x":sgl, "y":sgl, "z":sgl}
  T19 = cluster{"Magic word":u32, "Size of prev messages":u32, "Size of this messages":u32, "Reserved":u8, "DeviceID":u8, "Data type":u16, "NTP time":u64}
  T20 = cluster{"command id":u16, "Reserved":u16, "parameter idx":u16}
  T21 = enum16{"Standard", "Buffered", "CRLF", "Immediate"}
  T22 = cluster{"hash":i64, "sys time":i64, "time":dbl, "yaw_rate":dbl, "mdps torque":dbl, "mdps str_ang":dbl, "VS_CAN":dbl, "lat_accel":dbl, "mcp":dbl, "accel pedal value":dbl, "tps":dbl, "odometer":dbl, "battery voltage":dbl, "WHL_SPD_RR":dbl, "WHL_SPD_RL":dbl, "WHL_SPD_FR":dbl, "WHL_SPD_FL":dbl}
  T23 = cluster{"hash":i64, "sys time":i64, "size":i32, "data":u8[]}
  T24 = cluster{"hash":i64, "sys time":i64, "Auto":bool, "Run":bool, "Solenoid":bool, "T lim":bool, "brk_enc":u8, "B PWM":u16, "T PWM":u16, "ref_vel":dbl, "ref_bkr_enc":dbl, "ref_apv":dbl, "ref_steer":dbl, "net address":u32}
  T25 = cluster{"hash":i64, "sys time":i64, "Auto":bool, "Run":bool, "Solenoid":bool, "T lim":bool, "brk_enc":u8, "B PWM":u16, "T PWM":u16, "ref_vel":dbl, "ref_bkr_enc":dbl, "ref_apv":dbl, "ref_steer":dbl}
  T26 = cluster{"hash":i64, "sys time":i64, "mobileye":u8[]}
  T27 = cluster{"hash":i64, "sys time":i64, "mobileye time":u32, "ID":u32, "data":u8[]}
  T28 = cluster{"hash":i64, "sys time":i64, "car time":u32, "ID":u32, "data":u8[]}
  T29 = cluster{"Scan number":u16, "scanner status":u16, "Sync phase offset":u16, "Scan start time NTP":u64, "Scan end time NTP":u64, "Angle ticks per rotation":u16, "Start angle":dbl, "End angle":dbl, "Scan points":u16, "pos_x":dbl, "pos_y":dbl, "pos_h":dbl, "Mounting position x":dbl, "Mounting position y":dbl, "Mounting position z":dbl, "Reserved":u16}
  T30 = cluster{"flags":u8, "Echo":u8, "Radial distance":dbl, "Horizontal angle":dbl, "Vertical angle":dbl, "Echo pulse width":u16, "Reserved":u16}[]
  T31 = cluster{"hash":i64, "sys time":i64, "Header":cluster{"Size of prev messages":u32, "Size of this messages":u32, "Reserved":u8, "DeviceID":u8, "Data type":u16, "NTP time":u64}, "Scan header":cluster{"Scan number":u16, "scanner status":u16, "Sync phase offset":u16, "Scan start time NTP":u64, "Scan end time NTP":u64, "Angle ticks per rotation":u16, "Start angle":dbl, "End angle":dbl, "Scan points":u16, "pos_x":dbl, "pos_y":dbl, "pos_h":dbl, "Mounting position x":dbl, "Mounting position y":dbl, "Mounting position z":dbl, "Reserved":u16}}
  T32 = cluster{"flags":u8, "Echo":u8, "Radial distance":dbl, "Horizontal angle":dbl, "Vertical angle":dbl, "Echo pulse width":u16, "Reserved":u16}
  T33 = cluster{"hash":i64, "sys time":i64, "Timestamp":u32, "Rotational angle":u16[], "dist":u16[][], "Intensity":u8[][], "pos_x":dbl, "pos_y":dbl, "pos_h":dbl}
  T34 = cluster{"hash":i64, "sys time":i64, "dt":dbl, "x":dbl, "y":dbl, "speed":dbl, "heading":dbl, "yaw_rate":dbl}
  T35 = cluster{"X":dbl[], "Y":dbl[], "Z":dbl[], "d":dbl[], "i":u8[]}
  T36 = cluster{"hash":i64, "sys time":i64, "model_no":i16, "n":i16, "SICK_FRONT_range":sgl[], "SICK_FRONT_intensity":sgl[]}
  T37 = cluster{"hash":i64, "sys time":i64, "n":i32, "data1":dbl[], "data2":dbl[], "lat":dbl[], "lon":dbl[]}
  T38 = cluster{"beep":bool, "duration (msec)":u32, "frequency (Hz)":u32}
  T39 = cluster{"hash":i64, "sys time":i64, "time":dbl, "x":dbl, "y":dbl, "h":dbl, "numSV":i32, "postype":i32, "lag":i32, "hordev":dbl, "lat":dbl, "lon":dbl, "hgt":dbl, "map_idx":i32}
  T40 = cluster{"hash":i64, "sys time":i64, "s_lat":dbl, "s_lon":dbl, "d_lat":dbl, "d_lon":dbl, "Message":i64}
  T41 = cluster{"hash":i64, "sys time":i64, "status":i32, "TS_num":i32, "TS_type":i32[], "TS_loc_x":dbl[], "TS_loc_y":dbl[]}
  T42 = cluster{"hash":i64, "sys time":i64, "left_lane_exist":bool, "right_lane_exist":bool, "left_lane_dot":dbl, "right_lane_dot":dbl}
  T43 = cluster{"hash":i64, "sys time":i64, "signal":i32, "sign":i32, "pedestrian":bool, "flag car":bool, "distance":dbl}
  T44 = cluster{"hash":i64, "sys time":i64, "size":i64, "x":dbl[], "y":dbl[], "point_flag":i32[]}
  T45 = cluster{"hash":i64, "sys time":i64, "stopline_exist":bool, "stopline_distance":dbl}
  T46 = cluster{"hash":i64, "sys time":i64, "time":dbl, "speed":dbl, "heading":dbl, "lat":dbl, "lon":dbl}
  T47 = cluster{"Scan number":u16, "scanner status":u16, "Sync phase offset":u16, "Scan start time NTP":u64, "Scan end time NTP":u64, "Angle ticks per rotation":u16, "Start angle":i16, "End angle":i16, "Scan points":u16, "Mounting position yaw angle ":i16, "Mounting position pitch angle":i16, "Mounting position roll angle":i16, "Mounting position x":i16, "Mounting position y":i16, "Mounting position z":i16, "Reserved":u16}
  T48 = cluster{"Scan number":u16, "scanner status":u16, "Sync phase offset":u16, "Scan start time NTP":u64, "Scan end time NTP":u64, "Angle ticks per rotation":u16, "Start angle":dbl, "End angle":dbl, "Scan points":u16, "Mounting position yaw angle ":dbl, "Mounting position pitch angle":dbl, "Mounting position roll angle":dbl, "Mounting position x":dbl, "Mounting position y":dbl, "Mounting position z":dbl, "Reserved":u16}
  T49 = cluster{"Layer/Echo":u8, "flags":u8, "Horizontal angle":i16, "Radial distance":u16, "Echo pulse width":u16, "Reserved":u16}
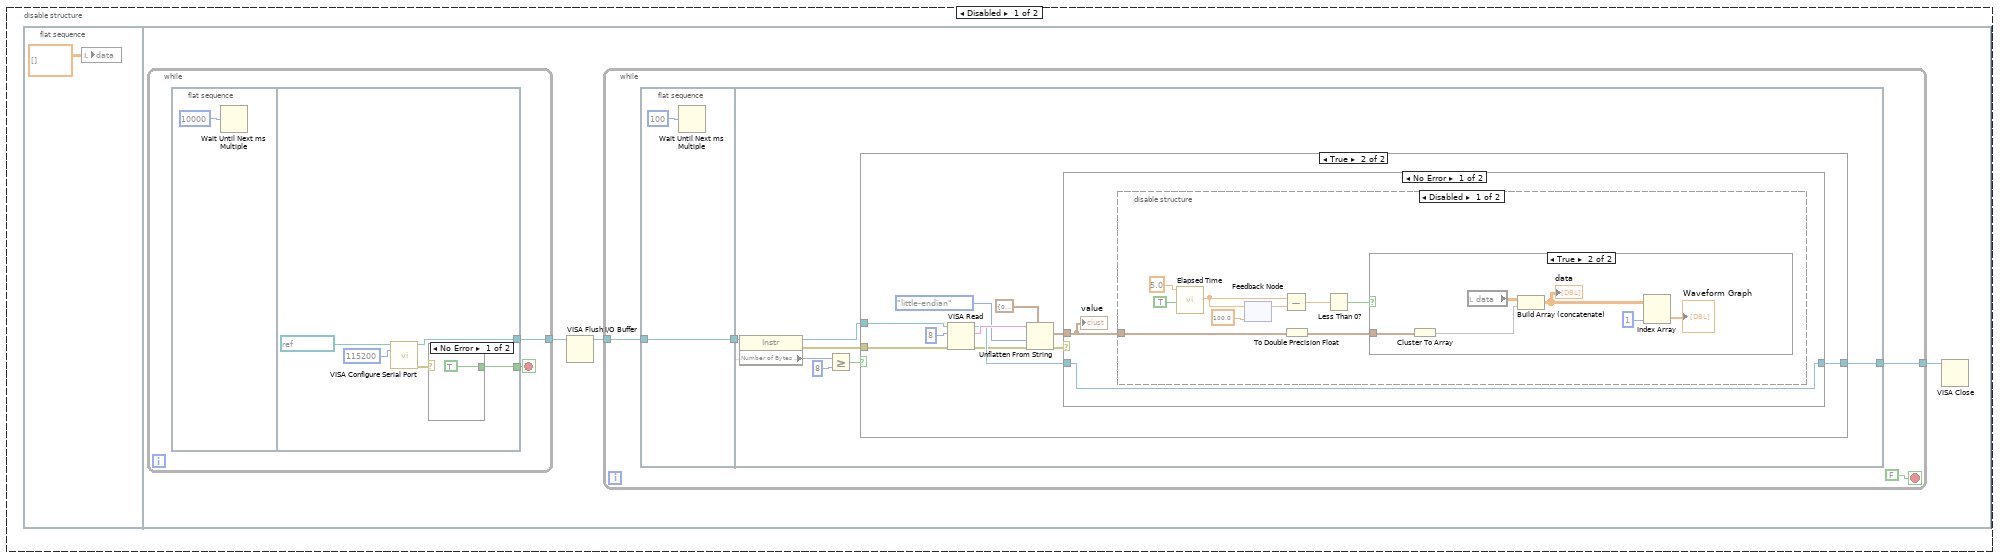
[diagram p2: hidden frame]
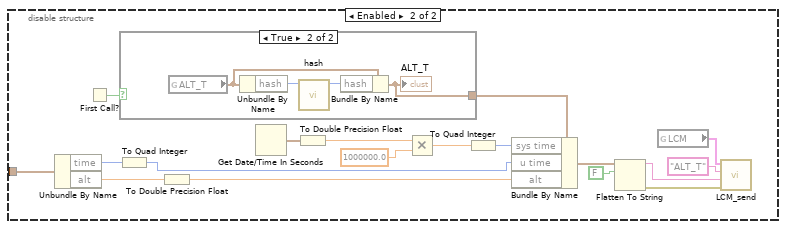
[diagram p6: hidden frame]
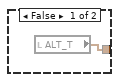
[diagram p7: hidden frame]
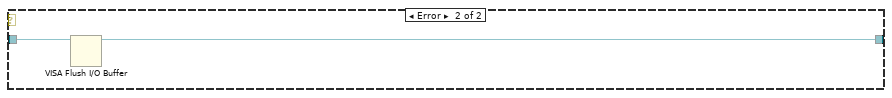
[diagram p8: hidden frame]
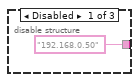
[diagram p9: hidden frame]
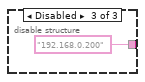
[diagram p10: hidden frame]
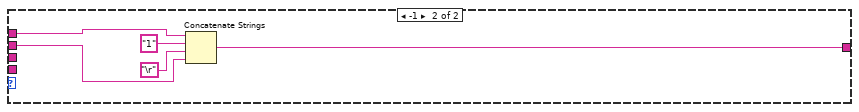
[diagram p12: hidden frame]
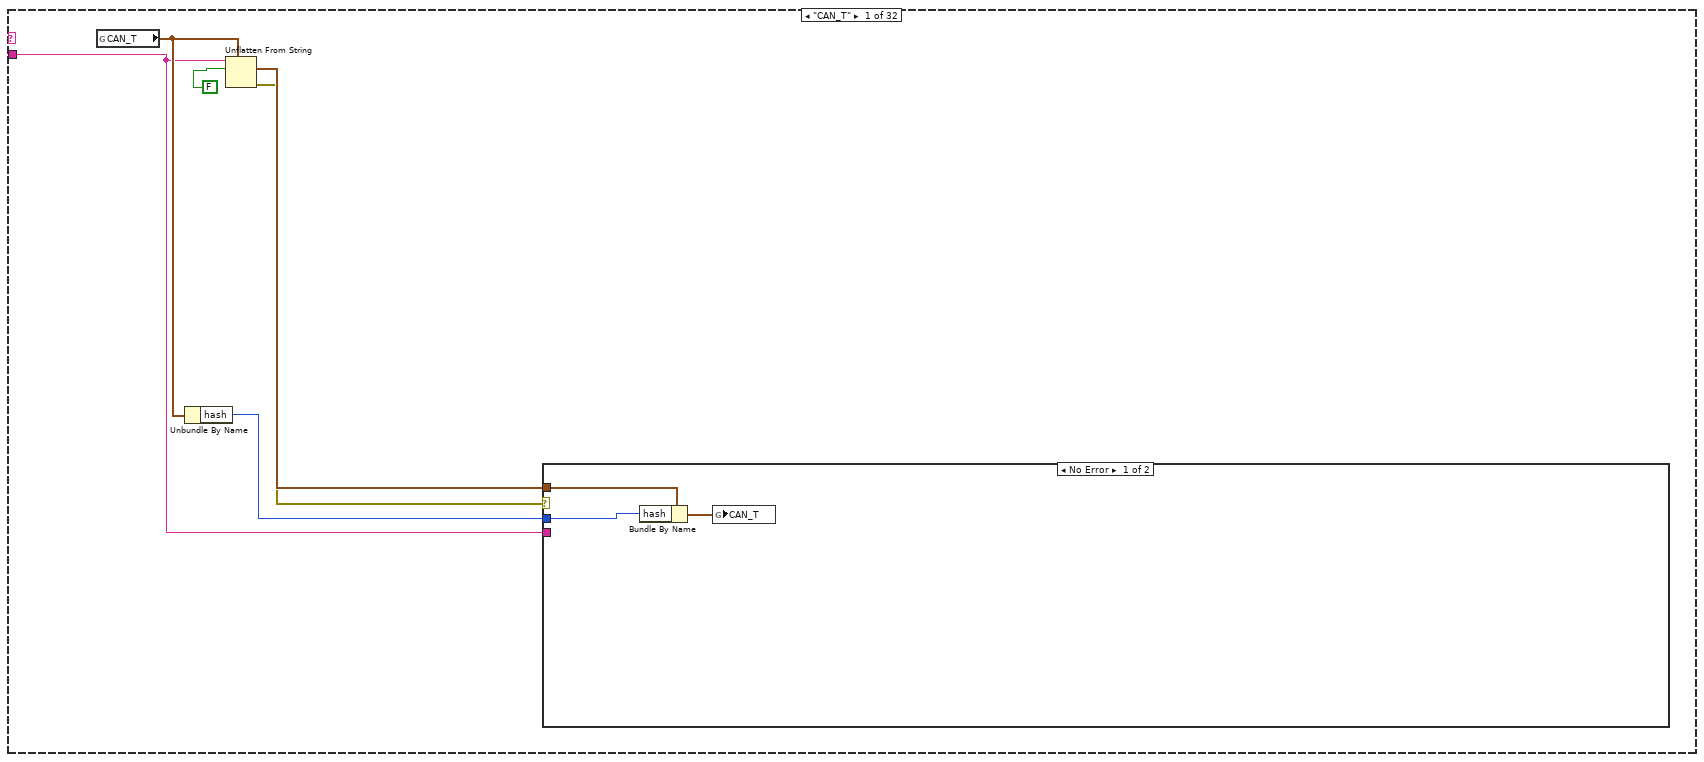
[diagram p13: hidden frame]
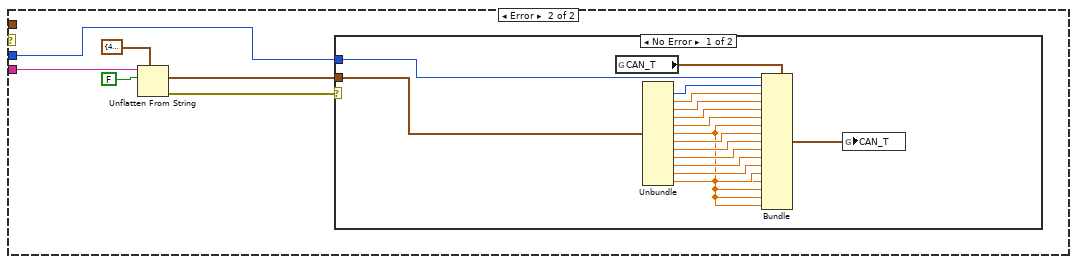
[diagram p14: hidden frame]
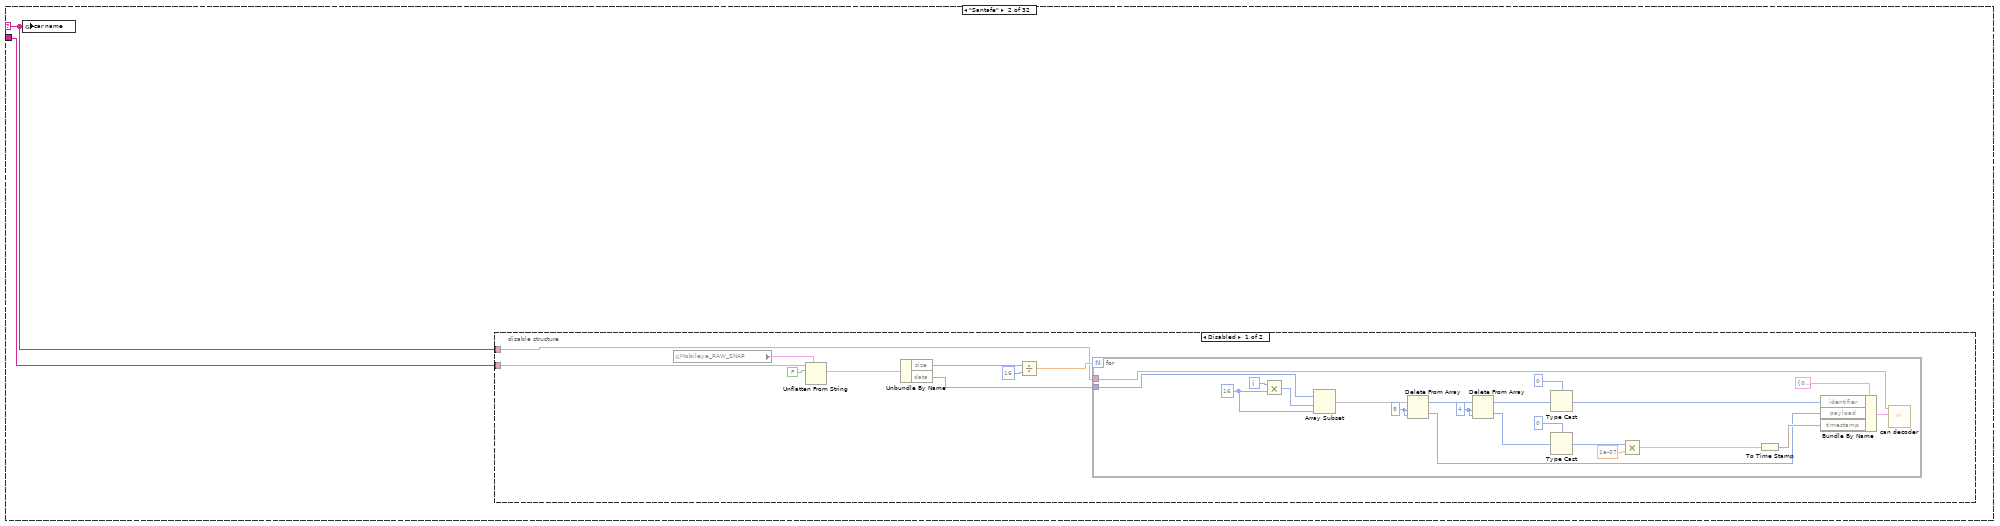
[diagram p16: hidden frame]
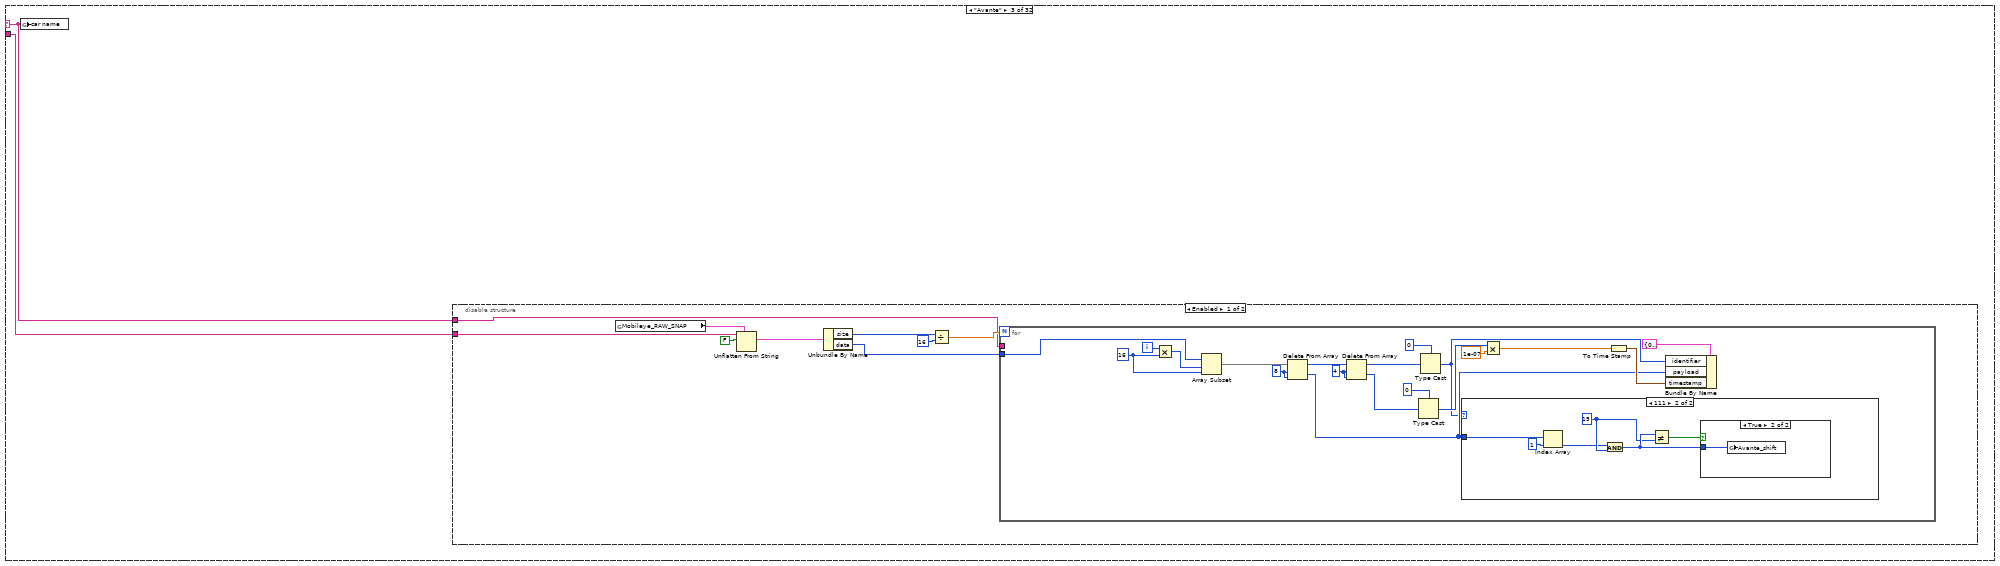
[diagram p18: hidden frame]
diagram:
  n1 = disable-structure shown="Enabled" {
    frame Disabled {
      n2 = flat-sequence {
        frame #0 {
          n3 = local write "data"(dbl[][] [] ("data")) -> ()
        }
        frame #1 {
          n4 = while {
            tunnel: [w6] -> w3
            stop <- w5 stop-if-true
            n5 = flat-sequence {
              tunnel: [w10] -> w6
              tunnel: [w8] -> w5
              frame #0 {
                n6 = Wait Until Next ms Multiple(millisecond multiple=u32 10000) -> ()  [unwired: 1 out]
              }
              frame #1 {
                n7 = call-poly "VISA Configure Serial Port"("VISA resource name"=refnum<visa-resource-name> "COM7", "baud rate (9600)"=u32 115200) -> ("VISA resource name out"=w10:refnum<visa-resource-name>, "error out"=w9:errorcluster)  [unwired: 7 in, 5 out]
                n8 = case shown="No Error" w9 {
                  tunnel: [TRUE _] -> w8
                  frame No Error {
                  }
                  frame Error {
                  }
                }
              }
            }
          }
          n9 = VISA Flush I/O Buffer(VISA resource name=w3) -> (VISA resource name out=w2:refnum<visa-resource-name>)  [unwired: 2 in, 1 out]
          n10 = while {
            tunnel: w2 -> [w15]
            tunnel: [w16] -> w4
            stop <- FALSE ("Boolean") stop-if-true
            n11 = flat-sequence {
              tunnel: w15 -> [w19]
              tunnel: [w19] -> w14
              tunnel: [w26] -> w16
              tunnel: w14 -> [w25]
              frame #0 {
                n12 = Wait Until Next ms Multiple(millisecond multiple=u32 100) -> ()  [unwired: 1 out]
              }
              frame #1 {
                n13 = property class="Instr"(reference=w25) -> (reference out=w24:refnum<visa-resource-name>, error out=w20:errorcluster, "Serial Settings:Number of Bytes at Serial Port"=w23:u32)  [unwired: 1 in]
                n14 = Greater Or Equal?(x=w23, y=u32 8) -> (x >= y?=w21:bool)
                n15 = case shown="True" w21 {
                  tunnel: [w27 w32] -> w26
                  tunnel: w24 -> [w27 w34]
                  tunnel: w20 -> [_ w29]
                  frame False {
                  }
                  frame True {
                    n16 = VISA Read(VISA resource name=w34, byte count=u32 8, error in (no error)=w29) -> (VISA resource name out=w31:refnum<visa-resource-name>, read buffer=w36:string, error out=w30:errorcluster)  [unwired: 1 out]
                    n17 = Unflatten From String(type=cluster{"time":i32, "alt":sgl} {"time"=0, "alt"=0.0}, binary string=w36, byte order (0:big-endian, network order)=T10."little-endian", error in (no error)=w30) -> (value=w28:cluster{"time":i32, "alt":sgl}, error out=w33:errorcluster)  [unwired: 1 in, 1 out]
                    n18 = case shown="No Error" w33 {
                      tunnel: [w40 w79] -> w32
                      tunnel: w31 -> [w40 w80]
                      tunnel: w28 -> [w39 _]
                      frame No Error {
                        n19 = disable-structure shown="Disabled" {
                          disable-tunnel: w39 -> [w49 w73]
                          frame Disabled {
                            n20 = call "Elapsed Time"("Time Target (s)"=5.0, "Auto Reset"=TRUE) -> ("Elapsed Time (s)"=w44:dbl)  [unwired: 10 in, 7 out]
                            n21 = feedback #1(100.0 ("Elapsed Time (s)")) -> (w45:dbl)
                            n22 = feedback-in #1(w44) -> ()
                            n23 = Subtract(x=w44, y=w45) -> (x-y=w43:dbl)
                            n24 = To Double Precision Float(number=w49) -> (double precision float=w48:cluster{"time":dbl, "alt":dbl})
                            n25 = Less Than 0?(x=w43) -> (x < 0?=w42:bool)
                            n26 = case shown="True" w42 {
                              tunnel: w48 -> [_ w55]
                              frame False {
                              }
                              frame True {
                                n27 = Cluster To Array(cluster=w55) -> (array=w54:dbl[])
                                n28 = local read "data"() -> (w53:dbl[][])
                                n29 = Build Array (concatenate)(w53, w54) -> (w52:dbl[][])
                                "data" <- w52
                                n30 = Index Array(array=w52, index (col)=1 ("disabled index (col)")) -> (element=→"Waveform Graph":dbl[])  [unwired: 1 in]
                              }
                            }
                          }
                          frame Enabled {
                            n31 = Unbundle By Name(w73) -> ("time"=w65:i32, "alt"=w63:sgl)
                            n32 = First Call?() -> (First Call?: T/F=w57:bool)
                            n33 = To Quad Integer(1:w65) -> (0:w64:i64)
                            n34 = case shown="True" w57 {
                              tunnel: [w74 w75] -> w56
                              frame False {
                                n35 = local read "ALT_T"() -> (w74:T7)
                              }
                              frame True {
                                n36 = global read "G_LCM.vi" "ALT_T"() -> (w76:T7)
                                n37 = Unbundle By Name(w76) -> ("hash"=w78:i64)
                                n38 = call "hash.vi"("input"=w78) -> ("output"=w77:i64)  [unwired: 10 in]
                                n39 = Bundle By Name(cluster=w76, "hash"=w77) -> (w75:T7)
                                "ALT_T" <- w75
                              }
                            }
                            n40 = To Double Precision Float(number=w63) -> (double precision float=w62:dbl)
                            n41 = Get Date/Time In Seconds() -> (seconds since 1Jan1904=w67:timestamp)
                            n42 = To Double Precision Float(number=w67) -> (double precision float=w68:dbl)
                            n43 = Multiply(x=w68, y=1000000.0) -> (x*y=w70:dbl)
                            n44 = To Quad Integer(1:w70) -> (0:w66:i64)
                            n45 = Bundle By Name(cluster=w56, "sys time"=w66, "u time"=w64, "alt"=w62) -> (w61:T7)
                            n46 = Flatten To String(anything=w61, prepend array or string size? (T)=FALSE) -> (data string=w59:string, error out=w58:errorcluster)  [unwired: 2 in, 1 out]
                            n47 = global read "G_LCM.vi" "LCM"() -> (w72:T11)
                            n48 = call "LCM_send.vi"("error in (no error)"=w58, "DATA"=w59, "ID"="ALT_T", "LCM"=w72) -> ()  [unwired: 6 in, 2 out]
                          }
                        }
                        "value" <- w39
                      }
                      frame Error {
                        n49 = VISA Flush I/O Buffer(VISA resource name=w80) -> (VISA resource name out=w79:refnum<visa-resource-name>)  [unwired: 2 in, 1 out]
                      }
                    }
                  }
                }
              }
            }
          }
          n50 = VISA Close(VISA resource name=w4) -> ()  [unwired: 1 in, 1 out]
        }
      }
    }
    frame Enabled {
    }
  }
  n51 = flat-sequence {
    frame #0 {
      w88 = u16 7667 ("port")
      w97 = u16 7668 ("port 2")
      n52 = disable-structure shown="Enabled" {
        disable-tunnel: ["192.168.0.50" ("name") "192.168.100.200" ("name") "192.168.0.200" ("name")] -> w94
        frame Disabled {
        }
        frame Enabled {
        }
        frame Disabled {
        }
      }
      n53 = String To IP(1:"239.255.76.67" ("Multicast Address")) -> (0:w89:u32)
      n54 = UDP Multicast Open(9:"time-to-live", 10:w89, 11:w88) -> (0:w82:errorcluster, 3:w84:refnum<k16>)  [unwired: 2 in, 1 out]
      n55 = String To IP(1:w94) -> (0:w95:u32)
      n56 = UDP Open(11:w97) -> (port=w96:refnum<k16>)  [unwired: 4 in, 2 out]
      n57 = global read "G_LCM.vi" "LCM 2 RIO"() -> (w99:T11)
      n58 = call "UDP_set_receive_buffer.vi"("error in (no error)"=w82, "Receive Buffer Size"=u32 2097152, "connection ID"=w84) -> ("error out"=w86:errorcluster, "connection ID out"=w85:refnum<k16>)  [unwired: 6 in]
      n59 = Bundle By Name(cluster=w99, "port"=w97, "connection ID"=w96, "net address"=w95) -> (w98:T11)
      n60 = call "UDP_read_receive_buffer.vi"("error in (no error)"=w86, "connection ID"=w85) -> ("error out"=→"LCM error":errorcluster, "connection ID out"=w83:refnum<k16>)  [unwired: 5 in, 1 out]
      n61 = global write "G_LCM.vi" "LCM 2 RIO"(w98) -> ()
      n62 = global read "G_LCM.vi" "LCM"() -> (w91:T11)
      n63 = Bundle By Name(cluster=w91, "port"=w88, "connection ID"=w83, "net address"=w89) -> (w90:T11)
      n64 = global write "G_LCM.vi" "LCM"(w90) -> ()
    }
    frame #1 {
      w114 = "" ("recv data idx")
      n65 = global read "G_LCM.vi" "CON_INPUT_T 2"() -> (w116:T4)
      n66 = global read "G_LCM.vi" "SDT_GPS_DATA"() -> (w120:T5)
      n67 = global read "G_LCM.vi" "IBEO_2202_T"() -> (w111:T8)
      n68 = global read "G_LCM.vi" "VELO_RAW"() -> (w106:T2)
      n69 = global read "G_LCM.vi" "VELO_384"() -> (w104:T14)
      n70 = global write "G_LCM.vi" "recv data"(w114) -> ()
      n71 = global write "G_LCM.vi" "recv data idx"(w114) -> ()
      n72 = Unbundle By Name(w116) -> ("hash"=w117:i64)
      n73 = Unbundle By Name(w111) -> ("hash"=w123:i64)
      n74 = Unbundle By Name(w120) -> ("hash"=w121:i64)
      n75 = Unbundle By Name(w106) -> ("hash"=w109:i64)
      n76 = call "hash.vi"("input"=i64 -3992327254439260095 ("hash")) -> ("output"=w122:i64)  [unwired: 10 in]
      n77 = Obtain Queue(max queue size (-1, unlimited)=2, element data type=w111) -> (queue out=w110:refnum<queue>)  [unwired: 3 in, 2 out]
      n78 = Obtain Queue(max queue size (-1, unlimited)=1000, element data type=w104) -> (queue out=w105:refnum<queue>)  [unwired: 3 in, 2 out]
      n79 = global write "G_LCM.vi" "queue velo"(w105) -> ()
      n80 = global write "G_LCM.vi" "queue ibeo"(w110) -> ()
      n81 = Add(x=w123, y=w122) -> (x+y=w124:i64)
      n82 = call "hash.vi"("input"=w117) -> ("output"=w115:i64)  [unwired: 10 in]
      n83 = call "hash.vi"("input"=w121) -> ("output"=w119:i64)  [unwired: 10 in]
      n84 = call "hash.vi"("input"=w109) -> ("output"=w108:i64)  [unwired: 10 in]
      n85 = Bundle By Name(cluster=w116, "hash"=w115) -> (→"control input":T4)
      n86 = Bundle By Name(cluster=w120, "hash"=w119) -> (→"SDT_GPS_DATA":T5)
      n87 = Bundle By Name(cluster=w106, "hash"=w108) -> (→"VELO_RAW":T2)
      n88 = call "hash.vi"("input"=w124) -> ("output"=w127:i64)  [unwired: 10 in]
      n89 = Bundle By Name(cluster=w111, "hash"=w127) -> (→"IBEO_2202_T":T8)
    }
    frame #2 {
      n90 = while {
        stop <- FALSE stop-if-true
        n91 = global read "G_LCM.vi" "LCM"() -> (w134:T11)
        n92 = call "LCM_read.vi"("LCM"=w134) -> ("data"=w137:string, "ID"=w136:string)  [unwired: 7 in, 2 out]
        n93 = case shown="\"LSTONE_T\"" w136 {
          selector: w136 -> [_ w194 w226 w263 w264 _ _ _ _ _ _ _ _ _ _ _ _ _ _ _ _ _ _ _ _ _ _ w780 _ _ _ _]
          tunnel: w137 -> [w163 w195 w227 _ w266 w277 w398 w408 w421 _ w437 w464 w470 w479 w604 w613 w627 w639 w659 w671 w692 w698 w721 w730 w739 w762 w771 w787 w826 w861 w874 w883]
          frame "CAN_T" {
            n94 = global read "G_LCM.vi" "CAN_T"() -> (w167:T22)
            n95 = Unbundle By Name(w167) -> ("hash"=w165:i64)
            n96 = Unflatten From String(type=w167, binary string=w163, data includes array or string size? (T)=FALSE) -> (value=w166:T22, error out=w164:errorcluster)  [unwired: 2 in, 1 out]
            n97 = case shown="No Error" w164 {
              tunnel: w166 -> [w171 _]
              tunnel: w165 -> [w170 w173]
              tunnel: w163 -> [_ w177]
              frame No Error {
                n98 = Bundle By Name(cluster=w171, "hash"=w170) -> (w169:T22)
                n99 = global write "G_LCM.vi" "CAN_T"(w169) -> ()
              }
              frame Error {
                n100 = Unflatten From String(type=T12 {"hash"=4925705798588944810, "sys time"=0, "time"=0.0, "yaw_rate"=0.0, "mdps torque"=0.0, "mdps str_ang"=0.0, "VS_CAN"=0.0, "lat_accel"=0.0, "mcp"=0.0, "accel pedal value"=0.0, "tps"=0.0, "odometer"=0.0, "battery voltage"=0.0} ("CAN_T"), binary string=w177, data includes array or string size? (T)=FALSE) -> (value=w174:T12, error out=w172:errorcluster)  [unwired: 2 in, 1 out]
                n101 = case shown="No Error" w172 {
                  tunnel: w174 -> [w193 _]
                  tunnel: w173 -> [w179 _]
                  frame No Error {
                    n102 = global read "G_LCM.vi" "CAN_T"() -> (w192:T22)
                    n103 = Unbundle(w193) -> ("sys time"=w191:i64, "time"=w190:dbl, "yaw_rate"=w189:dbl, "mdps torque"=w188:dbl, "mdps str_ang"=w187:dbl, "VS_CAN"=w180:dbl, "lat_accel"=w186:dbl, "mcp"=w185:dbl, "accel pedal value"=w184:dbl, "tps"=w183:dbl, "odometer"=w182:dbl, "battery voltage"=w181:dbl)  [unwired: 1 out]
                    n104 = Bundle(cluster=w192, "hash"=w179, "sys time"=w191, "time"=w190, "yaw_rate"=w189, "mdps torque"=w188, "mdps str_ang"=w187, "VS_CAN"=w180, "lat_accel"=w186, "mcp"=w185, "accel pedal value"=w184, "tps"=w183, "odometer"=w182, "battery voltage"=w181, "WHL_SPD_RR"=w180, "WHL_SPD_RL"=w180, "WHL_SPD_FR"=w180, "WHL_SPD_FL"=w180) -> (w178:T22)
                    n105 = global write "G_LCM.vi" "CAN_T"(w178) -> ()
                  }
                  frame Error {
                  }
                }
              }
            }
          }
          frame "Santafe" {
            n106 = global write "G_LCM.vi" "car name"(w194) -> ()
            n107 = disable-structure shown="Disabled" {
              disable-tunnel: w195 -> [w198 _]
              disable-tunnel: w194 -> [w196 _]
              frame Disabled {
                n108 = global read "G_LCM.vi" "Mobileye_RAW_SNAP"() -> (w199:T23)
                n109 = Unflatten From String(type=w199, binary string=w198, data includes array or string size? (T)=FALSE) -> (value=w197:T23)  [unwired: 2 in, 2 out]
                n110 = Unbundle By Name(w197) -> ("size"=w201:i32, "data"=w204:u8[])
                n111 = Divide(x=w201, y=16) -> (x/y=w203:dbl)
                n112 = for {
                  N: w203 -> [_]
                  tunnel: w204 -> [w225]
                  tunnel: w196 -> [w205]
                  i -> [w224]
                  w217 = 4 ("length")
                  w215 = 8 ("index")
                  w223 = 16 ("y")
                  n113 = Multiply(x=w224, y=w223) -> (x*y=w222:i32)
                  n114 = Array Subset(array=w225, index=w222, length=w223) -> (w207:u8[])
                  n115 = Delete From Array(array=w207, length=w215, index=w215) -> (deleted portion=w208:u8[], array with subset deleted=w216:u8[])
                  n116 = Delete From Array(array=w216, length=w217, index=w217) -> (deleted portion=w221:u8[], array with subset deleted=w218:u8[])
                  n117 = Type Cast(type=u32 0, x=w218) -> (*(type *) &x=w209:u32)
                  n118 = Type Cast(type=u32 0, x=w221) -> (*(type *) &x=w210:u32)
                  n119 = Multiply(x=w210, y=1e-07) -> (x*y=w213:dbl)
                  n120 = To Time Stamp(1:w213) -> (0:w212:timestamp)
                  n121 = Bundle By Name(cluster=T13 {"identifier"=0, "timestamp"=timestamp(0 s since 1904-01-01), "payload"=[]} ("can cluster"), "identifier"=w209, "payload"=w208, "timestamp"=w212) -> (w206:T13)
                  n122 = call "can decoder.vi"("can cluster"=w206, "name"=w205) -> ()  [unwired: 10 in]
                }
              }
              frame Enabled {
              }
            }
          }
          frame "Avante" {
            n123 = global write "G_LCM.vi" "car name"(w226) -> ()
            n124 = disable-structure shown="Enabled" {
              disable-tunnel: w227 -> [w230 _]
              disable-tunnel: w226 -> [w228 _]
              frame Enabled {
                n125 = global read "G_LCM.vi" "Mobileye_RAW_SNAP"() -> (w231:T23)
                n126 = Unflatten From String(type=w231, binary string=w230, data includes array or string size? (T)=FALSE) -> (value=w229:T23)  [unwired: 2 in, 2 out]
                n127 = Unbundle By Name(w229) -> ("size"=w233:i32, "data"=w236:u8[])
                n128 = Divide(x=w233, y=16) -> (x/y=w235:dbl)
                n129 = for {
                  N: w235 -> [_]
                  tunnel: w236 -> [w255]
                  tunnel: w228 -> [_]
                  i -> [w254]
                  w247 = 4 ("length")
                  w245 = 8 ("index")
                  w253 = 16 ("y")
                  n130 = Multiply(x=w254, y=w253) -> (x*y=w252:i32)
                  n131 = Array Subset(array=w255, index=w252, length=w253) -> (w239:u8[])
                  n132 = Delete From Array(array=w239, length=w245, index=w245) -> (deleted portion=w238:u8[], array with subset deleted=w246:u8[])
                  n133 = Delete From Array(array=w246, length=w247, index=w247) -> (deleted portion=w251:u8[], array with subset deleted=w248:u8[])
                  n134 = Type Cast(type=u32 0, x=w251) -> (*(type *) &x=w240:u32)
                  n135 = Type Cast(type=u32 0, x=w248) -> (*(type *) &x=w237:u32)
                  n136 = case shown="111" w237 {
                    tunnel: w238 -> [_ w256]
                    frame 0, Default {
                    }
                    frame 273 {
                      w259 = u8 15 ("y")
                      n137 = Index Array(array=w256, index=1) -> (element=w258:u8)
                      n138 = And(x=w258, y=w259) -> (x .and. y?=w260:u8)
                      n139 = Not Equal?(x=w260, y=w259) -> (x != y?=w261:bool)
                      n140 = case shown="True" w261 {
                        tunnel: w260 -> [_ w262]
                        frame False {
                        }
                        frame True {
                          n141 = global write "G_ALL.vi" "Avante_shift"(w262) -> ()
                        }
                      }
                    }
                  }
                  n142 = Multiply(x=w240, y=1e-07) -> (x*y=w243:dbl)
                  n143 = To Time Stamp(1:w243) -> (0:w242:timestamp)
                  n144 = Bundle By Name(cluster=T13 {"identifier"=0, "timestamp"=timestamp(0 s since 1904-01-01), "payload"=[]} ("can cluster"), "identifier"=w237, "payload"=w238, "timestamp"=w242) -> ()  [unwired: 1 out]
                }
              }
              frame Disabled {
              }
            }
          }
          frame "Prius" {
            # "s"
            n145 = global write "G_LCM.vi" "car name"(w263) -> ()
          }
          frame "Mobileye560", "Mobileye560S" {
            n146 = global read "G_LCM.vi" "car name"() -> (w265:string)
            n147 = case shown="Default" w265 {
              tunnel: w266 -> [_ w268]
              tunnel: w264 -> [_ w267]
              frame "Avante" {
              }
              frame Default {
                n148 = global write "G_LCM.vi" "Mobileye name"(w267) -> ()
                n149 = global read "G_LCM.vi" "Mobileye_RAW_SNAP"() -> (w272:T23)
                n150 = Unbundle By Name(w272) -> ("hash"=w270:i64)
                n151 = Unflatten From String(type=w272, binary string=w268, data includes array or string size? (T)=FALSE) -> (value=w271:T23, error out=w269:errorcluster)  [unwired: 2 in, 1 out]
                n152 = case shown="No Error" w269 {
                  tunnel: w271 -> [w276 _]
                  tunnel: w270 -> [w275 _]
                  frame No Error {
                    n153 = Bundle By Name(cluster=w276, "hash"=w275) -> (w274:T23)
                    n154 = global write "G_LCM.vi" "Mobileye_RAW_SNAP"(w274) -> ()
                  }
                  frame Error {
                  }
                }
              }
            }
          }
          frame "CON_T" {
            n155 = flat-sequence {
              tunnel: w277 -> [w278]
              frame #0 {
                n156 = global read "G_LCM.vi" "CON_T 2"() -> (w281:T24)
                n157 = Unflatten From String(type=w281, binary string=w278, data includes array or string size? (T)=FALSE) -> (value=w280:T24, error out=w279:errorcluster)  [unwired: 2 in, 1 out]
                n158 = case shown="No Error" w279 {
                  tunnel: w280 -> [w298 _]
                  tunnel: w278 -> [_ w314]
                  frame No Error {
                    n159 = Unbundle(w298) -> ("sys time"=w299:i64, "Auto"=w297:bool, "Run"=w296:bool, "Solenoid"=w295:bool, "T lim"=w294:bool, "brk_enc"=w293:u8, "B PWM"=w292:u16, "T PWM"=w291:u16, "ref_vel"=w290:dbl, "ref_bkr_enc"=w289:dbl, "ref_apv"=w288:dbl, "ref_steer"=w287:dbl, "net address"=w283:u32)  [unwired: 1 out]
                    n160 = global read "G_LCM.vi" "CON_T"() -> (w286:T25)
                    n161 = First Call?() -> (First Call?: T/F=w284:bool)
                    n162 = case shown="True" w284 {
                      tunnel: w283 -> [_ w302]
                      frame False {
                      }
                      frame True {
                        n163 = flat-sequence {
                          tunnel: w302 -> [w305]
                          tunnel: [w305] -> w301
                          tunnel: w301 -> [w306]
                          frame #0 {
                            n164 = global read "G_LCM.vi" "LCM 2 RIO"() -> (w304:T11)
                            n165 = Unbundle By Name(w304) -> ("connection ID"=w303:refnum<k16>)
                            n166 = UDP Close(connection ID=w303) -> ()  [unwired: 1 in, 2 out]
                          }
                          frame #1 {
                            w308 = u16 7668 ("port 2")
                            n167 = global read "G_LCM.vi" "LCM 2 RIO"() -> (w310:T11)
                            n168 = UDP Open(11:w308) -> (port=w307:refnum<k16>)  [unwired: 4 in, 2 out]
                            n169 = Bundle By Name(cluster=w310, "port"=w308, "connection ID"=w307, "net address"=w306) -> (w309:T11)
                            n170 = global write "G_LCM.vi" "LCM 2 RIO"(w309) -> ()
                          }
                        }
                      }
                    }
                    n171 = Unbundle By Name(w286) -> ("hash"=w285:i64)
                    n172 = Bundle(cluster=w286, "hash"=w285, "sys time"=w299, "Auto"=w297, "Run"=w296, "Solenoid"=w295, "T lim"=w294, "brk_enc"=w293, "B PWM"=w292, "T PWM"=w291, "ref_vel"=w290, "ref_bkr_enc"=w289, "ref_apv"=w288, "ref_steer"=w287) -> (w300:T25)
                    n173 = global write "G_LCM.vi" "CON_T"(w300) -> ()
                  }
                  frame Error {
                    n174 = global read "G_LCM.vi" "CON_T"() -> (w316:T25)
                    n175 = Unbundle By Name(w316) -> ("hash"=w311:i64)
                    n176 = Unflatten From String(type=w316, binary string=w314, data includes array or string size? (T)=FALSE) -> (value=w312:T25, error out=w313:errorcluster)  [unwired: 2 in, 1 out]
                    n177 = case shown="No Error" w313 {
                      tunnel: w312 -> [w319 _]
                      tunnel: w311 -> [w317 _]
                      frame No Error {
                        n178 = Bundle By Name(cluster=w319, "hash"=w317) -> (w318:T25)
                        n179 = global write "G_LCM.vi" "CON_T"(w318) -> ()
                      }
                      frame Error {
                      }
                    }
                  }
                }
              }
              frame #1 {
                n180 = disable-structure shown="Enabled" {
                  frame Enabled {
                    n181 = Get Date/Time In Seconds() -> (seconds since 1Jan1904=w340:timestamp)
                    n182 = global read "G_LCM.vi" "ibeo"() -> (w326:bool)
                    n183 = To Double Precision Float(number=w340) -> (double precision float=w339:dbl)
                    n184 = global read "G_ALL.vi" "Steering"() -> (w321:dbl)
                    n185 = Build Array(w326) -> (w325:bool[])
                    n186 = Multiply(x=w339, y=1000000.0) -> (x*y=w337:dbl)
                    n187 = Negate(x=w321) -> (-x=w320:dbl)
                    n188 = Boolean Array To Number(Boolean array=w325) -> (number=w324:u32)
                    n189 = local read "control input"() -> (w329:T4)
                    n190 = global read "G_ALL.vi" "VS_des"() -> (w322:dbl)
                    n191 = To Quad Integer(1:w337) -> (0:w336:i64)
                    n192 = To Unsigned Byte Integer(number=w324) -> (unsigned 8bit integer=w323:u8)
                    n193 = Add(x=w320, y=0.0) -> (x+y=w327:dbl)
                    n194 = Bundle By Name(cluster=w329, "sys time"=w336, "ref_vel"=w322, "ref_steer"=w327, "alert"=w323) -> (w331:T4)
                    n195 = global read "G_LCM.vi" "LCM 2 RIO"() -> (w330:T11)
                    n196 = Flatten To String(anything=w331, prepend array or string size? (T)=FALSE) -> (data string=w332:string, error out=w335:errorcluster)  [unwired: 2 in, 1 out]
                    n197 = call "LCM_send.vi"("error in (no error)"=w335, "DATA"=w332, "ID"="CON_INPUT_T", "LCM"=w330) -> ()  [unwired: 6 in, 2 out]
                  }
                  frame Disabled {
                  }
                }
              }
              frame #2 {
                n198 = global read "G_ALL.vi" "replay"() -> (w341:bool)
                n199 = case shown="False" w341 {
                  frame False {
                    n200 = disable-structure shown="Enabled" {
                      frame Enabled {
                        n201 = First Call?() -> (First Call?: T/F=w351:bool)
                        n202 = case shown="True" w351 {
                          tunnel: [w363 w364] -> w350
                          frame False {
                            n203 = local read "PATH_T"() -> (w363:T6)
                          }
                          frame True {
                            n204 = global read "G_LCM.vi" "PATH_T"() -> (w365:T6)
                            n205 = Unbundle By Name(w365) -> ("hash"=w367:i64)
                            n206 = call "hash.vi"("input"=w367) -> ("output"=w366:i64)  [unwired: 10 in]
                            n207 = Bundle By Name(cluster=w365, "hash"=w366) -> (w364:T6)
                            "PATH_T" <- w364
                          }
                        }
                        n208 = global read "G_ALL.vi" "map_track 2"() -> (w342:dbl[][])
                        n209 = Get Date/Time In Seconds() -> (seconds since 1Jan1904=w357:timestamp)
                        n210 = To Double Precision Float(number=w357) -> (double precision float=w358:dbl)
                        n211 = Transpose 2D Array(2D array=w342) -> (transposed array=w346:dbl[][])
                        n212 = Array Size(array=w342) -> (size(s)=w345:i32[])
                        n213 = Multiply(x=w358, y=1000000.0) -> (x*y=w360:dbl)
                        n214 = Multiply Array Elements(1:w345) -> (0:w344:i32)
                        n215 = Index Array(array=w345, index=0) -> (element=w348:i32)
                        n216 = Reshape Array(w346, w344) -> (w343:dbl[])
                        n217 = To Quad Integer(1:w360) -> (0:w356:i64)
                        n218 = To Unsigned Long Integer(number=w348) -> (unsigned 32bit integer=w347:u32)
                        n219 = Bundle By Name(cluster=w350, "sys time"=w356, "n"=w347, "pathxy"=w343) -> (w355:T6)
                        n220 = Flatten To String(anything=w355, prepend array or string size? (T)=FALSE) -> (data string=w353:string, error out=w352:errorcluster)  [unwired: 2 in, 1 out]
                        n221 = global read "G_LCM.vi" "LCM"() -> (w362:T11)
                        n222 = call "LCM_send.vi"("error in (no error)"=w352, "DATA"=w353, "ID"="PATH_T", "LCM"=w362) -> ()  [unwired: 6 in, 2 out]
                      }
                      frame Disabled {
                      }
                    }
                  }
                  frame True {
                  }
                }
              }
              frame #3 {
                n223 = First Call?() -> (First Call?: T/F=w371:bool)
                n224 = case shown="True" w371 {
                  tunnel: [w392 w393] -> w370
                  frame False {
                    n225 = local read "mission_request"() -> (w392:T1)
                  }
                  frame True {
                    n226 = global read "G_LCM.vi" "mission_request"() -> (w394:T1)
                    n227 = Unbundle By Name(w394) -> ("hash"=w396:i64)
                    n228 = call "hash.vi"("input"=w396) -> ("output"=w395:i64)  [unwired: 10 in]
                    n229 = Bundle By Name(cluster=w394, "hash"=w395) -> (w393:T1)
                    "mission_request" <- w393
                  }
                }
                n230 = global read "G_ALL.vi" "mission num"() -> (w369:i32)
                n231 = case shown="8" w369 {
                  tunnel: [i32[] [0, 0, 0, 0, 1, 0, 0, 0, 0, 0, 0, 0, 0, 0, 0, 0, 0, 0] i32[] [0, 0, 0, 1, 1, 1, 0, 0, 0, 0, 0, 0, 0, 0, 0, 0, 0, 0] i32[] [0, 0, 1, 0, 1, 0, 0, 0, 0, 0, 0, 0, 0, 0, 0, 0, 0, 0] i32[] [0, 0, 1, 1, 1, 1, 1, 0, 0, 0, 0, 0, 0, 0, 0, 0, 0, 0] i32[] [0, 1, 0, 0, 1, 0, 0, 0, 0, 0, 0, 0, 0, 0, 0, 0, 0, 0] i32[] [0, 1, 0, 1, 1, 1, 0, 1, 1, 0, 0, 0, 0, 0, 0, 0, 0, 0] i32[] [0, 1, 1, 0, 1, 0, 0, 0, 0, 0, 0, 0, 0, 1, 0, 0, 0, 0] i32[] [0, 1, 1, 1, 1, 0, 0, 0, 0, 1, 1, 0, 0, 0, 0, 0, 0, 0] i32[] [1, 0, 0, 0, 0, 0, 0, 0, 0, 0, 0, 1, 1, 0, 0, 0, 0, 0]] -> w368
                  frame 0, Default {
                  }
                  frame 1 {
                  }
                  frame 2 {
                  }
                  frame 3 {
                  }
                  frame 4 {
                  }
                  frame 5 {
                  }
                  frame 6 {
                  }
                  frame 7 {
                  }
                  frame 8 {
                  }
                }
                n232 = Get Date/Time In Seconds() -> (seconds since 1Jan1904=w377:timestamp)
                n233 = To Double Precision Float(number=w377) -> (double precision float=w378:dbl)
                n234 = Multiply(x=w378, y=1000000.0) -> (x*y=w380:dbl)
                n235 = To Quad Integer(1:w380) -> (0:w376:i64)
                n236 = Bundle By Name(cluster=w370, "sys time"=w376, "request"=w368) -> (w375:T1)
                n237 = Flatten To String(anything=w375, prepend array or string size? (T)=FALSE) -> (data string=w373:string, error out=w372:errorcluster)  [unwired: 2 in, 1 out]
                n238 = global read "G_LCM.vi" "LCM"() -> (w382:T11)
                n239 = call "LCM_send.vi"("error in (no error)"=w372, "DATA"=w373, "ID"="mission_request", "LCM"=w382) -> ()  [unwired: 6 in, 2 out]
              }
            }
          }
          frame "EYE_RAW_T", "EYE_T" {
            n240 = global read "G_LCM.vi" "EYE_RAW_T"() -> (w402:T26)
            n241 = global write "G_LCM.vi" "Mobileye name"("Mobileye" ("Mobileye name")) -> ()
            n242 = Unbundle By Name(w402) -> ("hash"=w400:i64)
            n243 = Unflatten From String(type=w402, binary string=w398, data includes array or string size? (T)=FALSE) -> (value=w401:T26, error out=w399:errorcluster)  [unwired: 2 in, 1 out]
            n244 = case shown="No Error" w399 {
              tunnel: w401 -> [w405 _]
              tunnel: w400 -> [w404 _]
              frame No Error {
                n245 = Bundle By Name(cluster=w405, "hash"=w404) -> (w406:T26)
                n246 = global write "G_LCM.vi" "EYE_RAW_T"(w406) -> ()
              }
              frame Error {
              }
            }
          }
          frame "CAN_EYE_RAW_T" {
            n247 = global write "G_LCM.vi" "Mobileye name"("Mobileye" ("Mobileye name")) -> ()
            n248 = global read "G_LCM.vi" "CAN_EYE_RAW_T"() -> (w412:T27)
            n249 = Unbundle By Name(w412) -> ("hash"=w410:i64)
            n250 = Unflatten From String(type=w412, binary string=w408, data includes array or string size? (T)=FALSE) -> (value=w411:T27, error out=w409:errorcluster)  [unwired: 2 in, 1 out]
            n251 = case shown="Error" w409 {
              tunnel: w411 -> [w415 _]
              tunnel: w410 -> [w414 _]
              frame No Error {
                n252 = Bundle By Name(cluster=w415, "hash"=w414) -> (w416:T27)
                n253 = global write "G_LCM.vi" "CAN_EYE_RAW_T"(w416) -> ()
              }
              frame Error {
              }
            }
          }
          frame "CAN_CAR_RAW_T" {
            n254 = global read "G_LCM.vi" "CAN_CAR_RAW_T"() -> (w420:T28)
            n255 = Unbundle By Name(w420) -> ("hash"=w418:i64)
            n256 = Unflatten From String(type=w420, binary string=w421, data includes array or string size? (T)=FALSE) -> (value=w419:T28, error out=w417:errorcluster)  [unwired: 2 in, 1 out]
            n257 = case shown="No Error" w417 {
              tunnel: w419 -> [w424 _]
              tunnel: w418 -> [w423 _]
              frame No Error {
                n258 = Bundle By Name(cluster=w424, "hash"=w423) -> (w425:T28)
                n259 = global write "G_LCM.vi" "CAN_CAR_RAW_T"(w425) -> ()
              }
              frame Error {
              }
            }
          }
          frame "False", Default {
          }
          frame "IBEO_2202_T" {
            n260 = global read "G_LCM.vi" "IBEO_2202_T"() -> (w426:T8)
            n261 = Unbundle By Name(w426) -> ("hash"=w435:i64)
            n262 = Unbundle(w426) -> ("hash"=w432:i64, "sys time"=w433:i64, "Header"=w431:T9, "Scan header"=w430:T29, "Scan points"=w427:T30)
            n263 = Bundle("hash"=w432, "sys time"=w433, "Header"=w431, "Scan header"=w430) -> (w429:T31)  [unwired: 1 in]
            n264 = Unflatten From String(type=w429, binary string=w437, data includes array or string size? (T)=FALSE) -> (rest of the binary string=w428:string, value=w436:T31, error out=w434:errorcluster)  [unwired: 2 in]
            n265 = case shown="No Error" w434 {
              tunnel: w436 -> [w447 _]
              tunnel: w435 -> [w446 _]
              tunnel: w428 -> [w452 _]
              tunnel: w427 -> [w451 _]
              tunnel: w426 -> [w448 _]
              frame No Error {
                n266 = Unbundle By Name(w447) -> ("Header.Size of this messages"=w453:u32)
                n267 = Index Array(array=w451, index=0) -> (element=w449:T32)
                n268 = for {
                  N: w453 -> [_]
                  shift-right: [w456] -> _
                  shift-left: w452 -> [w458]
                  tunnel: w449 -> [w457]
                  tunnel: [w455] -> w442 mode=indexing
                  tunnel: [w454] -> _
                  n269 = Unflatten From String(type=w457, binary string=w458, data includes array or string size? (T)=FALSE) -> (rest of the binary string=w456:string, value=w455:T32, error out=w454:errorcluster)  [unwired: 2 in]
                }
                n270 = Unbundle(w447) -> ("sys time"=w445:i64, "Header"=w444:T9, "Scan header"=w443:T29)  [unwired: 1 out]
                n271 = global read "G_LCM.vi" "queue ibeo"() -> (w441:refnum<queue>)
                n272 = Bundle(cluster=w448, "hash"=w446, "sys time"=w445, "Header"=w444, "Scan header"=w443, "Scan points"=w442) -> (w439:T8)
                n273 = global write "G_LCM.vi" "IBEO_2202_T"(w439) -> ()
                n274 = Lossy Enqueue Element(queue=w441, element=w439) -> (overflow?=→"ibeo overflow?":bool)  [unwired: 1 in, 3 out]
              }
              frame Error {
              }
            }
          }
          frame "VELO_PT_T" {
            n275 = global read "G_LCM.vi" "VELO_PT_T"() -> (w461:T33)
            n276 = Unflatten From String(type=w461, binary string=w464, data includes array or string size? (T)=FALSE) -> (value=w462:T33, error out=w460:errorcluster)  [unwired: 2 in, 1 out]
            n277 = case shown="No Error" w460 {
              tunnel: w462 -> [w465 _]
              frame No Error {
                n278 = call "velosterstack.vi"("VELO_PT_T"=w465) -> ()  [unwired: 10 in, 1 out]
              }
              frame Error {
              }
            }
          }
          frame "VELO_384 " {
            n279 = global read "G_LCM.vi" "VELO_384"() -> (w467:T14)
            n280 = Unflatten From String(type=w467, binary string=w470, data includes array or string size? (T)=FALSE) -> (value=w468:T14, error out=w466:errorcluster)  [unwired: 2 in, 1 out]
            n281 = case shown="No Error" w466 {
              tunnel: w468 -> [w471 _]
              frame No Error {
                n282 = flat-sequence {
                  tunnel: w471 -> [w473]
                  frame #0 {
                    n283 = global read "G_LCM.vi" "queue velo"() -> (w472)
                    n284 = Lossy Enqueue Element(queue=w472, element=w473) -> (overflow?=→"velodyne overflow? 2":bool)  [unwired: 1 in, 3 out]
                  }
                }
              }
              frame Error {
              }
            }
          }
          frame "VELO_RAW" {
            n285 = global read "G_LCM.vi" "VELO_RAW"() -> (w477:T2)
            n286 = Unflatten From String(type=w477, binary string=w479, data includes array or string size? (T)=FALSE) -> (value=w475:T2, error out=w476:errorcluster)  [unwired: 2 in, 1 out]
            n287 = case shown="No Error" w476 {
              tunnel: w475 -> [w504 _]
              frame No Error {
                n288 = Unbundle By Name(w504) -> ("raw"=w503:string, "type"=w502:u8)
                n289 = case shown="2" w502 {
                  tunnel: [w535 w536 w537] -> w486
                  frame 0 {
                    w535 = dbl[][] [[0.0, -15.0, 0.0, 0.0, 0.0], [0.0, 1.0, 0.0, 0.0, 0.0], [0.0, -13.0, 0.0, 0.0, 0.0], [0.0, 3.0, 0.0, 0.0, 0.0], [0.0, -11.0, 0.0, 0.0, 0.0], [0.0, 5.0, 0.0, 0.0, 0.0], [0.0, -9.0, 0.0, 0.0, 0.0], [0.0, 7.0, 0.0, 0.0, 0.0], [0.0, -7.0, 0.0, 0.0, 0.0], [0.0, 9.0, 0.0, 0.0, 0.0], [0.0, -5.0, 0.0, 0.0, 0.0], [0.0, 11.0, 0.0, 0.0, 0.0], [0.0, -3.0, 0.0, 0.0, 0.0], [0.0, 13.0, 0.0, 0.0, 0.0], [0.0, -1.0, 0.0, 0.0, 0.0], [0.0, 15.0, 0.0, 0.0, 0.0], [0.0, -15.0, 0.0, 0.0, 0.0], [0.0, 1.0, 0.0, 0.0, 0.0], [0.0, -13.0, 0.0, 0.0, 0.0], [0.0, 3.0, 0.0, 0.0, 0.0], [0.0, -11.0, 0.0, 0.0, 0.0], [0.0, 5.0, 0.0, 0.0, 0.0], [0.0, -9.0, 0.0, 0.0, 0.0], [0.0, 7.0, 0.0, 0.0, 0.0], [0.0, -7.0, 0.0, 0.0, 0.0], [0.0, 9.0, 0.0, 0.0, 0.0], [0.0, -5.0, 0.0, 0.0, 0.0], [0.0, 11.0, 0.0, 0.0, 0.0], [0.0, -3.0, 0.0, 0.0, 0.0], [0.0, 13.0, 0.0, 0.0, 0.0], [0.0, -1.0, 0.0, 0.0, 0.0], [0.0, 15.0, 0.0, 0.0, 0.0], [0.0, 0.0, 0.0, 0.0, 0.0], [0.0, 0.0, 0.0, 0.0, 0.0], [0.0, 0.0, 0.0, 0.0, 0.0], [0.0, 0.0, 0.0, 0.0, 0.0], [0.0, 0.0, 0.0, 0.0, 0.0], [0.0, 0.0, 0.0, 0.0, 0.0], [0.0, 0.0, 0.0, 0.0, 0.0], [0.0, 0.0, 0.0, 0.0, 0.0], [0.0, 0.0, 0.0, 0.0, 0.0], [0.0, 0.0, 0.0, 0.0, 0.0], [0.0, 0.0, 0.0, 0.0, 0.0], [0.0, 0.0, 0.0, 0.0, 0.0], [0.0, 0.0, 0.0, 0.0, 0.0], [0.0, 0.0, 0.0, 0.0, 0.0], [0.0, 0.0, 0.0, 0.0, 0.0], [0.0, 0.0, 0.0, 0.0, 0.0], [0.0, 0.0, 0.0, 0.0, 0.0], [0.0, 0.0, 0.0, 0.0, 0.0], [0.0, 0.0, 0.0, 0.0, 0.0], [0.0, 0.0, 0.0, 0.0, 0.0], [0.0, 0.0, 0.0, 0.0, 0.0], [0.0, 0.0, 0.0, 0.0, 0.0], [0.0, 0.0, 0.0, 0.0, 0.0], [0.0, 0.0, 0.0, 0.0, 0.0], [0.0, 0.0, 0.0, 0.0, 0.0], [0.0, 0.0, 0.0, 0.0, 0.0], [0.0, 0.0, 0.0, 0.0, 0.0], [0.0, 0.0, 0.0, 0.0, 0.0], [0.0, 0.0, 0.0, 0.0, 0.0], [0.0, 0.0, 0.0, 0.0, 0.0], [0.0, 0.0, 0.0, 0.0, 0.0], [0.0, 0.0, 0.0, 0.0, 0.0]]  # Velo 16
                  }
                  frame 1, Default {
                    w536 = dbl[][] [[0.0, -30.67, 0.0, 0.0, 0.0], [0.0, -9.3299999, 0.0, 0.0, 0.0], [0.0, -29.33, 0.0, 0.0, 0.0], [0.0, -8.0, 0.0, 0.0, 0.0], [0.0, -28.0, 0.0, 0.0, 0.0], [0.0, -6.6700001, 0.0, 0.0, 0.0], [0.0, -26.67, 0.0, 0.0, 0.0], [0.0, -5.3299999, 0.0, 0.0, 0.0], [0.0, -25.33, 0.0, 0.0, 0.0], [0.0, -4.0, 0.0, 0.0, 0.0], [0.0, -24.0, 0.0, 0.0, 0.0], [0.0, -2.6700001, 0.0, 0.0, 0.0], [0.0, -22.67, 0.0, 0.0, 0.0], [0.0, -1.33, 0.0, 0.0, 0.0], [0.0, -21.33, 0.0, 0.0, 0.0], [0.0, 0.0, 0.0, 0.0, 0.0], [0.0, -20.0, 0.0, 0.0, 0.0], [0.0, 1.33, 0.0, 0.0, 0.0], [0.0, -18.67, 0.0, 0.0, 0.0], [0.0, 2.6700001, 0.0, 0.0, 0.0], [0.0, -17.33, 0.0, 0.0, 0.0], [0.0, 4.0, 0.0, 0.0, 0.0], [0.0, -16.0, 0.0, 0.0, 0.0], [0.0, 5.3299999, 0.0, 0.0, 0.0], [0.0, -14.67, 0.0, 0.0, 0.0], [0.0, 6.6700001, 0.0, 0.0, 0.0], [0.0, -13.33, 0.0, 0.0, 0.0], [0.0, 8.0, 0.0, 0.0, 0.0], [0.0, -12.0, 0.0, 0.0, 0.0], [0.0, 9.3299999, 0.0, 0.0, 0.0], [0.0, -10.67, 0.0, 0.0, 0.0], [0.0, 10.67, 0.0, 0.0, 0.0], [0.0, 0.0, 0.0, 0.0, 0.0], [0.0, 0.0, 0.0, 0.0, 0.0], [0.0, 0.0, 0.0, 0.0, 0.0], [0.0, 0.0, 0.0, 0.0, 0.0], [0.0, 0.0, 0.0, 0.0, 0.0], [0.0, 0.0, 0.0, 0.0, 0.0], [0.0, 0.0, 0.0, 0.0, 0.0], [0.0, 0.0, 0.0, 0.0, 0.0], [0.0, 0.0, 0.0, 0.0, 0.0], [0.0, 0.0, 0.0, 0.0, 0.0], [0.0, 0.0, 0.0, 0.0, 0.0], [0.0, 0.0, 0.0, 0.0, 0.0], [0.0, 0.0, 0.0, 0.0, 0.0], [0.0, 0.0, 0.0, 0.0, 0.0], [0.0, 0.0, 0.0, 0.0, 0.0], [0.0, 0.0, 0.0, 0.0, 0.0], [0.0, 0.0, 0.0, 0.0, 0.0], [0.0, 0.0, 0.0, 0.0, 0.0], [0.0, 0.0, 0.0, 0.0, 0.0], [0.0, 0.0, 0.0, 0.0, 0.0], [0.0, 0.0, 0.0, 0.0, 0.0], [0.0, 0.0, 0.0, 0.0, 0.0], [0.0, 0.0, 0.0, 0.0, 0.0], [0.0, 0.0, 0.0, 0.0, 0.0], [0.0, 0.0, 0.0, 0.0, 0.0], [0.0, 0.0, 0.0, 0.0, 0.0], [0.0, 0.0, 0.0, 0.0, 0.0], [0.0, 0.0, 0.0, 0.0, 0.0], [0.0, 0.0, 0.0, 0.0, 0.0], [0.0, 0.0, 0.0, 0.0, 0.0], [0.0, 0.0, 0.0, 0.0, 0.0], [0.0, 0.0, 0.0, 0.0, 0.0]]  # Velo_32
                  }
                  frame 2 {
                    w537 = dbl[][] [[-5.3328056, -7.2988362, 111.0, 19.736338, 2.5999999], [-3.2344019, -6.9644198, 146.0, 19.778963, -2.5999999], [2.4376695, 0.250889, 131.76823, 20.688799, 2.5999999], [4.7373252, 0.55538797, 138.12656, 20.727015, -2.5999999], [-1.0502493, -6.6410818, 119.0, 19.82012, 2.5999999], [1.2386309, -6.2594609, 135.0, 19.868624, -2.5999999], [-1.8405367, -8.6656351, 132.0, 19.561426, 2.5999999], [0.4511103, -8.3104696, 145.0, 19.606993, -2.5999999], [3.2611551, -5.9352221, 116.0, 19.909781, 2.5999999], [5.4685535, -5.587399, 133.99889, 19.953875, -2.5999999], [2.4743285, -7.9891219, 117.0, 19.648148, 2.5999999], [4.7189918, -7.644258, 145.0, 19.692244, -2.5999999], [-5.3511744, -3.2475569, 118.71672, 20.249313, 2.5999999], [-3.1158857, -2.850472, 142.90839, 20.29929, -2.5999999], [-6.1270261, -5.204318, 120.0, 20.00238, 2.5999999], [-3.852011, -4.9137921, 137.0, 20.039125, -2.5999999], [-1.1109436, -2.4998751, 101.71324, 20.343384, 2.5999999], [1.1519098, -2.184176, 145.31258, 20.38307, -2.5999999], [-1.8682934, -4.5764661, 130.0, 20.081753, 2.5999999], [0.43604341, -4.2038751, 147.0, 20.128786, -2.5999999], [3.1763444, -1.798143, 115.82812, 20.431576, 2.5999999], [5.4284201, -1.49388, 146.0, 20.469791, -2.5999999], [2.4024715, -1.877563, 129.29713, 20.169943, 2.5999999], [4.6698937, -3.492661, 157.97737, 20.218447, -2.5999999], [-5.3977456, 0.88327599, 124.12312, 20.768169, 2.5999999], [-3.1504908, 1.234519, 128.0, 20.812265, -2.5999999], [-6.1759849, -1.177825, 133.0, 20.509478, 2.5999999], [-3.8819003, -0.86169797, 130.0, 20.549164, -2.5999999], [-1.1136208, 1.585669, 131.0, 20.856361, 2.5999999], [1.0969903, 1.925001, 131.0, 20.898987, -2.5999999], [-1.9088749, -0.486963, 138.48773, 20.596197, 2.5999999], [0.36758029, -0.123898, 137.21994, 20.641764, -2.5999999], [-8.3386211, -22.597513, 117.0, 10.828748, 2.5999999], [-4.7629819, -22.397568, 100.0, 10.854152, -2.5999999], [4.1516571, -11.576517, 130.0, 12.142142, 2.5999999], [7.3577185, -10.877901, 102.0, 12.220895, -2.5999999], [-1.2630961, -21.935509, 106.0, 10.912581, 2.5999999], [2.1595552, -21.409546, 91.0, 10.978632, -2.5999999], [-2.6141083, -25.066507, 127.0, 10.508655, 2.5999999], [0.95595688, -24.458101, 95.0, 10.588678, -2.5999999], [5.5369682, -20.777454, 106.0, 11.057385, 2.5999999], [8.9712191, -20.243195, 97.0, 11.123436, -2.5999999], [4.4757471, -23.863358, 115.0, 10.666161, 2.5999999], [7.8848143, -23.352007, 92.0, 10.732212, -2.5999999], [-8.0466499, -16.629311, 135.0, 11.559117, 2.5999999], [-4.595552, -16.230633, 108.0, 11.606115, -2.5999999], [-9.3918352, -19.788239, 135.0, 11.179325, 2.5999999], [-5.9566336, -19.21587, 98.0, 11.249186, -2.5999999], [-1.3779737, -15.754419, 116.0, 11.662004, 2.5999999], [2.0754263, -15.166914, 105.0, 11.730595, -2.5999999], [-2.5654242, -18.828558, 138.0, 11.296184, 2.5999999], [0.87227631, -18.312876, 105.0, 11.358424, -2.5999999], [5.2989287, -14.641928, 123.0, 11.791565, 2.5999999], [8.7970304, -14.048302, 86.0, 11.860156, -2.5999999], [4.1742177, -17.687857, 135.0, 11.433367, 2.5999999], [7.5869775, -17.16544, 92.0, 11.495607, -2.5999999], [-7.8831077, -10.436752, 121.0, 12.270433, 2.5999999], [-4.5919614, -10.085198, 103.0, 12.30981, -2.5999999], [-9.1805763, -13.484814, 146.0, 11.924937, 2.5999999], [-5.7835727, -13.107666, 99.0, 11.968124, -2.5999999], [-1.2335371, -9.5621262, 123.0, 12.368239, 2.5999999], [1.9424959, -9.0374413, 106.0, 12.426669, -2.5999999], [-2.5727935, -12.651329, 134.0, 12.020203, 2.5999999], [0.81118912, -12.115005, 104.0, 12.081173, -2.5999999]]  # Velo_64
                  }
                }
                n290 = for {
                  N: 12 -> [_]
                  shift-right: [w543] -> _
                  shift-left: w503 -> [w596]
                  tunnel: w502 -> [w584]
                  tunnel: [w544] -> w488 mode=concatenating
                  tunnel: [w541] -> w480 mode=concatenating
                  tunnel: w486 -> [w540]
                  i -> [w591]
                  w579 = 96 ("length (rest)")
                  n291 = Equal?(x=w584, y=u8 2) -> (x = y?=w585:bool)
                  n292 = Quotient & Remainder(x=w591, y=2) -> (x-y*floor(x/y)=w588:i32)  [unwired: 1 out]
                  n293 = Select(t=w588, s=w585, f=0) -> (s? t:f=w587:i32)
                  n294 = Multiply(x=32, y=w587) -> (x*y=w564:i32)
                  n295 = Array Subset(array=w540, index (row)=w564, length (row)=32 ("length")) -> (w562:dbl[][])  [unwired: 2 in]
                  n296 = Unflatten From String(type=T15 {"Laser block ID"=0, "Rotational position"=0}, binary string=w596, data includes array or string size? (T)=FALSE, byte order (0:big-endian, network order)=T10."native, host order") -> (rest of the binary string=w580:string, value=w595:T15)  [unwired: 1 in, 1 out]
                  n297 = Unbundle By Name(w595) -> ("Rotational position"=w592:u16)
                  n298 = String Subset(string=w580, offset (0)=w579) -> (substring=w543:string)  [unwired: 1 in]
                  n299 = String Subset(string=w580, length (rest)=w579) -> (substring=w578:string)  [unwired: 1 in]
                  n300 = Unflatten From String(type=u8[] [], binary string=w578, data includes array or string size? (T)=FALSE, byte order (0:big-endian, network order)=T10."native, host order") -> (value=w576:u8[])  [unwired: 1 in, 2 out]
                  n301 = Reshape Array(w576, 32 ("dimension size"), 3 ("dimension size")) -> (w573:u8[][])
                  n302 = Index Array(array=w573, index (col) #1=1 ("disabled index (col)"), index (col) #2=0 ("index (col)"), index (col) #3=2 ("index (col)")) -> (element #1=w571:u8[], element #2=w570:u8[], element #3=w541:u8[])  [unwired: 3 in]
                  n303 = Join Numbers(hi=w571, lo=w570) -> ((hi.lo)=w565:u16[])
                  n304 = To Double Precision Float(number=w592) -> (double precision float=w593:dbl)
                  n305 = To Double Precision Float(number=w565) -> (double precision float=w567:dbl[])
                  n306 = Multiply(x=w593, y=0.01) -> (x*y=w559:dbl)
                  n307 = Index Array(array=w562, index (col) #1=0 ("disabled index (col)"), index (col) #2=4 ("disabled index (col)"), index (col) #3=1 ("index (col)")) -> (element #1=w560:dbl[], element #2=w552:dbl[], element #3=w548:dbl[], element #4=w538:dbl[], element #5=w547:dbl[])  [unwired: 7 in]
                  n308 = Multiply(x=0.2, y=w567) -> (x*y=w539:dbl[])
                  n309 = Subtract(x=w559, y=w560) -> (x-y=w558:dbl[])
                  n310 = Add(x=w538, y=w539) -> (x+y=w546:dbl[])
                  n311 = Divide(x=w552, y=w546) -> (x/y=w553:dbl[])
                  n312 = Inverse Tangent(1:w553) -> (0:w554:dbl[])
                  n313 = Multiply(x=w554, y=180.0) -> (x*y=w556:dbl[])
                  n314 = Divide(x=w556, y=3.141592653589793) -> (x/y=w551:dbl[])
                  n315 = Subtract(x=w558, y=w551) -> (x-y=w550:dbl[])
                  n316 = Build Array(w550, w548, w546, w547) -> (w545:dbl[][])
                  n317 = Transpose 2D Array(2D array=w545) -> (transposed array=w544:dbl[][])
                }
                n318 = Index Array(array=w488, index (col) #1=0 ("disabled index (col)")) -> (element #1=w490:dbl[], element #2=w497:dbl[], element #3=w498:dbl[], element #4=w501:dbl[])  [unwired: 7 in]
                n319 = Multiply(x=3.141592653589793, y=w490) -> (x*y=w492:dbl[])
                n320 = Multiply(x=3.141592653589793, y=w497) -> (x*y=w495:dbl[])
                n321 = Multiply(x=w501, y=0.01) -> (x*y=w481:dbl[])
                n322 = Divide(x=w492, y=180.0) -> (x/y=w484:dbl[])
                n323 = Divide(x=w495, y=180.0) -> (x/y=w483:dbl[])
                n324 = Multiply(x=w498, y=0.01) -> (x*y=w482:dbl[])
                n325 = disable-structure shown="Enabled" {
                  disable-tunnel: [w517 w518] -> w487
                  disable-tunnel: w484 -> [w516 w527]
                  disable-tunnel: w483 -> [w515 w526]
                  disable-tunnel: w482 -> [w514 w520]
                  disable-tunnel: w481 -> [w513 w525]
                  disable-tunnel: w480 -> [w512 w519]
                  frame Enabled {
                    n326 = global read "G_LCM.vi" "POS_T"() -> (w509:T34)
                    n327 = Unbundle By Name(w509) -> ("y"=w508:dbl, "x"=w507:dbl, "heading"=w506:dbl)
                    n328 = Bundle By Name(cluster=T14 {"hash"=-1208058655852198207, "sys time"=0, "Timestamp"=0, "Rot_ang"=[], "Ver_ang"=[], "Dist"=[], "Ver_off"=[], "Intensity"=[], "pos x"=0.0, "pos y"=0.0, "Heading"=0.0} ("VELO_384"), "Rot_ang"=w516, "Ver_ang"=w515, "Dist"=w514, "Ver_off"=w513, "Intensity"=w512, "pos x"=w508, "pos y"=w507, "Heading"=w506) -> (w510:T14)
                    n329 = global read "G_LCM.vi" "queue velo"() -> (w511)
                    n330 = Enqueue Element(queue=w511, element=w510) -> (error out=w517:errorcluster)  [unwired: 2 in, 2 out]
                  }
                  frame Disabled {
                    n331 = Sine & Cosine(0:w527) -> (1:w529:dbl[], 2:w530:dbl[])
                    n332 = Sine & Cosine(0:w526) -> (1:w531:dbl[], 2:w528:dbl[])
                    n333 = Compound Arithmetic op=MULTIPLY(w520, w530, w528) -> (w523:dbl[])
                    n334 = Compound Arithmetic op=MULTIPLY(w529, w528, w520) -> (w524:dbl[])
                    n335 = Compound Arithmetic op=MULTIPLY(w531, w520) -> (w532:dbl[])
                    n336 = global read "G_SEN.vi" "velo_decode"() -> (w533:T35)
                    n337 = Add(x=w532, y=w525) -> (x+y=w522:dbl[])
                    n338 = global read "G_SEN.vi" "queue velo decode"() -> (w534:refnum<queue>)
                    n339 = Bundle By Name(cluster=w533, "i"=w519, "X"=w524, "Y"=w523, "Z"=w522, "d"=w520) -> (w521:T35)
                    n340 = Enqueue Element(queue=w534, element=w521) -> (error out=w518:errorcluster)  [unwired: 2 in, 2 out]
                  }
                }
                "error out 3" <- w487
              }
              frame Error {
              }
            }
          }
          frame "POS_T" {
            n341 = global read "G_LCM.vi" "POS_T"() -> (w603:T34)
            n342 = Unbundle By Name(w603) -> ("hash"=w601:i64)
            n343 = Unflatten From String(type=w603, binary string=w604, data includes array or string size? (T)=FALSE) -> (value=w602:T34, error out=w600:errorcluster)  [unwired: 2 in, 1 out]
            n344 = case shown="No Error" w600 {
              tunnel: w602 -> [w608 _]
              tunnel: w601 -> [w607 _]
              frame No Error {
                n345 = Bundle By Name(cluster=w608, "hash"=w607) -> (w606:T34)
                n346 = global write "G_LCM.vi" "POS_T"(w606) -> ()
              }
              frame Error {
              }
            }
          }
          frame "SICK_FRONT" {
            n347 = global read "G_LCM.vi" "SICK_FRONT"() -> (w612:T36)
            n348 = Unbundle By Name(w612) -> ("hash"=w610:i64)
            n349 = Unflatten From String(type=w612, binary string=w613, data includes array or string size? (T)=FALSE) -> (value=w611:T36, error out=w609:errorcluster)  [unwired: 2 in, 1 out]
            n350 = case shown="No Error" w609 {
              tunnel: w611 -> [w622 _]
              tunnel: w610 -> [w621 _]
              frame No Error {
                n351 = Bundle By Name(cluster=w622, "hash"=w621) -> (w615:T36)
                n352 = global write "G_LCM.vi" "SICK_FRONT"(w615) -> ()
                n353 = Unbundle By Name(w615) -> ("buff[meter]"=w616:sgl[], "n"=w617:i16)
                n354 = Delete From Array(array=w616, length=w617, index=0) -> (deleted portion=w620:sgl[], array with subset deleted=w619:sgl[])
                n355 = global write "G_LCM.vi" "SICK_FRONT_intensity"(w619) -> ()
                n356 = global write "G_LCM.vi" "SICK_FRONT_range"(w620) -> ()
              }
              frame Error {
              }
            }
          }
          frame "LOCALIZER_T", "SLAM" {
            n357 = global read "G_LCM.vi" "SLAM"() -> (w626:T34)
            n358 = Unbundle By Name(w626) -> ("hash"=w624:i64)
            n359 = Unflatten From String(type=w626, binary string=w627, data includes array or string size? (T)=FALSE) -> (value=w625:T34, error out=w623:errorcluster)  [unwired: 2 in, 1 out]
            n360 = case shown="Error" w623 {
              tunnel: w625 -> [w631 _]
              tunnel: w624 -> [w630 _]
              frame No Error {
                n361 = Bundle By Name(cluster=w631, "hash"=w630) -> (w629:T34)
                n362 = global write "G_LCM.vi" "SLAM"(w629) -> ()
              }
              frame Error {
              }
            }
          }
          frame "LANE_T" {
            n363 = Unflatten From String(type=cluster{"hash":i64, "sys time":i64, "n":i32} {"hash"=-8920902524919788889, "sys time"=0, "n"=0} ("LANE_T"), binary string=w639, data includes array or string size? (T)=FALSE) -> (rest of the binary string=w637:string, value=w640:cluster{"hash":i64, "sys time":i64, "n":i32}, error out=w634:errorcluster)  [unwired: 2 in]
            n364 = Unflatten From String(type=dbl[] [] ("data 2"), binary string=w637, data includes array or string size? (T)=FALSE, error in (no error)=w634) -> (value=w632:dbl[], error out=w633:errorcluster)  [unwired: 1 in, 1 out]
            n365 = case shown="No Error" w633 {
              tunnel: w640 -> [w655 _]
              tunnel: w632 -> [w652 _]
              frame No Error {
                n366 = Unbundle By Name(w655) -> ("sys time"=w654:i64, "n"=w646:i32)
                n367 = Delete From Array(array=w652, length=w646, index=0) -> (deleted portion=w650:dbl[], array with subset deleted=w648:dbl[])
                n368 = Delete From Array(array=w648, length=w646, index=0) -> (deleted portion=w647:dbl[], array with subset deleted=w645:dbl[])
                n369 = global read "G_LCM.vi" "LANE_T"() -> (w656:T37)
                n370 = Delete From Array(array=w645, length=w646, index=0) -> (deleted portion=w643:dbl[], array with subset deleted=w642:dbl[])
                n371 = Bundle By Name(cluster=w656, "sys time"=w654, "n"=w646, "lon"=w642, "lat"=w643, "data2"=w647, "data1"=w650) -> (w653:T37)
                n372 = global write "G_LCM.vi" "LANE_T"(w653) -> ()
              }
              frame Error {
              }
            }
          }
          frame "PATH_T" {
            n373 = Unflatten From String(type=T6 {"hash"=-8920902524919788889, "sys time"=3528569500002214, "n"=0, "pathxy"=[15.0, 175.0, 132.0, 243.0, 160.0, 0.0, 0.0, 1.0, 0.0, 0.0, 160.0, 18.0, 230.0, 6.0, 22.0, 255.0, 89.0, 1.0, 34.0, 1.0, 0.0, 0.0, 0.0, 0.0, 0.0, 0.0, 0.0, 0.0, 0.0, 0.0, 0.0, 0.0, 0.0, 0.0, 0.0, 0.0, 0.0, 0.0, 0.0, 0.0, 0.0, 0.0, 0.0, 0.0, 0.0, 0.0, 0.0, 0.0, 0.0, 0.0, 0.0, 0.0, 0.0, 0.0, 0.0, 0.0, 0.0, 0.0, 0.0, 0.0, 0.0, 0.0, 0.0, 0.0, 0.0, 0.0, 0.0, 0.0, 0.0, 0.0, 0.0, 0.0, 0.0, 0.0, 0.0, 0.0, 0.0, 0.0, 0.0, 0.0, 0.0, 0.0, 0.0, 0.0, 0.0, 0.0, 0.0, 0.0, 0.0, 0.0, 0.0, 0.0, 0.0, 0.0, 0.0, 0.0, 0.0, 0.0, 0.0, 0.0, 0.0, 0.0, 0.0, 0.0, 0.0]} ("PATH_T"), binary string=w659, data includes array or string size? (T)=FALSE) -> (value=w660:T6, error out=w657:errorcluster)  [unwired: 2 in, 1 out]
            n374 = case shown="No Error" w657 {
              tunnel: w660 -> [w667 _]
              frame No Error {
                n375 = Unbundle By Name(w667) -> ("sys time"=w665:i64, "pathxy"=w663:dbl[], "n"=w662:u32)
                n376 = global read "G_LCM.vi" "PATH_T"() -> (w666:T6)
                n377 = Bundle By Name(cluster=w666, "sys time"=w665, "pathxy"=w663, "n"=w662) -> (w664:T6)
                n378 = disable-structure shown="Enabled" {
                  disable-tunnel: w664 -> [w668 _]
                  frame Enabled {
                    n379 = global write "G_LCM.vi" "PATH_T"(w668) -> ()
                  }
                  frame Disabled {
                  }
                }
              }
              frame Error {
              }
            }
          }
          frame "ERROR_T" {
            n380 = Unflatten From String(type=T16 {"hash"=-3262420976274766845, "sys time"=0, "n"=0, "error"=[]} ("ERROR_T"), binary string=w671, data includes array or string size? (T)=FALSE) -> (value=w672:T16, error out=w670:errorcluster)  [unwired: 2 in, 1 out]
            n381 = case shown="No Error" w670 {
              tunnel: w672 -> [w679 _]
              frame No Error {
                n382 = Unbundle By Name(w679) -> ("sys time"=w677:i64, "error"=w675:i32[], "n"=w674:i32)
                n383 = global read "G_LCM.vi" "ERROR_T"() -> (w678:T16)
                n384 = Bundle By Name(cluster=w678, "sys time"=w677, "error"=w675, "n"=w674) -> (w676:T16)
                n385 = disable-structure shown="Enabled" {
                  disable-tunnel: w676 -> [w688 _]
                  frame Enabled {
                    n386 = global write "G_LCM.vi" "ERROR_T"(w688) -> ()
                    n387 = Unbundle By Name(w688) -> ("error"=w682:i32[])
                    n388 = global read "G_ALL.vi" "beep"() -> (w687:T38)
                    n389 = Unbundle By Name(w687) -> ("beep"=w686:bool)
                    n390 = Greater?(x=w682, y=10) -> (0:w681:bool[])
                    n391 = Or Array Elements(Boolean array=w681) -> (logical OR=w684:bool)
                    n392 = Not(x=w686) -> (.not. x?=w685:bool)
                    n393 = And(x=w685, y=w684) -> (x .and. y?=w683:bool)
                    n394 = case shown="True" w683 {
                      frame False {
                      }
                      frame True {
                        n395 = global read "G_ALL.vi" "beep"() -> (w689:T38)
                        n396 = Bundle By Name(cluster=w689, "beep"=TRUE ("use system alert? (T)")) -> (w690:T38)
                        n397 = global write "G_ALL.vi" "beep"(w690) -> ()
                      }
                    }
                  }
                  frame Disabled {
                  }
                }
              }
              frame Error {
              }
            }
          }
          frame "FLEA3_CURRENT" {
            n398 = String Length(string=w692) -> (length=→"length":i32)
          }
          frame "GGA_1" {
            n399 = global read "G_LCM.vi" "GGA_1"() -> (w697:T39)
            n400 = Unbundle By Name(w697) -> ("hash"=w695:i64)
            n401 = Unflatten From String(type=w697, binary string=w698, data includes array or string size? (T)=FALSE) -> (value=w696:T39, error out=w694:errorcluster)  [unwired: 2 in, 1 out]
            n402 = case shown="No Error" w694 {
              tunnel: w696 -> [w702 _]
              tunnel: w695 -> [w701 _]
              frame No Error {
                n403 = flat-sequence {
                  tunnel: w702 -> [w705]
                  tunnel: w701 -> [w704]
                  tunnel: [w703] -> w700
                  tunnel: w700 -> [w716]
                  frame #0 {
                    n404 = Bundle By Name(cluster=w705, "hash"=w704) -> (w703:T39)
                    n405 = global write "G_LCM.vi" "GGA_1"(w703) -> ()
                  }
                  frame #1 {
                    n406 = Unbundle By Name(w716) -> ("sys time"=w714:i64, "lat"=w713:dbl, "lon"=w712:dbl)
                    n407 = local read "SDT_GPS_DATA"() -> (w715:T5)
                    n408 = Bundle By Name(cluster=w715, "sys time"=w714, "lat"=w713, "lon"=w712) -> (w710:T5)
                    n409 = Flatten To String(anything=w710, prepend array or string size? (T)=FALSE) -> (data string=w707:string, error out=→"error out":errorcluster)  [unwired: 2 in, 1 out]
                    n410 = global read "G_LCM.vi" "LCM"() -> (w709:T11)
                    n411 = call "LCM_send.vi"("DATA"=w707, "ID"="SDT_GPS_DATA", "LCM"=w709) -> ()  [unwired: 7 in, 2 out]
                  }
                }
              }
              frame Error {
              }
            }
          }
          frame "GGA_2" {
            n412 = global read "G_LCM.vi" "GGA_2"() -> (w720:T39)
            n413 = Unbundle By Name(w720) -> ("hash"=w718:i64)
            n414 = Unflatten From String(type=w720, binary string=w721, data includes array or string size? (T)=FALSE) -> (value=w719:T39, error out=w717:errorcluster)  [unwired: 2 in, 1 out]
            n415 = case shown="No Error" w717 {
              tunnel: w719 -> [w725 _]
              tunnel: w718 -> [w724 _]
              frame No Error {
                n416 = Bundle By Name(cluster=w725, "hash"=w724) -> (w723:T39)
                n417 = global write "G_LCM.vi" "GGA_2"(w723) -> ()
              }
              frame Error {
              }
            }
          }
          frame "APP_GPS_DATA" {
            n418 = global read "G_LCM.vi" "APP_GPS_DATA"() -> (w729:T40)
            n419 = Unbundle By Name(w729) -> ("hash"=w727:i64)
            n420 = Unflatten From String(type=w729, binary string=w730, data includes array or string size? (T)=FALSE) -> (value=w728:T40, error out=w726:errorcluster)  [unwired: 2 in, 1 out]
            n421 = case shown="No Error" w726 {
              tunnel: w728 -> [w734 _]
              tunnel: w727 -> [w733 _]
              frame No Error {
                n422 = Bundle By Name(cluster=w734, "hash"=w733) -> (w732:T40)
                n423 = global write "G_LCM.vi" "APP_GPS_DATA"(w732) -> ()
              }
              frame Error {
              }
            }
          }
          frame "EURECAR_VISION" {
            n424 = Unflatten From String(type=T17 {"hash"=4202194748993759695, "sys time"=0, "status"=0, "TS_num"=0} ("EURECAR_VISION"), binary string=w739, data includes array or string size? (T)=FALSE) -> (rest of the binary string=w735:string, value=w738:T17, error out=w737:errorcluster)  [unwired: 2 in]
            n425 = case shown="No Error" w737 {
              tunnel: w738 -> [w761 _]
              tunnel: w735 -> [w754 _]
              frame No Error {
                n426 = Unbundle By Name(w761) -> ("sys time"=w743:i64, "status"=w742:i32, "TS_num"=w744:i32)
                n427 = Multiply(x=4, y=w744) -> (x*y=w753:i32)
                n428 = String Subset(string=w754, offset (0)=w753) -> (substring=w752:string)  [unwired: 1 in]
                n429 = String Subset(string=w754, offset (0)=0, length (rest)=w753) -> (substring=w758:string)
                n430 = Unflatten From String(type=dbl[] [] ("TS_loc_x"), binary string=w752, data includes array or string size? (T)=FALSE) -> (value=w748:dbl[])  [unwired: 2 in, 2 out]
                n431 = global read "G_LCM.vi" "EURECAR_VISION"() -> (w756:T41)
                n432 = Delete From Array(array=w748, length=w744, index=0) -> (deleted portion=w745:dbl[], array with subset deleted=w746:dbl[])
                n433 = Unflatten From String(type=i32[] [] ("TS_type"), binary string=w758, data includes array or string size? (T)=FALSE) -> (value=w755:i32[])  [unwired: 2 in, 2 out]
                n434 = Bundle By Name(cluster=w756, "sys time"=w743, "status"=w742, "TS_num"=w744, "TS_type"=w755, "TS_loc_y"=w746, "TS_loc_x"=w745) -> (w741:T41)
                n435 = global write "G_LCM.vi" "EURECAR_VISION"(w741) -> ()
              }
              frame Error {
              }
            }
          }
          frame "vision_lane" {
            n436 = global read "G_LCM.vi" "VISION_LANE"() -> (w766:T42)
            n437 = Unbundle By Name(w766) -> ("hash"=w764:i64)
            n438 = Unflatten From String(type=w766, binary string=w762, data includes array or string size? (T)=FALSE) -> (value=w765:T42, error out=w763:errorcluster)  [unwired: 2 in, 1 out]
            n439 = case shown="No Error" w763 {
              tunnel: w765 -> [w770 _]
              tunnel: w764 -> [w769 _]
              frame No Error {
                n440 = Bundle By Name(cluster=w770, "hash"=w769) -> (w768:T42)
                n441 = global write "G_LCM.vi" "VISION_LANE"(w768) -> ()
              }
              frame Error {
              }
            }
          }
          frame "vision_front_cam" {
            n442 = global read "G_LCM.vi" "VISION_FRONT_CAM"() -> (w775:T43)
            n443 = Unbundle By Name(w775) -> ("hash"=w773:i64)
            n444 = Unflatten From String(type=w775, binary string=w771, data includes array or string size? (T)=FALSE) -> (value=w774:T43, error out=w772:errorcluster)  [unwired: 2 in, 1 out]
            n445 = case shown="No Error" w772 {
              tunnel: w774 -> [w779 _]
              tunnel: w773 -> [w778 _]
              frame No Error {
                n446 = Bundle By Name(cluster=w779, "hash"=w778) -> (w777:T43)
                n447 = global write "G_LCM.vi" "VISION_FRONT_CAM"(w777) -> ()
              }
              frame Error {
              }
            }
          }
          frame "vision_lane_pt" {
            n448 = global write "G_LCM.vi" "Mobileye name"(w780) -> ()
            n449 = global read "G_LCM.vi" "VISION_LANE_PT"() -> (w781:T44)
            n450 = Unbundle(w781) -> ("hash"=w785:i64, "sys time"=w784:i64, "size"=w783:i64)  [unwired: 3 out]
            n451 = Bundle("hash"=w785, "sys time"=w784, "size"=w783) -> (w782:cluster{"hash":i64, "sys time":i64, "size":i64})  [unwired: 1 in]
            n452 = Unflatten From String(type=w782, binary string=w787, data includes array or string size? (T)=FALSE) -> (rest of the binary string=w786:string, value=w789:cluster{"hash":i64, "sys time":i64, "size":i64}, error out=w788:errorcluster)  [unwired: 2 in]
            n453 = case shown="No Error" w788 {
              tunnel: w789 -> [w815 _]
              tunnel: w786 -> [w819 _]
              tunnel: w781 -> [w814 _]
              frame No Error {
                n454 = Unbundle By Name(w815) -> ("size"=w797:i64, "sys time"=w812:i64)
                n455 = Multiply(x=w797, y=i64 2) -> (x*y=w800:i64)
                n456 = Unflatten From String(type=dbl[] [], binary string=w819, data includes array or string size? (T)=FALSE) -> (value=w801:dbl[])  [unwired: 2 in, 2 out]
                n457 = Delete From Array(array=w801, length=w800, index=0) -> (deleted portion=w798:dbl[], array with subset deleted=w791:dbl[])
                n458 = Type Cast(type=i32[] [], x=w791) -> (*(type *) &x=w792:i32[])
                n459 = Delete From Array(array=w798, length=w797, index=0) -> (deleted portion=w794:dbl[], array with subset deleted=w795:dbl[])
                n460 = Divide(x=w794, y=3.0) -> (x/y=w802:dbl[])
                n461 = Subtract(x=w795, y=450.0) -> (x-y=w810:dbl[])
                n462 = Subtract(x=w802, y=117.0) -> (x-y=w806:dbl[])
                n463 = Multiply(x=-0.02, y=w810) -> (x*y=w808:dbl[])
                n464 = Multiply(x=w806, y=0.02) -> (x*y=w803:dbl[])
                n465 = Bundle By Name(cluster=w814, "y"=w808, "x"=w803, "size"=w797, "sys time"=w812, "point_flag"=w792) -> (w813:T44)
                n466 = global write "G_LCM.vi" "VISION_LANE_PT"(w813) -> ()
              }
              frame Error {
              }
            }
          }
          frame "LSTONE_T" {
            n467 = global read "G_LCM.vi" "lstone_t"() -> (w821)
            n468 = Unbundle By Name(w821) -> ("hash"=w824, "sys time"=w823, "n"=w820)  [unwired: 2 out]
            n469 = Bundle("hash"=w824, "sys time"=w823, "n"=w820) -> (w822:cluster{"hash":void, "sys time":void, "n":void})  [unwired: 1 in]
            n470 = Unflatten From String(type=w822, binary string=w826, data includes array or string size? (T)=FALSE) -> (rest of the binary string=w825:string, value=w828:cluster{"hash":void, "sys time":void, "n":void}, error out=w827:errorcluster)  [unwired: 2 in]
            n471 = case shown="No Error" w827 {
              tunnel: w828 -> [w840 _]
              tunnel: w825 -> [w846 _]
              tunnel: w821 -> [w843 _]
              frame No Error {
                n472 = Unbundle By Name(w840) -> ("n"=w835, "sys time"=w836)
                n473 = for {
                  N: w835 -> [_]
                  shift-right: [w858] -> w844
                  shift-left: w846 -> [w859]
                  tunnel: [w855] -> w839 mode=indexing
                  tunnel: [w856] -> w838
                  tunnel: [w854] -> w834 mode=indexing
                  tunnel: [w853] -> w833 mode=indexing
                  tunnel: [w852] -> w832 mode=indexing
                  n474 = Unflatten From String(type=T18 {"sys time"=0, "x"=0.0, "y"=0.0, "z"=0.0} ("element"), binary string=w859, data includes array or string size? (T)=FALSE) -> (rest of the binary string=w858:string, value=w855:T18, error out=w856:errorcluster)  [unwired: 2 in]
                  n475 = Unbundle By Name(w855) -> ("y"=w854:sgl, "x"=w853:sgl, "z"=w852:sgl)
                }
                n476 = Unflatten From String(type=i64[] [] ("Istone_dir"), binary string=w844, data includes array or string size? (T)=FALSE, error in (no error)=w838) -> (value=w831:i64[], error out=w837:errorcluster)  [unwired: 1 in, 1 out]
                n477 = Bundle By Name(cluster=w843, "buffer(label,side,group)"=w831, "Istone"=w839, "n"=w835, "sys time"=w836) -> (w842:cluster{})
                n478 = Build Array(w834, w833, w832, w831) -> (w830:sgl[][])
                n479 = case shown="No Error" w837 {
                  tunnel: w842 -> [w850 _]
                  tunnel: w830 -> [w849 _]
                  frame No Error {
                    n480 = To Double Precision Float(number=w849) -> (double precision float=w848:dbl[][])
                    n481 = disable-structure shown="Disabled" {
                      disable-tunnel: w850 -> [w851 _]
                      frame Disabled {
                        n482 = global write "G_LCM.vi" "lstone_t"(w851) -> ()
                      }
                      frame Enabled {
                      }
                    }
                    n483 = Transpose 2D Array(2D array=w848) -> (transposed array=w847:dbl[][])
                    n484 = global write "G_SEN.vi" "LSTONE"(w847) -> ()
                  }
                  frame Error {
                  }
                }
              }
              frame Error {
              }
            }
          }
          frame "vision_stopline" {
            n485 = global read "G_LCM.vi" "VISION_STOPLINE"() -> (w865:T45)
            n486 = Unbundle By Name(w865) -> ("hash"=w863:i64)
            n487 = Unflatten From String(type=w865, binary string=w861, data includes array or string size? (T)=FALSE) -> (value=w864:T45, error out=w862:errorcluster)  [unwired: 2 in, 1 out]
            n488 = case shown="No Error" w862 {
              tunnel: w864 -> [w869 _]
              tunnel: w863 -> [w868 _]
              frame No Error {
                n489 = Bundle By Name(cluster=w869, "hash"=w868) -> (w867:T45)
                n490 = global write "G_LCM.vi" "VISION_STOPLINE"(w867) -> ()
              }
              frame Error {
              }
            }
          }
          frame "RMC_1" {
            n491 = global read "G_LCM.vi" "RMC_1"() -> (w873:T46)
            n492 = Unbundle By Name(w873) -> ("hash"=w871:i64)
            n493 = Unflatten From String(type=w873, binary string=w874, data includes array or string size? (T)=FALSE) -> (value=w872:T46, error out=w870:errorcluster)  [unwired: 2 in, 1 out]
            n494 = case shown="No Error" w870 {
              tunnel: w872 -> [w878 _]
              tunnel: w871 -> [w877 _]
              frame No Error {
                n495 = Bundle By Name(cluster=w878, "hash"=w877) -> (w876:T46)
                n496 = global write "G_LCM.vi" "RMC_1"(w876) -> ()
              }
              frame Error {
              }
            }
          }
          frame "RMC_2" {
            n497 = global read "G_LCM.vi" "RMC_2"() -> (w882:T46)
            n498 = Unbundle By Name(w882) -> ("hash"=w880:i64)
            n499 = Unflatten From String(type=w882, binary string=w883, data includes array or string size? (T)=FALSE) -> (value=w881:T46, error out=w879:errorcluster)  [unwired: 2 in, 1 out]
            n500 = case shown="No Error" w879 {
              tunnel: w881 -> [w887 _]
              tunnel: w880 -> [w886 _]
              frame No Error {
                n501 = Bundle By Name(cluster=w887, "hash"=w886) -> (w885:T46)
                n502 = global write "G_LCM.vi" "RMC_2"(w885) -> ()
              }
              frame Error {
              }
            }
          }
        }
        n503 = case shown="Default" w136 {
          selector: w136 -> [_ w138]
          frame "" {
          }
          frame Default {
            n504 = Concatenate Strings(w138, "\t") -> (w139:string)
            n505 = global read "G_LCM.vi" "recv data"() -> (w144:string)
            n506 = Match Pattern(string=w144, regular expression=w139) -> (before substring=w143:string, match substring=w142:string, after substring=w141:string, offset past match=w146:i32)  [unwired: 1 in]
            n507 = case shown="0, Default" w146 {
              tunnel: w143 -> [w150 w158]
              tunnel: w142 -> [w149 _]
              tunnel: w141 -> [w148 _]
              tunnel: [w147 w160] -> w140
              tunnel: w139 -> [_ w159]
              frame 0, Default {
                n508 = Match Pattern(string=w148, regular expression="\r") -> (before substring=w157:string, match substring=w153:string, after substring=w154:string)  [unwired: 1 in, 1 out]
                n509 = Decimal String To Number(string=w157) -> (number=w152:i32)  [unwired: 2 in, 1 out]
                n510 = Increment(x=w152) -> (x+1=w156:i32)
                n511 = Number To Decimal String(number=w156) -> (decimal integer string=w155:string)  [unwired: 1 in]
                n512 = Concatenate Strings(w150, w149, w155, w153, w154) -> (w147:string)
              }
              frame -1 {
                n513 = Concatenate Strings(w159, "1", "\r", w158) -> (w160:string)
              }
            }
            n514 = global write "G_LCM.vi" "recv data"(w140) -> ()
          }
        }
      }
      n515 = case shown="True" "velodyne enable" {
        frame False {
        }
        frame True {
          n516 = UDP Open(9:10 ("timeout ms (25000)"), 11:u16 2368 ("Sensor Port 2")) -> (port=w890:refnum<k16>, 0:w892:errorcluster)  [unwired: 3 in, 1 out]
          n517 = call "UDP_set_receive_buffer.vi"("error in (no error)"=w892, "Receive Buffer Size"=u32 12480, "connection ID"=w890) -> ("error out"=w893:errorcluster, "connection ID out"=w889:refnum<k16>)  [unwired: 6 in]
          n518 = call "UDP_read_receive_buffer.vi"("error in (no error)"=w893, "connection ID"=w889) -> ("error out"=w891:errorcluster, "connection ID out"=w888:refnum<k16>)  [unwired: 5 in, 1 out]
          n519 = while {
            tunnel: [w906] -> w895
            tunnel: w891 -> [w905]
            tunnel: w888 -> [w904]
            stop <- FALSE stop-if-true
            n520 = UDP Read(connection ID=w904, max size (548)=1248 ("bytes to read"), timeout ms (25000)=1000, 8:w905) -> (data out=w899:string, error out=w898:errorcluster, 3:w906:refnum<k16>)  [unwired: 2 out]
            n521 = case shown="No Error" w898 {
              selector: w898 -> [w908 w920]
              tunnel: w899 -> [_ w909]
              tunnel: [w908 w925] -> w902
              frame Error {
                n522 = Wait Until Next ms Multiple(millisecond multiple=u32 10000) -> ()  [unwired: 1 out]
              }
              frame No Error {
                n523 = Get Date/Time In Seconds() -> (seconds since 1Jan1904=w916:timestamp)
                n524 = To Double Precision Float(number=w916) -> (double precision float=w917:dbl)
                n525 = local read "Velodyne1"() -> (w912:T3)
                n526 = Multiply(x=w917, y=1000000.0) -> (x*y=w919:dbl)
                n527 = local read "VELO_RAW"() -> (w910:T2)
                n528 = To Quad Integer(1:w919) -> (0:w915:i64)
                n529 = To Unsigned Byte Integer(number=w912) -> (unsigned 8bit integer=w911:u8)
                n530 = Bundle By Name(cluster=w910, "sys time"=w915, "raw"=w909, "type"=w911) -> (w913:T2)
                n531 = Flatten To String(anything=w913, prepend array or string size? (T)=FALSE, error in (no error)=w920) -> (data string=w924:string, error out=w921:errorcluster)  [unwired: 1 in, 1 out]
                n532 = global read "G_LCM.vi" "LCM"() -> (w922:T11)
                n533 = call "LCM_send.vi"("error in (no error)"=w921, "DATA"=w924, "ID"="VELO_RAW", "LCM"=w922) -> ("error out"=w925:errorcluster)  [unwired: 6 in, 1 out]
              }
            }
            "veodyne error out" <- w902
          }
          n534 = UDP Close(connection ID=w895) -> ()  [unwired: 1 in, 2 out]
        }
      }
      n535 = while {
        tunnel: [w935] -> w130
        shift-right: [w933] -> _
        shift-left: FALSE -> [w934]
        stop <- w932 continue-if-true
        n536 = Wait Until Next ms Multiple(millisecond multiple=u32 5000) -> ()  [unwired: 1 out]
        n537 = Select(t="10.152.36.11" ("address"), s=w934, f="192.168.100.1" ("address")) -> (s? t:f=w926:string)
        n538 = TCP Open Connection(address=w926, remote port or service name=u16 12002 ("Sensor Port 2"), timeout ms (60000)=10 ("timeout ms (25000)")) -> (connection ID=w935:refnum<k5>, error out=w932:errorcluster)  [unwired: 2 in]
        n539 = Not(x=w934) -> (.not. x?=w933:bool)
      }
      n540 = while {
        tunnel: w130 -> [w959]
        tunnel: [w943] -> w132
        stop <- FALSE stop-if-true
        w955 = u8[] [175, 254, 192, 194] ("value")
        n541 = TCP Read(connection ID=w959, bytes to read=4 ("count (1)"), 9:1000 ("timeout ms (25000)")) -> (connection ID out=w952:refnum<k5>, data out=w951:string, error out=w954:errorcluster)  [unwired: 2 in]
        n542 = Unflatten From String(type=w955, binary string=w951, data includes array or string size? (T)=FALSE, error in (no error)=w954) -> (value=w936:u8[], error out=w953:errorcluster)  [unwired: 1 in, 1 out]
        n543 = Equal?(x=w955, y=w936) -> (x = y?=w937:bool[])
        n544 = Empty Array?(array=w936) -> (empty?=w941:bool)
        n545 = And Array Elements(Boolean array=w937) -> (logical AND=w939:bool)
        n546 = Not(x=w941) -> (.not. x?=w940:bool)
        n547 = case shown="True" w939 {
          tunnel: w952 -> [w1014 w1036]
          tunnel: [w1013 w1031] -> w947
          tunnel: w953 -> [w1012 w1030]
          tunnel: [w1011 w1021] -> w957
          frame False {
            n548 = TCP Read(connection ID=w1014, bytes to read=9999999, error in (no error)=w1012, 7:T21."Immediate" ("mode (standard)"), 9:10 ("timeout ms (25000)")) -> (connection ID out=w1013:refnum<k5>, error out=w1011:errorcluster)  [unwired: 1 out]
          }
          frame True {
            n549 = TCP Read(connection ID=w1036, bytes to read=20 ("count (1)"), error in (no error)=w1030, 9:10 ("timeout ms (25000)")) -> (connection ID out=w1032:refnum<k5>, data out=w1024:string, error out=w1029:errorcluster)  [unwired: 1 in]
            n550 = Unflatten From String(type=T9 {"Size of prev messages"=20, "Size of this messages"=20, "Reserved"=20, "DeviceID"=20, "Data type"=20, "NTP time"=20} ("Header"), binary string=w1024, data includes array or string size? (T)=FALSE, error in (no error)=w1029) -> (value=w1018:T9, error out=w1028:errorcluster)  [unwired: 1 in, 1 out]
            "header" <- w1018
            n551 = Unbundle By Name(w1018) -> ("Data type"=w1023:u16, "Size of this messages"=w1020:u32)
            n552 = To Long Integer(number=w1020) -> (32bit integer=w1019:i32)
            n553 = TCP Read(connection ID=w1032, bytes to read=w1019, error in (no error)=w1028, 9:1000 ("timeout ms (25000)")) -> (connection ID out=w1031:refnum<k5>, data out=w1025:string, error out=w1022:errorcluster)  [unwired: 1 in]
            n554 = case shown="2202" w1023 {
              tunnel: w1025 -> [_ w1053]
              tunnel: w1022 -> [_ w1052]
              tunnel: [_ w1051] -> w1021
              frame Default {
              }
              frame 8706 {
                w1043 = T47 {"Scan number"=0, "scanner status"=0, "Sync phase offset"=0, "Scan start time NTP"=0, "Scan end time NTP"=0, "Angle ticks per rotation"=0, "Start angle"=0, "End angle"=0, "Scan points"=0, "Mounting position yaw angle "=0, "Mounting position pitch angle"=0, "Mounting position roll angle"=0, "Mounting position x"=0, "Mounting position y"=0, "Mounting position z"=0, "Reserved"=0}  # Scan header
                n555 = String Subset(string=w1053, offset (0)=u16 44 ("y")) -> (substring=w1044:string)  [unwired: 1 in]
                n556 = String Subset(string=w1053, length (rest)=44 ("length (rest)")) -> (substring=w1046:string)  [unwired: 1 in]
                n557 = Unflatten From String(type=w1043, binary string=w1046, data includes array or string size? (T)=FALSE, byte order (0:big-endian, network order)=T10."little-endian", error in (no error)=w1052) -> (value=w1050:T47, error out=w1040:errorcluster)  [unwired: 1 out]
                n558 = flat-sequence {
                  tunnel: w1050 -> [w1089]
                  tunnel: [w1088] -> w1049
                  frame #0 {
                    w1087 = T48 {"Scan number"=0, "scanner status"=0, "Sync phase offset"=0, "Scan start time NTP"=0, "Scan end time NTP"=0, "Angle ticks per rotation"=0, "Start angle"=0.0, "End angle"=0.0, "Scan points"=0, "Mounting position yaw angle "=0.0, "Mounting position pitch angle"=0.0, "Mounting position roll angle"=0.0, "Mounting position x"=0.0, "Mounting position y"=0.0, "Mounting position z"=0.0, "Reserved"=0}  # Scan header
                    n559 = Unbundle(w1089) -> ("Scan number"=w1086:u16, "scanner status"=w1085:u16, "Sync phase offset"=w1084:u16, "Scan start time NTP"=w1083:u64, "Scan end time NTP"=w1082:u64, "Angle ticks per rotation"=w1073:u16, "Start angle"=w1079:i16, "End angle"=w1078:i16, "Scan points"=w1080:u16, "Mounting position yaw angle"=w1077:i16, "Mounting position pitch angle"=w1076:i16, "Mounting position roll angle"=w1075:i16, "Mounting position x"=w1068:i16, "Mounting position y"=w1067:i16, "Mounting position z"=w1066:i16, "Reserved"=w1058:u16)
                    n560 = Build Array(w1079, w1078, w1077, w1076, w1075) -> (w1074:i16[])
                    n561 = Build Array(w1068, w1067, w1066) -> (w1065:i16[])
                    n562 = Divide(x=w1074, y=w1073) -> (x/y=w1081:dbl[])
                    n563 = Multiply(x=w1081, y=6.283185307179586) -> (x*y=w1057:dbl[])
                    n564 = disable-structure shown="Enabled" {
                      disable-tunnel: w1057 -> [w1093 _]
                      disable-tunnel: [w1092 w1097] -> w1056
                      disable-tunnel: [w1091 w1096] -> w1055
                      disable-tunnel: [w1090 w1095] -> w1054
                      frame Disabled {
                        n565 = Index Array(array=w1093, index #1=2 ("index")) -> (element #1=w1092:dbl, element #2=w1091:dbl, element #3=w1090:dbl)  [unwired: 2 in]
                      }
                      frame Enabled {
                        n566 = global read "G_LCM.vi" "POS_T"() -> (w1098:T34)
                        n567 = Unbundle By Name(w1098) -> ("y"=w1097:dbl, "x"=w1096:dbl, "heading"=w1095:dbl)
                      }
                    }
                    n568 = Index Array(array=w1057, index #1=0 ("index")) -> (element #1=w1070:dbl, element #2=w1069:dbl)  [unwired: 1 in]
                    n569 = Multiply(x=w1065, y=0.01) -> (x*y=w1063:dbl[])
                    n570 = Index Array(array=w1063, index #1=0 ("index")) -> (element #1=w1061:dbl, element #2=w1060:dbl, element #3=w1059:dbl)  [unwired: 2 in]
                    n571 = Bundle(cluster=w1087, "Scan number"=w1086, "scanner status"=w1085, "Sync phase offset"=w1084, "Scan start time NTP"=w1083, "Scan end time NTP"=w1082, "Angle ticks per rotation"=w1073, "Start angle"=w1070, "End angle"=w1069, "Scan points"=w1080, "Mounting position yaw angle"=w1056, "Mounting position pitch angle"=w1055, "Mounting position roll angle"=w1054, "Mounting position x"=w1061, "Mounting position y"=w1060, "Mounting position z"=w1059, "Reserved"=w1058) -> (w1088:T48)
                  }
                }
                n572 = Unbundle By Name(w1050) -> ("Scan points"=w1038:u16, "Angle ticks per rotation"=w1041:u16)
                n573 = for {
                  N: w1038 -> [_]
                  shift-right: [w1135] -> _
                  shift-left: w1044 -> [w1138]
                  tunnel: w1041 -> [w1122]
                  shift-right: [w1117] -> w1037
                  shift-left: w1040 -> [w1118]
                  tunnel: [w1099] -> w1048 mode=indexing
                  w1129 = T32 {"flags"=0, "Echo"=0, "Radial distance"=0.0, "Horizontal angle"=0.0, "Vertical angle"=0.0, "Echo pulse width"=0, "Reserved"=0}  # Scan point
                  w1136 = T49 {"Layer/Echo"=0, "flags"=0, "Horizontal angle"=0, "Radial distance"=0, "Echo pulse width"=0, "Reserved"=0}  # scan point
                  n574 = Unflatten From String(type=w1136, binary string=w1138, data includes array or string size? (T)=FALSE, byte order (0:big-endian, network order)=T10."little-endian", error in (no error)=w1118) -> (rest of the binary string=w1135:string, value=w1134:T49, error out=w1117:errorcluster)
                  n575 = Unbundle(w1134) -> ("Layer/Echo"=w1124:u8, "flags"=w1101:u8, "Horizontal angle"=w1123:i16, "Radial distance"=w1105:u16, "Echo pulse width"=w1112:u16, "Reserved"=w1111:u16)
                  n576 = Divide(x=w1123, y=w1122) -> (x/y=w1121:dbl)
                  n577 = Logical Shift(y=i16 4, x=w1101) -> (x << y=w1103:u8)
                  n578 = Logical Shift(y=i16 4, x=w1124) -> (x << y=w1132:u8)
                  n579 = Logical Shift(y=i16 -4, x=w1103) -> (x << y=w1100:u8)
                  n580 = Logical Shift(y=i16 -4, x=w1132) -> (x << y=w1128:u8)
                  n581 = Multiply(x=0.8, y=w1128) -> (x*y=w1126:dbl)
                  n582 = Multiply(x=w1105, y=0.01) -> (x*y=w1114:dbl)
                  n583 = Logical Shift(y=i16 -4, x=w1124) -> (x << y=w1115:u8)
                  n584 = Subtract(x=w1126, y=1.2) -> (x-y=w1110:dbl)
                  n585 = Multiply(x=3.141592653589793, y=w1110) -> (x*y=w1108:dbl)
                  n586 = Multiply(x=w1121, y=6.283185307179586) -> (x*y=w1113:dbl)
                  n587 = Divide(x=w1108, y=180.0) -> (x/y=w1106:dbl)
                  n588 = Bundle(cluster=w1129, "flags"=w1100, "Echo"=w1115, "Radial distance"=w1114, "Horizontal angle"=w1113, "Vertical angle"=w1106, "Echo pulse width"=w1112, "Reserved"=w1111) -> (w1099:T32)
                }
                n589 = case shown="No Error" w1037 {
                  selector: w1037 -> [w1139 _]
                  tunnel: w1049 -> [w1141 _]
                  tunnel: [w1166 _] -> w1051
                  tunnel: w1048 -> [w1140 _]
                  frame No Error {
                    n590 = Get Date/Time In Seconds() -> (seconds since 1Jan1904=w1164:timestamp)
                    n591 = To Double Precision Float(number=w1164) -> (double precision float=w1163:dbl)
                    n592 = Multiply(x=w1163, y=1000000.0) -> (x*y=w1161:dbl)
                    n593 = local read "IBEO_2202_T"() -> (w1159:T8)
                    n594 = local read "header"() -> (w1165:T9)
                    n595 = To Quad Integer(1:w1161) -> (0:w1160:i64)
                    n596 = Bundle By Name(cluster=w1159, "sys time"=w1160, "Header"=w1165, "Scan header"=w1141, "Scan points"=w1140) -> (w1158:T8)
                    n597 = Unbundle(w1158) -> ("hash"=w1152:i64, "sys time"=w1151:i64, "Header"=w1144:T9, "Scan header"=w1150:T29, "Scan points"=w1145:T30)
                    n598 = Array Size(array=w1145) -> (size(s)=w1143:i32)
                    n599 = Bundle By Name(cluster=w1144, "Size of this messages"=w1143) -> (w1142:T9)
                    n600 = for {
                      N: w1143 -> [_]
                      tunnel: w1145 -> [w1167] mode=indexing
                      shift-right: [w1168] -> w1146
                      shift-left: "" -> [w1170]
                      n601 = Flatten To String(anything=w1167, prepend array or string size? (T)=FALSE) -> (data string=w1169:string)  [unwired: 2 in, 2 out]
                      n602 = Concatenate Strings(w1170, w1169) -> (w1168:string)
                    }
                    n603 = Bundle("hash"=w1152, "sys time"=w1151, "Header"=w1142, "Scan header"=w1150) -> (w1153:T31)  [unwired: 1 in]
                    n604 = Flatten To String(anything=w1153, prepend array or string size? (T)=FALSE, error in (no error)=w1139) -> (data string=w1147:string, error out=w1155:errorcluster)  [unwired: 1 in, 1 out]
                    n605 = Concatenate Strings(w1147, w1146) -> (w1154:string)
                    n606 = global read "G_LCM.vi" "LCM"() -> (w1156:T11)
                    n607 = call "LCM_send.vi"("error in (no error)"=w1155, "DATA"=w1154, "ID"="IBEO_2202_T", "LCM"=w1156) -> ("error out"=w1166:errorcluster)  [unwired: 6 in, 1 out]
                  }
                  frame Error {
                  }
                }
              }
            }
          }
        }
        "Ibeo error out" <- w957
        n608 = And(x=w939, y=w940) -> (x .and. y?=w938:bool)
        n609 = global write "G_LCM.vi" "ibeo"(w938) -> ()
        n610 = case shown="True" "setdata" {
          tunnel: [w990 w1009] -> w946
          tunnel: w947 -> [w990 w1009]
          frame False {
          }
          frame True {
            w996 = T10."little-endian" ("byte order (0:big-endian, network order)")
            n611 = Bundle By Name(cluster=T20 {"command id"=16, "Reserved"=0, "parameter idx"=0} ("Header"), "parameter idx"="parameter idx") -> (w1005:T20)
            n612 = Build Array("Mouting", i16 0) -> ()  [unwired: 1 out]
            n613 = Flatten To String(anything=w1005, prepend array or string size? (T)=FALSE, byte order (0:big-endian, network order)=w996) -> (data string=w995:string)  [unwired: 1 in, 2 out]
            n614 = Flatten To String(anything="Mouting", prepend array or string size? (T)=FALSE, byte order (0:big-endian, network order)=w996) -> (data string=w994:string)  [unwired: 1 in, 2 out]
            n615 = Concatenate Strings(w995, w994) -> (w993:string)
            n616 = String Length(string=w993) -> (length=w1002:i32)
            n617 = To Unsigned Long Integer(number=w1002) -> (unsigned 32bit integer=w1001:u32)
            n618 = Bundle By Name(cluster=T19 {"Magic word"=2952708290, "Size of prev messages"=0, "Size of this messages"=10, "Reserved"=0, "DeviceID"=7, "Data type"=8208, "NTP time"=0} ("Header"), "Size of this messages"=w1001) -> (w1003:T19)
            n619 = Flatten To String(anything=w1003, prepend array or string size? (T)=FALSE) -> (data string=w1000:string)  [unwired: 2 in, 2 out]
            n620 = Concatenate Strings(w1000, w993) -> (w999:string)
            n621 = TCP Write(connection ID=w1009, data in=w999, 9:1000 ("timeout ms (25000)")) -> ()  [unwired: 1 in, 3 out]
          }
        }
        n622 = case shown="True" "get data" {
          tunnel: [w974 w988] -> w944
          tunnel: w946 -> [w974 w988]
          frame False {
          }
          frame True {
            n623 = Bundle By Name(cluster=T20 {"command id"=17, "Reserved"=0, "parameter idx"=0} ("Header"), "parameter idx"="parameter idx 2") -> (w984:T20)
            n624 = Flatten To String(anything=w984, prepend array or string size? (T)=FALSE, byte order (0:big-endian, network order)=T10."little-endian") -> (data string=w976:string)  [unwired: 1 in, 2 out]
            n625 = String Length(string=w976) -> (length=w981:i32)
            n626 = To Unsigned Long Integer(number=w981) -> (unsigned 32bit integer=w980:u32)
            n627 = Bundle By Name(cluster=T19 {"Magic word"=2952708290, "Size of prev messages"=0, "Size of this messages"=10, "Reserved"=0, "DeviceID"=7, "Data type"=8208, "NTP time"=0} ("Header"), "Size of this messages"=w980) -> (w982:T19)
            n628 = Flatten To String(anything=w982, prepend array or string size? (T)=FALSE) -> (data string=w979:string)  [unwired: 2 in, 2 out]
            n629 = Concatenate Strings(w979, w976) -> (w978:string)
            n630 = TCP Write(connection ID=w988, data in=w978, 9:1000 ("timeout ms (25000)")) -> ()  [unwired: 1 in, 3 out]
          }
        }
        n631 = case shown="True" "saveconfig" {
          tunnel: [w960 w972] -> w943
          tunnel: w944 -> [w960 w972]
          frame False {
          }
          frame True {
            n632 = Flatten To String(anything=cluster{"command id":u16, "Reserved":u16} {"command id"=4, "Reserved"=0} ("Header"), prepend array or string size? (T)=FALSE, byte order (0:big-endian, network order)=T10."little-endian") -> (data string=w963:string)  [unwired: 1 in, 2 out]
            n633 = String Length(string=w963) -> (length=w967:i32)
            n634 = To Unsigned Long Integer(number=w967) -> (unsigned 32bit integer=w966:u32)
            n635 = Bundle By Name(cluster=T19 {"Magic word"=2952708290, "Size of prev messages"=0, "Size of this messages"=10, "Reserved"=0, "DeviceID"=7, "Data type"=8208, "NTP time"=0} ("Header"), "Size of this messages"=w966) -> (w968:T19)
            n636 = Flatten To String(anything=w968, prepend array or string size? (T)=FALSE) -> (data string=w965:string)  [unwired: 2 in, 2 out]
            n637 = Concatenate Strings(w965, w963) -> (w964:string)
            n638 = TCP Write(connection ID=w972, data in=w964, 9:1000 ("timeout ms (25000)")) -> ()  [unwired: 1 in, 3 out]
          }
        }
      }
      n639 = Not Equal?(x=refnum<k5> refnum, y=w132) -> (x != y?=w131:bool)
      n640 = case shown="True" w131 {
        tunnel: w132 -> [_ w1172]
        frame False {
        }
        frame True {
          n641 = TCP Close Connection(connection ID=w1172) -> ()  [unwired: 2 in, 2 out]
        }
      }
    }
  }
